vi "Step Speed Caluculation.vi"() -> ()   [LabVIEW 2025]
uses:
  controls/LAB-IQ UI Data.ctl
  HEAVE vi's/Heave Write enum.ctl
  HEAVE vi's/Heave Right enum.ctl
  SWAY vi's/Sway Write enum.ctl
  SWAY vi's/Sway Right enum.ctl
  d081153b-36ca-4bc4-8478-749476f82ba4.vi
  1202965f-721d-4349-8d61-5de826f379ef.vi
  785ec975-e53d-4ed4-be48-2cc128d7a91f.vi
  02c5850b-52e8-4ed5-91f8-6f0ad62f4994.vi
  1223eb78-e4c4-4b69-bf80-185c82055158.vi
  e5651a45-6a49-4a3f-b503-ff1eaf449b4a.vi
  support/Message Queue/Enqueue Message (Single).vi
  <vilib>/Utility/error.llb/Error Cluster From Error Code.vi
  <vilib>/Utility/file.llb/Read Delimited Spreadsheet (string).vi
  <vilib>/Utility/file.llb/Write Delimited Spreadsheet (string).vi
  <vilib>/ErrorRing/Error Ring.xnode
  support/Message Queue/LAB-IQ Message Queue.lvlib
  support/User Event - Stop/LAB-IQ User Event - Stop.lvlib
panel:
  out "error out":errorcluster
  in  "File Path :  2":path
  out "Wear Track Diameter":dbl
  in  "Stribeck table":bool
  in  "seq":bool=TRUE
  out "Drive Error":string
  out "mm/s  Surge":dbl=7.0 caption="Jog" min=0.001 max=50.0 step=0.0001 format="%.2f"
  in  "Update Surge Speed":bool
  out "mm/s  Sway":dbl=7.0 caption="Jog" min=0.001 max=50.0 step=0.0001 format="%.2f"
  in  "Update Sway Speed":bool
  in  "Update Heave Speed":bool
  out "mm/s Heave":dbl=7.0 caption="Jog" min=0.001 max=30.0 step=0.0001 format="%.2f"
  in  "mm/sec":dbl=1.0 caption="Jog" min=0.001 max=50.0 step=0.001 format="%.2f"
  out "Scratch Start Test":bool
  in  "HomeScratch":bool
  in  "TEST SELECTION":enum32{"Time", "Cycle"}(radio)
  in  "Sway Loop Delay":dbl
  in  "Sway PID Speed":dbl=1.0 format="%.4f"
  in  "Sway Jog Speed":dbl=1.0 format="%.4f"
  out "HEAVE ENABLE":bool
  in  "SPARE  5":u8
  in  "Manual Write SWAY":bool
  out "SWAY WRITE":string
  in  "SPARE  4":u8
  in  "SPARE  3":u8
  in  "SPARE 2":u8
  in  "SPARE 1":u8
  out "Spare 15":u8
  out "Spare 14":u8
  out "Spare 13":u8
  out "Spare 12":u8
  out "Spare 11":u8
  out "Spare 10":u8
  out "Spare 9":u8
  out "Spare 8":u8
  out "Spare 7":u8
  out "Spare 6":u8
  out "Spare 5":u8
  out "Spare 4":u8
  out "Spare 3":u8
  out "Spare 2":u8
  out "Spare 1":u8
  out "Node Id":u8
  out "Read SWAY Temp":bool
  out "fwMinor":u8
  out "fwMajor":u8
  out "faultCode":u16
  out "Rotary POSE":sgl format="%#.6f"
  out "SWAY POSE":sgl format="%#.6f"
  out "Homed":u8
  out "State":u8
  out "Ack ID":u16
  in  "SPEED":sgl=10000.0
  in  "Distance":sgl=10000.0
  in  "Mode Command":u8=2
  out "Sequence ID":u16
  out "error out Read SWAY":errorcluster
  out "error out Write  SWAY":errorcluster
  out "SWAY READ":string
  in  "min_finetune_floor":dbl=0.15
  in  "min_deadband_floor":dbl=0.05
  in  "fine_tune_pct":dbl=100.0
  out "Start Test Temp":bool
  in  "STOP":bool
  in  "AppLoadSeq scratch":bool
  out "Pulse delta":dbl
  in  "Fine Tune Zone":dbl=10.0
  in  "PID Delay (sec)":dbl=1.0 format="%#_6p"
  in  "Max_pos_limit":dbl=50000000.0
  in  "Min_pos_limit":dbl
  in  "i_limit":dbl=10.0
  in  "Max Step Linit":dbl=10.0
  in  "Init Step":dbl=10.0
  in  "pct_scale":dbl=100.0
  in  "Deadband":dbl=0.1
  in  "Kd":dbl
  in  "Ki":dbl
  in  "Kp":dbl=1.0
  out "Current Position":dbl
  in  "Set Load":dbl
  in  "Current Load":dbl
  in  "Manual Write Heave & Surge":bool
  out "Heave and Surge Write":string
  in  "Heave Loop Delay":dbl
  in  "Heave PID Speed":dbl=15.0
  in  "Surge Jog Speed":dbl=1.0 format="%.4f"
  in  "Heave Jog Speed":dbl=15.0
  in  "SPARE 4":u8
  in  "SPARE 3":u8
  in  "SPARE 2":u8
  in  "SPARE 1":u8
  out "Spare 15":u8
  out "Spare 14":u8
  out "Spare 13":u8
  out "Spare 12":u8
  out "Spare 11":u8
  out "Spare 10":u8
  out "Spare 9":u8
  out "Spare 8":u8
  out "Spare 7":u8
  out "Spare 6":u8
  out "Spare 5":u8
  out "Spare 4":u8
  out "Spare 3":u8
  out "Spare 2":u8
  out "Spare 1":u8
  out "Node Id":u8
  out "Read Heave Temp":bool
  out "fwMinor":u8
  out "fwMajor":u8
  out "faultCode":u16
  out "SURGE POSE":sgl format="%#.6f"
  out "HEAVE POSE":sgl format="%#.6f"
  out "Homed":u8
  out "State":u8
  out "Ack ID":u16
  in  "SPEED":sgl=10000.0
  in  "Distance":sgl=10000.0
  in  "Mode Command":u8=2
  out "Sequence ID":u16
  out "error out Read":errorcluster
  out "error out Write":errorcluster
  out "Heave and Surge Read":string
  out "Load Cell Temp":bool
  in  "Stop Scratch":bool
  in  "Enter Fixed SRR 2":dbl min=0.0 max=0.0 format="%.3f"
  in  "E.Velocity 2":bool=TRUE caption="SRR"
  in  "Tab Control 3":T1(tab)
  in  "Tab Control 5":enum32{""}(tab)
  in  "Tab Control 14":T2(tab)=enum."Motor Load"
  in  "Ramp MulFac":dbl=2.0
  in  "pulses LoadDiffRamp(2..10)":dbl=9.0
  in  "PulseControlRamp(diff<=3N)":dbl=5.0 min=1.0 max=1000.0 step=1.0 format="%#.1f"
  in  "SetLoadDeadband(%) Load(0-10N)":dbl=0.1 min=0.0001 max=100.0 step=0.0001 format="%#.6f"
  in  "PID gains out delay (microForce)":T3={"proportional gain (Kc)"=300.0, "integral time (Ti, min)"=0.00011, "derivative time (Td, min)"=0.0} {"derivative time (Td, min)" format="%.3f"; "integral time (Ti, min)" min=1e-05 max=100.0 step=1e-06 format="%.6f"; "proportional gain (Kc)" format="%.3f"}
  in  "Ramp":bool
  in  "Gain 2":dbl=0.016
  in  "pulses LoadDiff(2..10)":dbl=10.0
  in  "pulses LoadDiff(11..50)":dbl=40.0
  in  "PulseControl(diff<=3N)":dbl=1.0 min=1.0 max=1000.0 step=1.0 format="%#.1f"
  out "SetLoadDeadband(%)  2":dbl=1.0 min=0.001 max=100.0 step=0.001 format="%#.6f"
  in  "Dummy Run":bool
  out "Vertical load (N)":dbl format="%#.3f"
  in  "AutoTune":bool
  in  "Offset  3":dbl=1.5
  in  "apply load":bool
  in  "Enter ByPass Load":dbl
  in  "reinit 3":bool=TRUE
  in  "output range delay":cluster{"output high":dbl, "output low":dbl}={"output high"=100.0, "output low"=-100.0} {"output low" format="%.2f"; "output high" format="%.2f"}
  in  "PID gains out delay":T3={"proportional gain (Kc)"=30.0, "integral time (Ti, min)"=0.00101, "derivative time (Td, min)"=0.0} {"derivative time (Td, min)" format="%.3f"; "integral time (Ti, min)" min=1e-05 max=100.0 step=0.0001 format="%.4f"; "proportional gain (Kc)" format="%.3f"}
  in  "Bypass Load":bool
  in  "pulsesSent":dbl=200.0
  out "pulses":dbl
  out "actpid":dbl
  out "gFF Rot 7":cluster{dbl, dbl, dbl}(graph)
  in  "pulses LoadDiff(21..1000)":dbl=40.0
  in  "Delay":dbl=1.5 min=0.001 max=5.0 step=0.001 format="%#.6f"
  in  "deadband":dbl=0.2
  in  "Tab Control 26":enum32{"Page 1", "Page 2"}(tab)
  in  "ClearAll":bool
  out "Mz(Nm)":dbl[](array[numeric])
  out "My(Nm)":dbl[](array[numeric])
  out "Mx(Nm)":dbl[](array[numeric])
  in  "Save Dwell":dbl=0.015 caption="Save Dwell (sec)" min=0.0 max=5.0 step=0.001 format="%.3f"
  out "Mx":dbl[](graph)
  out "My":dbl[](graph)
  out "Mz":dbl[](graph)
  out "Fy(N)":dbl[](graph)
  out "Fz(N)":dbl[](graph)
  in  "ZeroAll":bool
  in  "Acq Delay (ms)":dbl=10.0
  in  "Burst Delay (ms)":dbl=10.0
  out "model":string
  out "SN":i32
  out "FFx(N)":dbl[](array[numeric])
  in  "Sensor IP":string="192.168.1.100"
  in  "Port":i32=8080
  out "FFy(N)":dbl[](array[numeric])
  out "Load(N)":dbl[](array[numeric])
  out "Fx(N)":dbl[](graph)
  out "AE":bool
  in  "delete Handle":bool
  in  "Create Handle":bool=TRUE
  out "ft_data":dbl[](array[numeric])=[1.0, 1.0, 1.0, 1.0, 1.0, 1.0]
  out "ft_range":dbl[](array[numeric])=[1.0, 1.0, 1.0, 1.0, 1.0, 1.0]
  in  "stop 6":bool
  out "running_flag":bool
  out "ft_udp_handle":i32
  out "get-data-return":i32
  out "get-range-return":i32
  out "zero-return":i32
  out "filter-return":i32
  out "initial-return":i32
  out "deleteHandle-result":i32
  in  "Tab Control 19":enum32{"Platform COM", "Config ", "DevInfo"}(tab)=enum."Config "
  in  "SAMPLES":dbl=100.0
  in  "Re-initilaize":bool
  in  "Filter ON/OFF":bool=TRUE
  in  "TracHomeSurgeOffsetCounts 10MM":dbl=505100.0
  in  "TracHomeSwayOffsetCounts 10MM":dbl=1432.0
  in  "Acoustic Emission:":dbl=1.0 min=0.0001 max=200.0 step=0.0001 format="%.4f"
  in  "Apply Filter (FF)":bool
  in  "Filter% 2":dbl=50.0 min=50.0 max=100.0 step=0.1 format="%.1f"
  in  "Apply Filter (Load)":bool=TRUE
  in  "Filter%":dbl=80.0 min=50.0 max=100.0 step=0.1 format="%.1f"
  in  "Sway distance (mm)":dbl=245.0
  in  "Surge distance (mm)":dbl=370.0
  in  "DataSavingLoopDelay(ms)":dbl=15.0
  in  "SAVE  2":bool
  in  "Enter Distance":bool caption="Enter Counts"
  in  "Sway Counts:":dbl=100.0 min=0.0 max=100000000.0 step=1.0 format="%.2f"
  in  "Distance (mm): 3":dbl=100.0 caption="Distance (mm):" min=0.0 max=1500.0 step=0.001 format="%.5f"
  in  "Surge Counts:":dbl=100.0 min=0.0 max=100000000.0 step=1.0 format="%.1f"
  in  "Distance (mm): 2":dbl=100.0 caption="Distance (mm):" min=0.0 max=1500.0 step=0.0001 format="%.3f"
  in  "Distance (mm):":dbl=100.0 min=0.0 max=1500.0 step=0.001 format="%.5f"
  in  "Heave Counts:":dbl=100.0 min=0.0 max=100000000.0 step=1.0
  in  "LRMHomeSurgeOffsetCounts":dbl=307197.0
  in  "LRMHomeSwayOffsetCounts":dbl=26880.0
  in  "TracHomeSurgeOffsetCounts 20MM":dbl=505100.0
  in  "TracHomeSwayOffsetCounts 20MM":dbl=1432.0
  in  "RotHomeSwayOffsetCounts":dbl=14656.0
  in  "RotHomeSurgeOffsetCounts":dbl=311465.0
  in  "Heave distance":dbl=340.0
  out "Zmm":dbl=1600.0
  out "Heave Pulses/mm":dbl=1600.0
  out "Surge Pulses/mm":dbl=1600.0
  out "Sway Pulses/mm":dbl=320.0
  in  "Heave Pitch":dbl=4.0
  in  "Surge Pitch":dbl=3.0
  in  "Sway Pitch":dbl=2.0
  in  "Heave PPR":dbl=6400.0
  in  "Surge PPR":dbl=6400.0
  in  "Sway PPR":dbl=6400.0
  in  "GUI":T4(tab)
  in  "Platform Settings":bool caption="Password"
  in  "Configure":bool caption="Password"
  in  "Home":bool caption="Password"
  in  "EXIT":bool
  in  "Analysis":bool caption="Password"
  in  "service 2":bool caption="Password"
  in  "MainPage":T5(tab)=enum."HOME"
  in  "Select Load Head":bool
  in  "Notes :":string
  in  "FILE":string
  in  "Sample ID :":string
  in  "Operator ID :":string
  in  "Operator Name :":string
  in  "Auto":bool caption="Power Status"
  in  "Disable Axis Jog Soft Limits":bool
  out "Sway and Surge COM Status":bool=TRUE caption="Load COM Status"
  out "Heave COM Status":bool=TRUE caption="Load COM Status"
  in  "Enable Platform":bool
  in  "Surge Forward Main":bool
  in  "Surge Backward Main":bool
  in  "Sway Right Main":bool
  in  "Sway Left Main":bool
  in  "Heave Down Main":bool
  in  "Heave Up main":bool
  in  "mm":dbl=0.001 caption="Jog" min=0.001 max=200.0 step=0.0001 format="%#.3f"
  in  "Surface Analysis":bool
  in  "Imaging":bool
  in  "Image Analysis":bool
  in  "Post Analysis":bool
  in  "SSP 0.75":bool
  in  "SSP 0.5":bool
  in  "SSP 0.3":bool
  in  "Warning":enum32{"Page 2"}(tab)
  in  "gui GIF":enum32{"Check", "Deca", "kilo", "Micro"}(tab)
  out "Communication is established":bool=TRUE caption="Load COM Status"
  in  "Reference Sample":u16(ring) items=["None", "Brass", "Aluminium", "Mild Steel"]
  out "Load Cell Communication Slide":u8(slide)=1 min=1 max=10 step=1 scale=0.0..10.0
  in  "com 3":bool
  out "com":bool
  out "DecaForce COM Status":bool caption="Load COM Status"
  in  "Loading Mode":u16(ring) items=["Constant", "Ramp", "Steps", "Indentation"]
  in  "Enter the CoF Trip":dbl=1.0
  in  "Enter the Friction Force Trip":dbl=520.0 min=500.0 max=500.0 step=1.0 format="%#.1f"
  in  "Enter the Normal load Trip":dbl=520.0 min=500.0 max=500.0 step=0.001 format="%.3f"
  in  "KiloForce":bool
  in  "DecaForce":bool
  in  "MicroForce":bool
  in  "LHBack":bool
  in  "LHNext":bool
  in  "Load Selection":T6(tab)
  in  "Enter the Load  (N)":dbl=2.0 caption="Enter the Load (N)" min=200.0 max=500.0 step=0.1 format="%#.4f"
  in  "Enter the Final Load (N)":dbl=1.0 min=0.0 max=500.0 step=1.0 format="%#.0f"
  in  "Update":bool
  in  "Enter the Loading Rate (N/min)":dbl=60.0 min=1.0 max=1200.0 step=0.1 format="%.2f"
  out "Warning 2":bool
  in  "Stribeck Table  For loading":string[][](table)
  in  "Clear 3":bool
  out "Message":string="Load Entered is out of range!!!"
  in  "Indentation":string[][](table)=[["Detection", "5", "2"], ["Unload", "0", "5"], ["Load", "10", "2"], ["Unload", "0", "5"], ["Detection", "5", "2"], ["Unload", "0", "5"]]
  in  "Multipoint":bool caption="Singlepoint"
  in  "AppLoad 4":bool
  in  "zNL":bool
  out "NL disp":dbl caption="Normal Load ( N )" min=-2000.0 max=2000.0 step=0.0001 format="%.1f"
  in  "Traction":bool
  in  "Surge Forward MM":bool
  in  "Surge Backward MM":bool
  in  "M3 Image":enum32{"Page 1", "Page 2"}(tab)
  in  "String 39":string="Jog heave to bring the upper sample closer to the lower sample within 1mm."
  in  "Sway Left MM":bool
  in  "Sway Right MM":bool
  in  "Disable Axis Jog Soft Limits":bool
  in  "mm":dbl=0.001 caption="Jog" min=0.001 max=5.0 step=0.0001 format="%#.3f"
  in  "Heave Down MM":bool
  in  "Heave Up MM":bool
  in  "Wear Track Diameter (mm)":dbl=30.0 caption="Wear Track Diameter (mm):" min=1.0 max=30.0 step=1.0 format="%.2f"
  in  "Set WTD":bool
  in  "HomeScratch":bool
  in  "HomeRot":bool
  in  "PlaceModule":bool
  in  "Motion Mode:":u16(ring) items=["Uniform Rotation", "Angular Oscillation", "Stribeck ", "Steps"]
  in  "LR Sway":bool
  in  "Rot Hor":bool
  in  "Rot Ver":bool
  in  "Scratch":bool
  in  "LR Cam":bool
  in  "MMBack":bool
  in  "MMNext":bool
  in  "Rotary Module Selection":T7(tab)
  in  "SPEED SELECTION :":enum32{"Speed in RPM", "Speed in m/sec"}(radio)=enum."Speed in m/sec"
  in  "Enter the Speed(mm/sec)":dbl=0.1 min=0.1 max=10.0 step=0.1 format="%.3f"
  in  "Enter the Speed (RPM)":dbl=45.0 min=1.0 max=3000.0 step=1.0
  in  "Enter the Frequency (Hz)":dbl=1.0 min=0.1 max=10.0 step=0.1 format="%.1f"
  in  "Enter the Angle (Deg)":dbl=45.0 min=5.0 max=300.0 step=1.0
  in  "Angular Oscillation Set":bool
  in  "Rotary Tab":enum32{"Page 1", "Page 2"}(tab)
  out "e.v/ssr 2":enum32{"E.V", "SSR"}(tab)
  in  "Enter the Final E.Velocity (m/s) 2":dbl=1.0 min=0.001 max=4.0 step=0.001 format="%.3f"
  in  "Enter initial E.Velocity (m/s) 2":dbl=2.0 min=0.001 max=4.0 step=0.001 format="%.3f"
  in  "Enter Fixed E.Velocity 2":dbl=1.0 min=0.001 max=2.0 step=0.001 format="%.3f"
  in  "Enter Final SRR 2":dbl=1.0 min=0.001 max=1.0 step=0.001 format="%.2f"
  in  "Enter initial SRR 2":dbl=1.0 min=0.001 max=1.0 step=0.001 format="%.2f"
  out "Final Speed (RPM) 3":dbl=1.0 min=0.1 max=3000.0 step=0.1 format="%.1f"
  out "Initial Speed (RPM) 2":dbl=100.0 min=0.1 max=3000.0 step=0.1 format="%.1f"
  in  "Enter the Final Velocity (m/s) 3":dbl=1.0 min=0.001 max=2.0 step=0.001 format="%.3f"
  in  "Enter initial Velocity (m/s)  3":dbl=2.0 min=0.001 max=2.0 step=0.001 format="%.3f"
  out "Ramp Up 2":bool caption="Ramp Down"
  in  "Import 2":bool
  in  "Save 2":bool
  in  "SPEED SELECTION : rotary":enum32{"Speed in Rpm", "Speed in m/sec"}(radio)=enum."Speed in m/sec"
  in  "calculate rotary":bool
  in  "String 45":string="File Path Location : C:-->LAB-IQ 150 --> User Defined\n                                       Protocol-->File.txt"
  in  "Step Speed":enum32{"Step Speed", "Step (load-Speed)"}(tab)
  in  "StepTable For Speed":string[][](table)
  in  "StepTable For Load-Speed":string[][](table)=[["", "", ""], ["", "", ""], ["", "", ""], ["", "", ""]]
  in  "StepTable For Speed 3":string[][](table)=[["", "", ""], ["", "", ""], ["", "", ""], ["", "", ""]]
  in  "Motion Direction:  3":u16(ring) items=["Clockwise", "Counter Clockwise"]
  in  "Enter Scratch length (mm):":dbl=1.0 min=1.0 max=50.0 step=0.0001 format="%.4f"
  in  "Enter Scratch Speed (mm/s):":dbl=1.0 min=0.003 max=10.0 step=0.0031 format="%.5f"
  in  "SwaySpeed Set":bool
  in  "Scartch Offset":dbl=1.0 caption="Scratch Offset: (mm)" min=0.1 max=5.0 step=0.1 format="%.1f"
  in  "Motion type:":u16(ring) items=["Unidirection", "Bidirection"]
  in  "Scratch Mode:":u16(ring) items=["Scratch", "Pre-Post Scan", "Multi Pass"]
  in  "Rotary Speed Exced":string="Motor Speed Out of Range"
  out "Humidity  Status  3":bool caption="Communication Status"
  out "Low Temp  Status  2":bool=TRUE caption="Communication Status"
  out "TK4 status 2":bool=TRUE caption="Communication Status"
  in  "String 40":string="Before selecting Acoustic make sure the sensor output pin is connected to A4."
  in  "Stage Temperature":dbl[](array[numeric])=[150.0, 230.0, 300.0, 350.0, 400.0, 450.0, 500.0]
  in  "Sample Temperature":dbl[](array[numeric])=[100.0, 150.0, 200.0, 250.0, 300.0, 350.0, 400.0]
  in  "Humidity (Amb)":bool
  in  "Clear List":bool
  out "Sensors Picked":string
  in  "Add to list":bool
  in  "Wear":bool
  in  "Vibration":bool
  in  "Humidity (Chamber)":bool
  in  "Temperature (Chamber)":bool
  in  "ECR":bool
  in  "Temperature (Amb)":bool
  in  "Microphone":bool
  in  "Acoustic Emission 3":bool
  in  "SNext":bool
  in  "APBack":bool
  in  "Enter the Temperature (°C):":dbl
  in  "Enter the Stage \nTemperature (°C):":dbl=20.0 min=20.0 max=150.0 step=1.0 format="%#.0f"
  in  "Enter the Humidity (%Rh):":dbl=30.0 min=30.0 max=85.0 step=1.0
  in  "Low Temp":bool
  in  "High Temp":bool
  in  "Humidity":bool
  in  "Main Screen Tab":T8(tab)
  in  "ClrLog":bool
  out "Trip Log":string
  in  "Start Test":bool
  out "Test status":bool caption="Test Status"
  out "AR Led":bool caption="AR"
  out "Data":bool=TRUE
  out "Health":bool=TRUE
  out "Sway COM Status":bool=TRUE caption="Load COM Status"
  out "Heave COM Status":bool=TRUE caption="Load COM Status"
  in  "Grp Tab":enum32{"Rot/LRM", "FBT"}(tab)
  in  "Sub Graph":T9(tab)
  in  "Speed Reset Graph":bool
  in  "Speed Tab":enum32{" Rotary Disc", "MTM Ball", "MTM Disc"}(tab)
  out "speed mm/sec":dbl(graph)=0.13298760003255525
  out "MTM BALL SPEED":dbl(graph)=0.13298760003255525
  out "MTM DISC  SPEED":dbl(graph)=0.13298760003255525
  in  "Temperature Reset":bool
  out "Temperature (deg c)":dbl(graph)=0.13298760003255525
  in  "ECR RESET":bool
  out "ECR":dbl(graph)=0.13298760003255525
  out "Acoustic Emission (mV)":dbl min=0.0 max=5000.0 step=0.1
  in  "Aqucostic Reset Graph":bool
  out "gACQUOS":dbl(graph)=0.13298760003255525
  in  "Humidity Reset Graph":bool
  out "HumrGp":dbl(graph)=0.13298760003255525
  out "SD (mm)":dbl caption="Sliding Distance ( mm )" min=-200.0 max=200.0 step=0.1 format="%.4f"
  in  "Siliding distance Reset Graph":bool
  out "SDGp":dbl(graph)=0.13298760003255525
  out "Hymidity":bool
  in  "Humidity Disable trip":bool=TRUE
  in  "CoF Trip  2":dbl=540.0 min=100.0 max=540.0 step=1.0
  out "Depth Trip":dbl=600.0
  in  "Depth Trip":bool=TRUE
  out "Weart Deapth":bool
  in  "Depth Reset Graph":bool
  out "Weart":bool
  in  "Depthz":bool
  out "Depth (µm)":dbl min=-200.0 max=200.0 step=0.1 format="%.1f"
  out "WearGp":dbl(graph)=0.13298760003255525
  out "NL Trip 2":dbl=600.0
  out "Load pid":bool
  in  "Load Disable Trip":bool=TRUE
  in  "Load Reset Graph":bool
  out "NL Display 4":dbl caption="Normal Load ( N )" min=-2000.0 max=2000.0 step=0.0001 format="%.1f"
  out "Main Chart 3":cluster{dbl, "NL disp":dbl, dbl}(graph)
  in  "FF Tab":T10(tab)
  in  "COF Reset Graph":bool
  in  "COF Disable Trip":bool=TRUE
  out "COF TRIP":dbl=600.0
  out "Coefficient of Friction":dbl(graph)=0.13298760003255525
  in  "zFF":bool
  in  "FF Reset Graph":bool
  in  "FF Disable Trip":bool=TRUE
  out "FF TRIP":dbl=600.0
  out "Friction Force (N)":dbl min=-2000.0 max=2000.0 step=0.0001 format="%.3f"
  out "Friction Force (N) Graph":dbl(graph)=0.13298760003255525
  out "Cyclic FF TRIP":dbl=600.0
  in  "Cyclic FF Disable Trip":bool=TRUE
  in  "Cyclic FF Reset Graph":bool
  in  "CZ FF":bool
  out "Cyclic Friction Force (N) Graph":dbl(graph)=0.13298760003255525
  out "Cyclic Friction Force (N)":dbl min=-2000.0 max=2000.0 step=0.0001 format="%.3f"
  out "cyclic COF TRIP":dbl=600.0
  in  "cyclic COF Disable Trip":bool=TRUE
  in  "cyclic COF Reset Graph":bool
  out "Cyclic Coefficient of Friction":dbl(graph)=0.13298760003255525
  in  "BACK":bool
  out "Ambient \nTemperature":dbl min=0.0 max=5000.0 step=0.1 format="%.1f"
  out "Ambient\n Humidity":dbl min=0.0 max=5000.0 step=0.1 format="%.2f"
  out "NL disp 2":dbl caption="Normal Load ( N )" min=-2000.0 max=2000.0 step=0.0001 format="%.1f"
  out "Set Humidity":dbl caption="Set Humidity  (% Rh)" min=-2000.0 max=2000.0 step=1.0 format="%.1f"
  out "humidity disp":dbl caption="Humidity (% Rh)" min=-2000.0 max=2000.0 step=1.0 format="%.1f"
  in  "Humidity On":bool
  in  "zNL 2":bool
  out "NLt":bool
  in  "Load En":bool
  out "Freq (Hz)":dbl min=0.0 max=5000.0 step=0.1 format="%.4f"
  out "HumCOMStatus":bool caption="Communication Status"
  out "Load Communication":bool
  in  "Temp Tabs":enum32{"Low Temp", "High Temp"}(tab)=enum."High Temp"
  out "Controller  Status":bool
  out "ChamberTemp":dbl format="%#.1f"
  in  "SetTmp":dbl=-190.0 caption="Set Temperature (Deg C)" min=-190.0 max=100.0 step=1.0 format="%.1f"
  in  "Cooling":bool
  in  "Heater":bool
  out "TK4 status":bool caption="Controller  Status"
  out "ChamberTemp":dbl format="%#.1f"
  in  "SetTmp":dbl caption="Set Temperature (Deg C)" min=0.0 max=1000.0 step=1.0 format="%.1f"
  in  "Set Load (N)":dbl=100.0 min=0.01 max=1500.0 step=0.01 format="%.1f"
  in  "Time Tab":enum32{"cycles", "duration"}(tab)=enum."duration"
  out "Test Duration 4":dbl=600.0 caption="Test Duration\n(HH:MM:SS)" min=0.0083 max=180000.0 step=0.0001 format="%<%H:%M:%S>t"
  out "TEST CYCLE":dbl min=0.0 max=5000.0 step=0.01 format="%.2f"
  in  "TOTAL CYCLES":dbl min=0.0 max=5000.0 step=0.1 format="%.4f"
  out "Time ( HH:MM:SS ) 2":dbl min=0.0 max=144000.0 step=1.0 format="%<%H:%M:%S>t"
  in  "Test Duration":dbl=600.0 caption="Test Duration\n(HH:MM:SS)" min=0.0083 max=180000.0 step=0.0001 format="%<%H:%M:%S>t"
  in  "Main Speed Tab":enum32{"ROTARY", "TRACTION"}(tab)
  in  "SPEED TAB":enum32{"RPM", "m/sec"}(tab)
  out "Speed (RPM)":dbl min=0.0 max=5000.0 step=0.1 format="%.1f"
  out "Set Speed":dbl caption="Set Speed (RPM)" min=0.0 max=1500.0 step=0.1 format="%.1f"
  out "Speed (m/sec)":dbl min=0.0 max=5000.0 step=0.001 format="%.4f"
  out "Set Speed (m/sec)":dbl min=0.0 max=1500.0 step=0.001 format="%.4f"
  in  "MTM MOTOR DISPLAY":enum32{"MTM RPM", "MTM m/sec"}(tab)
  out "Disc Speed (RPM)":dbl min=0.0 max=1500.0 step=0.1 format="%.1f"
  out "Ball Speed (RPM)":dbl min=0.0 max=1500.0 step=0.1 format="%.1f"
  out "Disc Speed (m/sec)":dbl min=0.0 max=1500.0 step=0.1 format="%.1f"
  out "Ball Speed (m/sec)":dbl min=0.0 max=1500.0 step=0.1 format="%.1f"
  in  "Angle and Frequency":enum32{"angular", "lrm"}(tab)
  out "Angle (Deg)":dbl min=0.0 max=5000.0 step=0.01 format="%.2f"
  out "Stroke (mm)":dbl min=0.0 max=5000.0 step=0.01 format="%.2f"
  in  "Analysis Home":bool
  in  "Password":string
  in  "Home Service":bool
  in  "Advanced Setting":bool
  in  "About Tab":enum32{"Primary"}(tab)
  in  "ECR Port:":refnum<visa-resource-name>="COM10"
  in  "Ramp Port:":refnum<visa-resource-name>="COM10"
  in  "Installation/Replacement completed":bool
  in  "Loahead":bool
  in  "Heave and Surge COM Port:":refnum<visa-resource-name>="COM9"
  in  "Sway COM Port:":refnum<visa-resource-name>="COM10"
  in  "Temp Modbus:":refnum<visa-resource-name>="COM14"
  in  "Humidity Port:":refnum<visa-resource-name>="COM10"
  in  "Edit Gain Constants":bool
  in  "Save Gain Constants":bool
  in  "Service About":bool
  # "SET JOG SPEED"
  # "Speed Exceed the limit of the Motor"
  # "Motor Speed Out of Range"
  # "load Aquisition off"
  # "load Aquisition On"
  # "Configuration"
  # "Limits for Heave Surge and Sway"
  # "Modules Offset Parameters"
  # "Counts-Distance Calculator"
  # "File Name :"
  # "Ensure the traction module is aligned\n horizontally with the stage before ENABLE."
  # "JOG MODE"
  # "Module Selection"
  # "Positioning Control"
  # "Connect the controller\ncable to M3"
  # "Environment"
  # "Sensors"
  # "Data Points"
  # "Data Points"
  # "Data Points"
  # "Data Points"
  # "ohms"
  # "Data Points"
  # "Data Points"
  # "Data Points"
  # "LAB-IQ 150 / UNITEST / WO2456 / UT150  v05 / AUGUST 2025"
  # "NOTE: This operation needs to be done only when the machine is ON."
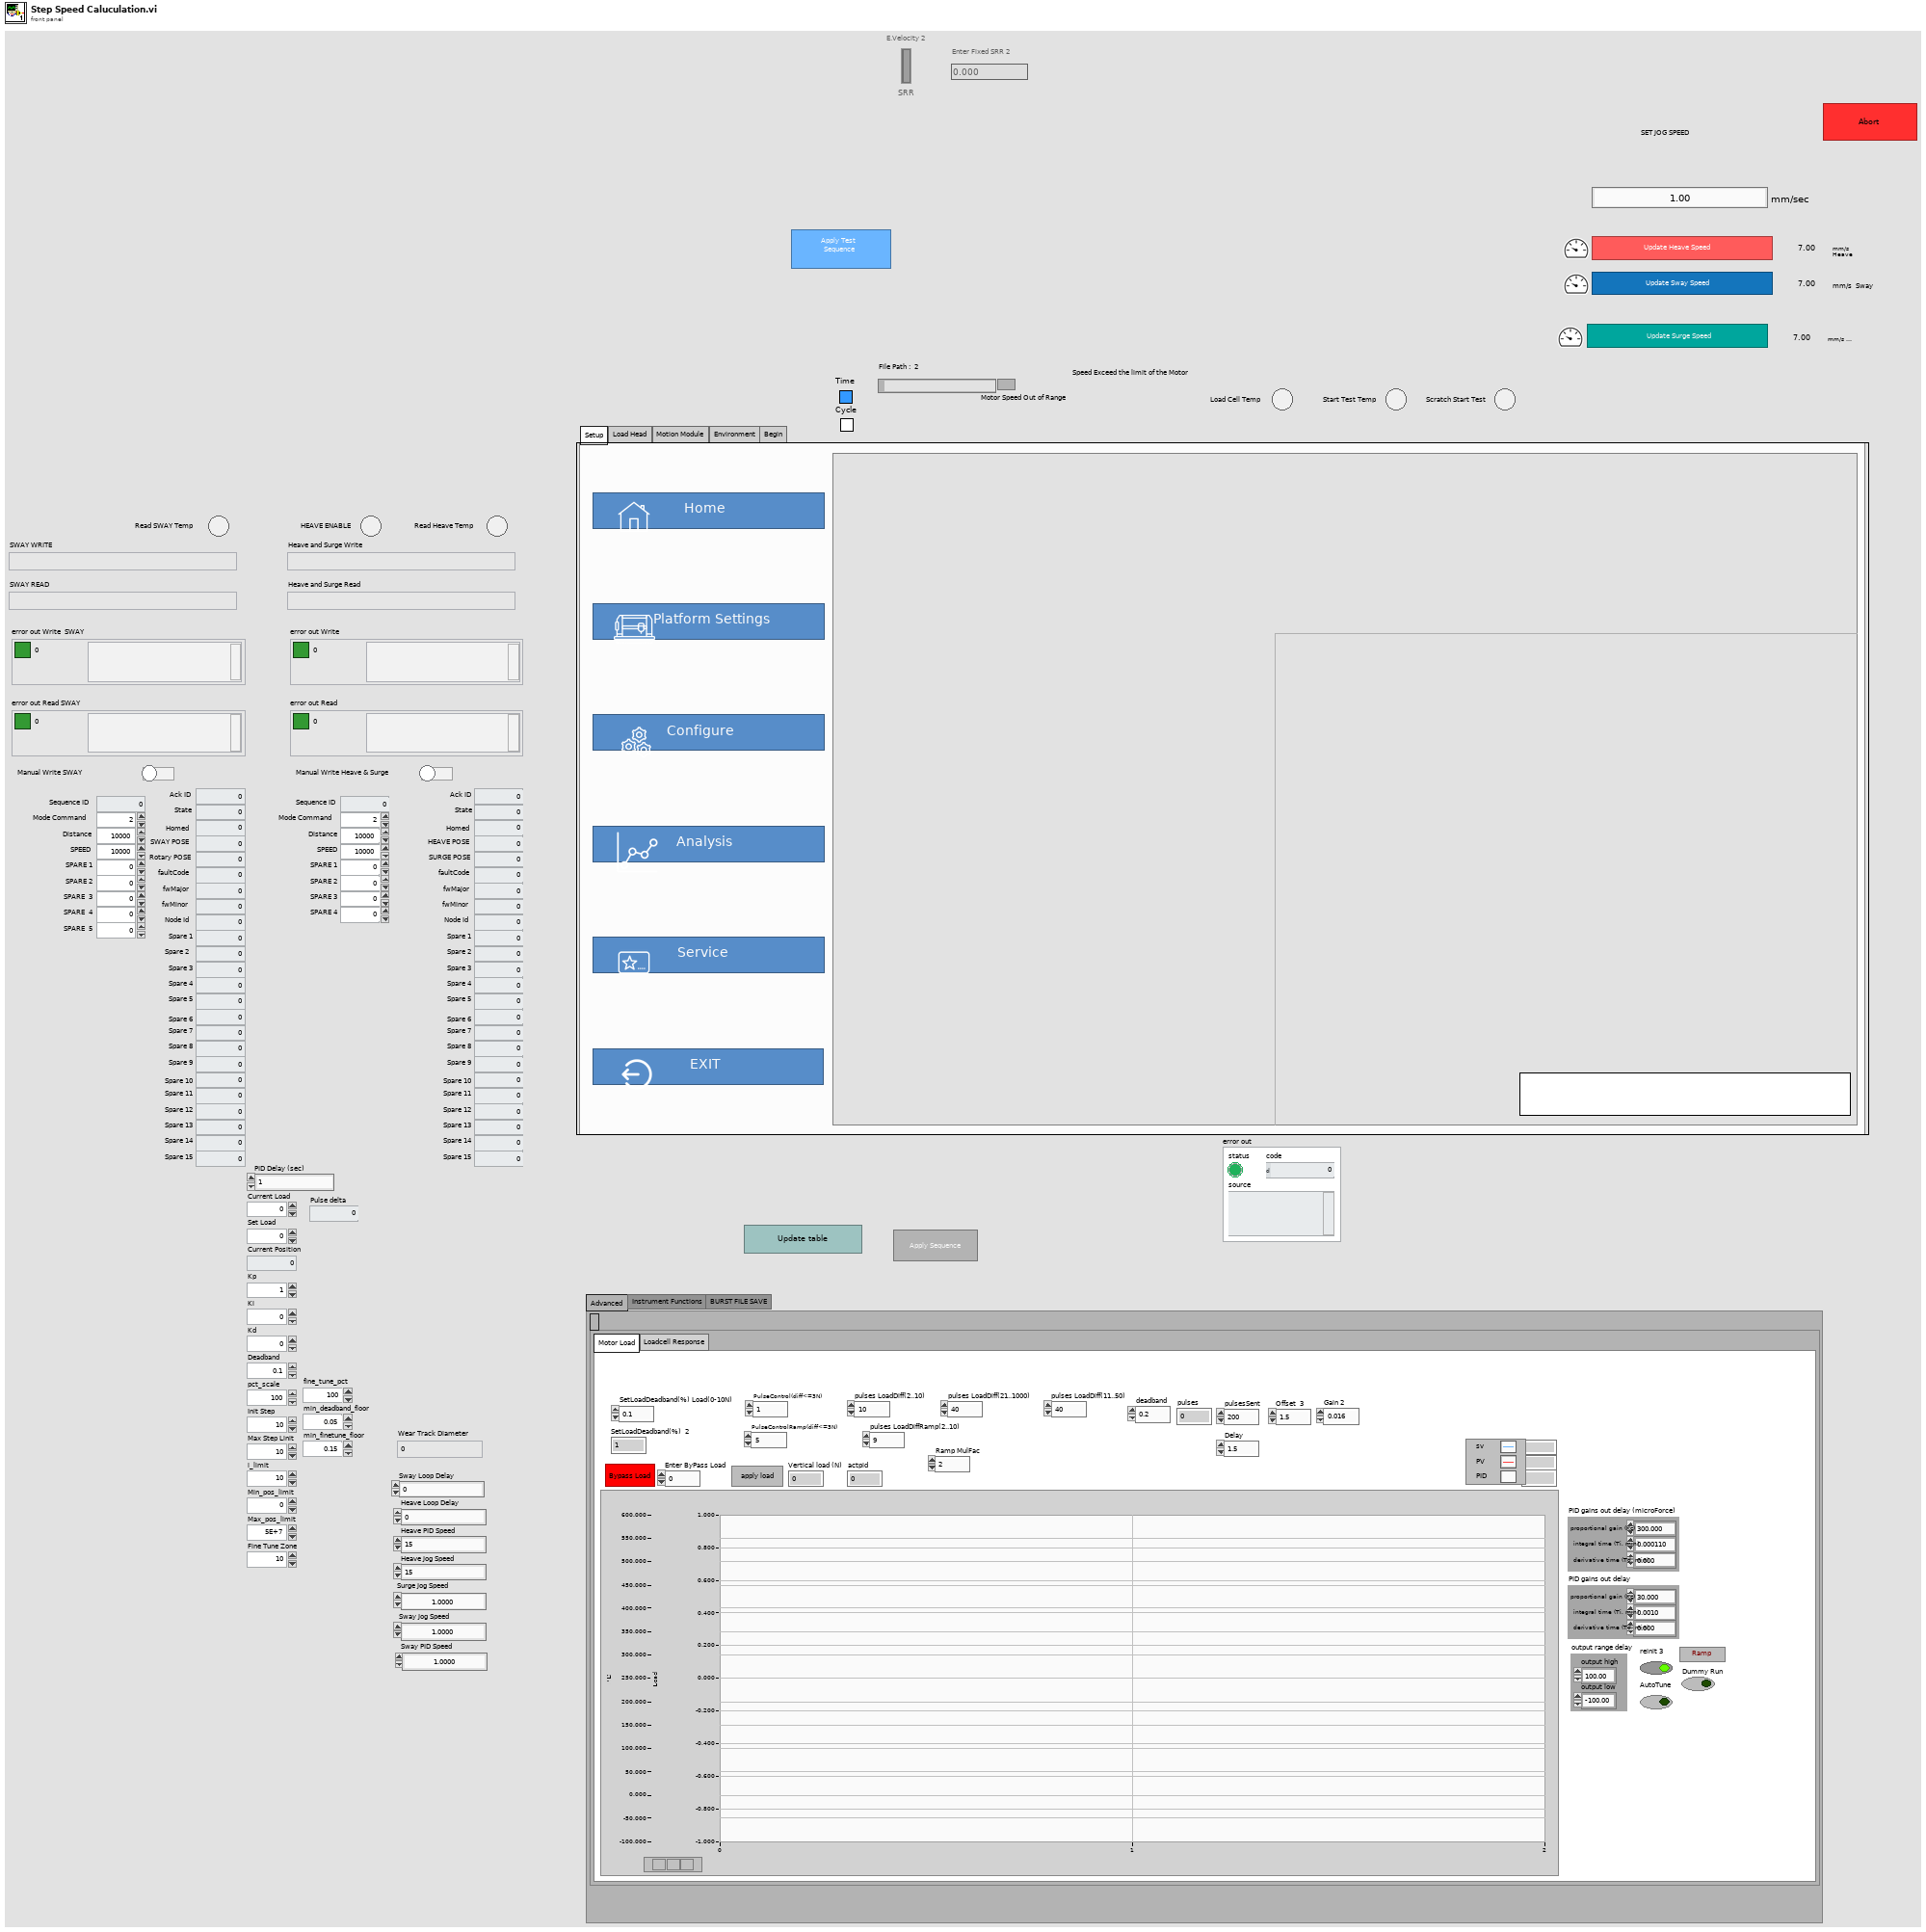
[diagram p1: front panel]
types:
  T1 = enum32{"Advanced", "Motor", "Depth_graph", "UIO Communicator", "Add to list parametrs", "Instrument Functions", "BURST FILE SAVE"}
  T2 = enum32{"LRM heating", "FBT_Heating", "Motor Load", "Loadcell Response", "Voice Load", "Step loading and speed ", "Depth"}
  T3 = cluster{"proportional gain (Kc)":dbl, "integral time (Ti, min)":dbl, "derivative time (Td, min)":dbl}
  T4 = enum32{"Setup", "Load Head", "Motion Module", "Environment", "Begin"}
  T5 = enum32{"Details", "PlatformSetting", "Analysis", "HOME"}
  T6 = enum32{"Constant", "Ramp", "Step", "Indentation"}
  T7 = enum32{"Uniform Rotation", "Angular Oscillation", "Speed Ramp", "Speed Step"}
  T8 = enum32{"  Acquire  ", "Compare Files Rot", "About", "Service"}
  T9 = enum32{"Speed", "Temperature", "ECR", "Acoustic Emission", "Humidity", "Sliding Distance"}
  T10 = enum32{"Coefficient of Friction ", "Friction Force (N)", "Cyclic Friction Force (N)", "Cyclic Coefficient of Friction "}
  T11 = typedef "LAB-IQ UI Data.ctl" = cluster{"Main Home Screen":cluster{"GUI":refnum<vi>, "Platform Settings":refnum<vi>, "Configure":refnum<vi>, "Home":refnum<vi>, "EXIT":refnum<vi>, "service 2":refnum<vi>, "MainPage":refnum<vi>, "Analysis":refnum<vi>}, "Platform Settings":cluster{"mm/s  Surge":refnum<vi>, "Update Surge Speed":refnum<vi>, "Drive Error":refnum<vi>, "Disable Axis Jog Soft Limits":refnum<vi>, "mm/s  Sway":refnum<vi>, "Sway and Surge COM Status":refnum<vi>, "Heave COM Status":refnum<vi>, "Enable Platform":refnum<vi>, "Surge Forward Main":refnum<vi>, "Sway Right Main":refnum<vi>, "Sway Left Main":refnum<vi>, "Heave Down Main":refnum<vi>, "Heave Up main":refnum<vi>, "Update Sway Speed":refnum<vi>, "Update Heave Speed":refnum<vi>, "mm/s Heave":refnum<vi>, "mm/sec":refnum<vi>, "mm":refnum<vi>, "Surge Backward Main":refnum<vi>}, "Analysis Screen":cluster{"Analysis Home":refnum<vi>, "Surface Analysis":refnum<vi>, "Imaging":refnum<vi>, "Image Analysis":refnum<vi>, "Post Analysis":refnum<vi>}, "Config Screen":cluster{"Select Load Head":refnum<vi>, "Notes :":refnum<vi>, "FILE":refnum<vi>, "Sample ID :":refnum<vi>, "Operator ID :":refnum<vi>, "Operator Name :":refnum<vi>, "Auto":refnum<vi>}, "Motion Module":cluster{"zNL":refnum<vi>, "NL disp":refnum<vi>, "Rotary Tab":refnum<vi>, "Motion Direction:  3":refnum<vi>, "E.Velocity 2":refnum<vi>, "e.v/ssr 2":refnum<vi>, "Enter Fixed E.Velocity 2":refnum<vi>, "Enter Final SRR 2":refnum<vi>, "Enter initial SRR 2":refnum<vi>, "Enter Fixed SRR 2":refnum<vi>, "Enter the Final E.Velocity (m/s) 2":refnum<vi>, "Enter initial E.Velocity (m/s) 2":refnum<vi>, "Final Speed (RPM) 3":refnum<vi>, "Initial Speed (RPM) 2":refnum<vi>, "Enter the Final Velocity (m/s) 3":refnum<vi>, "Enter initial Velocity (m/s)  3":refnum<vi>, "Ramp Up 2":refnum<vi>, "TEST SELECTION":refnum<vi>, "SPEED SELECTION : ":refnum<vi>, "Angular Oscillation Set":refnum<vi>, "Traction":refnum<vi>, "Step Speed":refnum<vi>, "StepTable For Load-Speed":refnum<vi>, "StepTable For Speed":refnum<vi>, "Surge Forward MM":refnum<vi>, "Surge Backward MM":refnum<vi>, "M3 Image":refnum<vi>, "String 39":refnum<vi>, "Sway Left MM":refnum<vi>, "Sway Right MM":refnum<vi>, "Disable Axis Jog Soft Limits":refnum<vi>, "mm":refnum<vi>, "Heave Down MM":refnum<vi>, "Heave Up MM":refnum<vi>, "Wear Track Diameter (mm)":refnum<vi>, "Set WTD":refnum<vi>, "HomeScratch":refnum<vi>, "HomeRot":refnum<vi>, "PlaceModule":refnum<vi>, "Enter the Angle (Deg)":refnum<vi>, "Enter the Frequency (Hz)":refnum<vi>, "Motion Mode:":refnum<vi>, "LR Sway":refnum<vi>, "Rot Hor":refnum<vi>, "Scratch":refnum<vi>, "LR Cam":refnum<vi>, "MMBack":refnum<vi>, "MMNext":refnum<vi>, "Rot Ver":refnum<vi>, "Rotary Module Selection":refnum<vi>, "calculate rotary":refnum<vi>, "SPEED SELECTION : rotary":refnum<vi>, "Import 2":refnum<vi>, "Save 2":refnum<vi>, "File Path :  2":refnum<vi>, "String 45":refnum<vi>, "StepTable For Speed 3":refnum<vi>, "Enter the Speed(mm/sec)":refnum<vi>, "Enter the Speed(RPM)":refnum<vi>, "Enter Scratch Speed (mm/s):":refnum<vi>, "SwaySpeed Set":refnum<vi>, "Scartch Offset":refnum<vi>, "Scratch Mode:":refnum<vi>, "Motion type:":refnum<vi>, "HomeScratch 2":refnum<vi>, "Enter Scratch length (mm):":refnum<vi>, "Wear Track Diameter":refnum<vi>, "Rotary Speed Exced":refnum<vi>}, "Environmental control":cluster{"Humidity  Status  3":refnum<vi>, "Low Temp  Status  2":refnum<vi>, "TK4 status 2":refnum<vi>, "Stage Temperature":refnum<vi>, "Sample Temperature":refnum<vi>, "Humidity (Amb)":refnum<vi>, "Clear List":refnum<vi>, "Add to list":refnum<vi>, "Wear":refnum<vi>, "Vibration":refnum<vi>, "Humidity (Chamber)":refnum<vi>, "Temperature (Chamber)":refnum<vi>, "ECR ":refnum<vi>, "Temperature (Amb)":refnum<vi>, "Microphone":refnum<vi>, "Acoustic Emission 3":refnum<vi>, "SNext":refnum<vi>, "APBack":refnum<vi>, "Enter the Temperature (°C):":refnum<vi>, "Enter the Stage \nTemperature (°C):":refnum<vi>, "Enter the Humidity (%Rh):":refnum<vi>, "Low Temp":refnum<vi>, "High Temp":refnum<vi>, "Humidity":refnum<vi>, "Sensors Picked":refnum<vi>}, "About Screen":cluster{"Password":refnum<vi>, "Home Service":refnum<vi>, "Advanced Setting":refnum<vi>, "About Tab":refnum<vi>, "ECR Port:":refnum<vi>, "Ramp Port:":refnum<vi>, "Installation/Replacement completed":refnum<vi>, "Loahead":refnum<vi>, "Heave and Surge COM Port:":refnum<vi>, "Sway COM Port:":refnum<vi>, "Temp Modbus:":refnum<vi>, "Humidity Port:":refnum<vi>, "Edit Gain Constants":refnum<vi>, "Save Gain Constants":refnum<vi>}, "Main Screen":cluster{"Main Screen Tab":refnum<vi>, "Angle and Frequency":refnum<vi>, "Stroke (mm)":refnum<vi>, "Angle (Deg)":refnum<vi>, "Main Speed Tab":refnum<vi>, "MTM MOTOR DISPLAY":refnum<vi>, "Disc Speed (m/sec)":refnum<vi>, "Ball Speed (m/sec)":refnum<vi>, "Disc Speed (RPM)":refnum<vi>, "Ball Speed (RPM)":refnum<vi>, "SPEED TAB":refnum<vi>, "Speed (m/sec)":refnum<vi>, "Set Speed (m/sec)":refnum<vi>, "Speed (RPM)":refnum<vi>, "Set Speed":refnum<vi>, "Time Tab":refnum<vi>, "Time ( HH:MM:SS ) 2":refnum<vi>, "Test Duration":refnum<vi>, "Test Duration 4":refnum<vi>, "TEST CYCLE":refnum<vi>, "TOTAL CYCLES":refnum<vi>, "Set Load (N)":refnum<vi>, "Temp Tabs":refnum<vi>, "Heater":refnum<vi>, "TK4 status":refnum<vi>, "ChamberTemp":refnum<vi>, "SetTmp":refnum<vi>, "Controller  Status":refnum<vi>, "ChamberTemp 2":refnum<vi>, "SetTmp 2":refnum<vi>, "Controller  Status 2":refnum<vi>, "ChamberTemp 3":refnum<vi>, "SetTmp 3":refnum<vi>, "Cooling":refnum<vi>, "Load Communication":refnum<vi>, "Ambient \nTemperature":refnum<vi>, "HumCOMStatus":refnum<vi>, "Ambient\n Humidity":refnum<vi>, "Freq (Hz)":refnum<vi>, "Load En":refnum<vi>, "NLt":refnum<vi>, "zNL 2":refnum<vi>, "Humidity On":refnum<vi>, "humidity disp":refnum<vi>, "Set Humidity":refnum<vi>, "NL disp 2":refnum<vi>, "Humidity On 2":refnum<vi>, "humidity disp 2":refnum<vi>, "Set Humidity 2":refnum<vi>, "NL disp 3":refnum<vi>, "AppLoadSeq scratch":refnum<vi>, "Stop Scratch":refnum<vi>, "ClrLog":refnum<vi>, "Trip Log":refnum<vi>, "STOP":refnum<vi>, "Start Test":refnum<vi>, "Test status":refnum<vi>, "AR Led":refnum<vi>, "Data":refnum<vi>, "Health":refnum<vi>, "Sway COM Status":refnum<vi>, "Heave COM Status":refnum<vi>, "Grp Tab":refnum<vi>, "Sub Graph":refnum<vi>, "SD (mm)":refnum<vi>, "Siliding distance Reset Graph":refnum<vi>, "SDGp":refnum<vi>, "Humidity Reset Graph":refnum<vi>, "HumrGp":refnum<vi>, "Acoustic Emission (mV)":refnum<vi>, "Aqucostic Reset Graph":refnum<vi>, "gACQUOS":refnum<vi>, "ECR RESET":refnum<vi>, "ECR":refnum<vi>, "Temperature Reset":refnum<vi>, "Acoustic Emission (mV) 2":refnum<vi>, "Aqucostic Reset Graph 2":refnum<vi>, "gACQUOS 2":refnum<vi>, "ECR RESET 2":refnum<vi>, "ECR 2":refnum<vi>, "Temperature Reset 2":refnum<vi>, "Temperature (deg c)":refnum<vi>, "Speed Reset Graph":refnum<vi>, "Speed Tab":refnum<vi>, "MTM DISC  SPEED":refnum<vi>, "MTM BALL SPEED":refnum<vi>, "speed mm/sec":refnum<vi>, "Hymidity":refnum<vi>, "Humidity Disable trip":refnum<vi>, "CoF Trip  2":refnum<vi>, "Depth Trip":refnum<vi>, "Weart Deapth":refnum<vi>, "Depth Reset Graph":refnum<vi>, "Weart":refnum<vi>, "Depthz":refnum<vi>, "Depth (µm)":refnum<vi>, "WearGp":refnum<vi>, "NL Trip 2":refnum<vi>, "Load pid":refnum<vi>, "Load Disable Trip":refnum<vi>, "Load Reset Graph":refnum<vi>, "NL Display 4":refnum<vi>, "Main Chart 3":refnum<vi>, "BACK":refnum<vi>, "Depth Trip 2":refnum<vi>, "COF TRIP ":refnum<vi>, "Friction Force (N)":refnum<vi>, "FF Reset Graph":refnum<vi>, "FF Disable Trip":refnum<vi>, "FF TRIP":refnum<vi>, "COF Disable Trip":refnum<vi>, "COF Reset Graph":refnum<vi>, "Start Test Temp":refnum<vi>, "zFF":refnum<vi>, "Friction Force (N) Graph":refnum<vi>, "Coefficient of Friction":refnum<vi>, "Scratch Start Test":refnum<vi>, "FF Tab":refnum<vi>, "Cyclic Friction Force (N)":refnum<vi>, "CZ FF":refnum<vi>, "Cyclic Friction Force (N) Graph":refnum<vi>, "Cyclic Coefficient of Friction":refnum<vi>, "Cyclic FF TRIP":refnum<vi>, "Cyclic FF Disable Trip":refnum<vi>, "cyclic COF Disable Trip":refnum<vi>, "cyclic COF TRIP":refnum<vi>, "cyclic COF Reset Graph":refnum<vi>, "Cyclic FF Reset Graph":refnum<vi>}, "Loading":cluster{"Indentation":refnum<vi>, "Reference Sample":refnum<vi>, "Load Cell Communication Slide":refnum<vi>, "com 3":refnum<vi>, "com":refnum<vi>, "DecaForce COM Status":refnum<vi>, "Update":refnum<vi>, "Clear 3":refnum<vi>, "seq":refnum<vi>, "Stribeck table":refnum<vi>, "Stribeck Table  For loading":refnum<vi>, "Loading Mode":refnum<vi>, "Enter the Final Load (N)":refnum<vi>, "Enter the CoF Trip":refnum<vi>, "Enter the Friction Force Trip":refnum<vi>, "Enter the Normal load Trip":refnum<vi>, "Enter the Load  (N)":refnum<vi>, "KiloForce":refnum<vi>, "DecaForce ":refnum<vi>, "MicroForce":refnum<vi>, "LHBack":refnum<vi>, "LHNext":refnum<vi>, "Enter the Loading Rate (N/min)":refnum<vi>, "Message":refnum<vi>, "Warning 2":refnum<vi>, "SSP 0.75":refnum<vi>, "SSP 0.5":refnum<vi>, "SSP 0.3":refnum<vi>, "Warning":refnum<vi>, "gui GIF":refnum<vi>, "Communication is established":refnum<vi>, "AppLoad 4":refnum<vi>, "Multipoint":refnum<vi>, "Load Selection":refnum<vi>}, "PID":cluster{"Ramp MulFac":refnum<vi>, "pulses LoadDiffRamp(2..10)":refnum<vi>, "PulseControlRamp(diff<=3N)":refnum<vi>, "SetLoadDeadband(%) Load(0-10N)":refnum<vi>, "PID gains out delay (microForce)":refnum<vi>, "Ramp":refnum<vi>, "Gain 2":refnum<vi>, "pulses LoadDiff(2..10)":refnum<vi>, "pulses LoadDiff(11..50)":refnum<vi>, "PulseControl(diff<=3N)":refnum<vi>, "SetLoadDeadband(%)  2":refnum<vi>, "Dummy Run":refnum<vi>, "Vertical load (N)":refnum<vi>, "AutoTune":refnum<vi>, "Offset 3 ":refnum<vi>, "apply load":refnum<vi>, "Offset  3":refnum<vi>, "apply load 2":refnum<vi>, "Enter ByPass Load":refnum<vi>, "reinit 3":refnum<vi>, "output range delay":refnum<vi>, "PID gains out delay":refnum<vi>, "Bypass Load":refnum<vi>, "pulsesSent":refnum<vi>, "pulses ":refnum<vi>, "actpid":refnum<vi>, "gFF Rot":refnum<vi>, "pulses LoadDiff(21..1000)":refnum<vi>, "Delay":refnum<vi>, "deadband":refnum<vi>}, "Config Parameters":cluster{"Tab Control 3":refnum<vi>, "Tab Control 19":refnum<vi>, "SAMPLES":refnum<vi>, "Re-initilaize":refnum<vi>, "Filter ON/OFF":refnum<vi>, "TracHomeSurgeOffsetCounts 10MM":refnum<vi>, "TracHomeSwayOffsetCounts 10MM":refnum<vi>, "Acoustic Emission:":refnum<vi>, "Apply Filter (FF)":refnum<vi>, "Filter% 2":refnum<vi>, "Apply Filter (Load)":refnum<vi>, "Filter% ":refnum<vi>, "Sway distance (mm)":refnum<vi>, "Surge distance (mm)":refnum<vi>, "DataSavingLoopDelay(ms)":refnum<vi>, "SAVE 2":refnum<vi>, "Enter Distance":refnum<vi>, "Sway Counts:":refnum<vi>, "Distance (mm): 3":refnum<vi>, "Surge Counts:":refnum<vi>, "Distance (mm): 2":refnum<vi>, "Distance (mm):":refnum<vi>, "Heave Counts:":refnum<vi>, "LRMHomeSurgeOffsetCounts":refnum<vi>, "LRMHomeSwayOffsetCounts":refnum<vi>, "TracHomeSurgeOffsetCounts 20MM":refnum<vi>, "TracHomeSwayOffsetCounts 20MM":refnum<vi>, "RotHomeSwayOffsetCounts":refnum<vi>, "RotHomeSurgeOffsetCounts":refnum<vi>, "Heave distance":refnum<vi>, "Zmm":refnum<vi>, "Heave Pulses/mm":refnum<vi>, "Surge Pulses/mm":refnum<vi>, "Sway Pulses/mm":refnum<vi>, "Heave Pitch":refnum<vi>, "Surge Pitch":refnum<vi>, "Sway Pitch":refnum<vi>, "Heave PPR":refnum<vi>, "Surge PPR":refnum<vi>, "Sway PPR":refnum<vi>, "Tab Control 5":refnum<vi>, "Tab Control 14":refnum<vi>, "Tab Control 26":refnum<vi>, "AE":refnum<vi>, "Heave Loop Delay":refnum<vi>, "Heave PID Speed":refnum<vi>, "Surge Jog Speed":refnum<vi>, "Heave Jog Speed":refnum<vi>, "Sway Loop Delay":refnum<vi>, "Sway PID Speed":refnum<vi>, "Sway Jog Speed":refnum<vi>}, "Loading Com Port":cluster{"ClearAll":refnum<vi>, "Mz(Nm)":refnum<vi>, "My(Nm)":refnum<vi>, "Mx(Nm)":refnum<vi>, "Save Dwell":refnum<vi>, "Mx ":refnum<vi>, "My ":refnum<vi>, "Mz":refnum<vi>, "Fx(N)":refnum<vi>, "Fy(N)":refnum<vi>, "Fz(N)":refnum<vi>, "ZeroAll":refnum<vi>, "Acq Delay (ms)":refnum<vi>, "Burst Delay (ms)":refnum<vi>, "model":refnum<vi>, "SN":refnum<vi>, "FFx(N)":refnum<vi>, "Sensor IP":refnum<vi>, "Port":refnum<vi>, "FFy(N)":refnum<vi>, "Load(N)":refnum<vi>, "delete Handle":refnum<vi>, "Create Handle":refnum<vi>, "ft_data":refnum<vi>, "ft_range":refnum<vi>, "ft_data 2":refnum<vi>, "stop 6":refnum<vi>, "running_flag":refnum<vi>, "ft_udp_handle":refnum<vi>, "get-data-return":refnum<vi>, "get-range-return":refnum<vi>, "zero-return":refnum<vi>, "filter-return":refnum<vi>, "initial-return":refnum<vi>, "deleteHandle-result":refnum<vi>, "Load Cell Temp":refnum<vi>}, "Heave AND Surge":cluster{"SURGE POSE":refnum<vi>, "error out Read":refnum<vi>, "HEAVE POSE":refnum<vi>, "State":refnum<vi>, "Homed":refnum<vi>, "Sequence ID":refnum<vi>, "error out Write":refnum<vi>, "faultCode":refnum<vi>, "Ack ID":refnum<vi>, "SPEED":refnum<vi>, "Distance":refnum<vi>, "Mode Command":refnum<vi>, "Heave and Surge Read":refnum<vi>, "Read Heave Temp":refnum<vi>, "Spare 15":refnum<vi>, "Spare 14":refnum<vi>, "Spare 13":refnum<vi>, "Spare 12":refnum<vi>, "Spare 11":refnum<vi>, "Spare 10":refnum<vi>, "Spare 9":refnum<vi>, "Spare 8":refnum<vi>, "Spare 7":refnum<vi>, "Spare 6":refnum<vi>, "Spare 5":refnum<vi>, "Spare 4":refnum<vi>, "Spare 2":refnum<vi>, "Spare 1":refnum<vi>, "Node Id":refnum<vi>, "Spare 3":refnum<vi>, "SPARE 4":refnum<vi>, "SPARE 3":refnum<vi>, "SPARE 2":refnum<vi>, "SPARE 1":refnum<vi>, "fwMajor":refnum<vi>, "fwMinor":refnum<vi>, "Manual Write":refnum<vi>, "Heave and Surge Write":refnum<vi>}, "New PID LOGIC":cluster{"Fine Tune Zone":refnum<vi>, "PID SDelay":refnum<vi>, "Max_pos_limit":refnum<vi>, "Min_pos_limit":refnum<vi>, "i_limit":refnum<vi>, "pct_scale":refnum<vi>, "Deadband":refnum<vi>, "Kd":refnum<vi>, "Ki":refnum<vi>, "Kp":refnum<vi>, "Current Position":refnum<vi>, "Set Load":refnum<vi>, "Current Load":refnum<vi>, "Pulse delta":refnum<vi>, "Init Step":refnum<vi>, "Max Step Linit":refnum<vi>}, "SWAY ":cluster{"fwMajor":refnum<vi>, "Homed":refnum<vi>, "Rotary POSE":refnum<vi>, "State":refnum<vi>, "SWAY POSE":refnum<vi>, "Ack ID":refnum<vi>, "faultCode":refnum<vi>, "Node Id":refnum<vi>, "fwMinor":refnum<vi>, "Spare 6":refnum<vi>, "Spare 5":refnum<vi>, "Spare 4":refnum<vi>, "Spare 3":refnum<vi>, "Spare 2":refnum<vi>, "Spare 1":refnum<vi>, "Spare 7":refnum<vi>, "SPARE  5":refnum<vi>, "error out Write  SWAY ":refnum<vi>, "error out Read SWAY ":refnum<vi>, "Manual Write SWAY ":refnum<vi>, "SWAY WRITE":refnum<vi>, "SPARE  4":refnum<vi>, "SPARE  3":refnum<vi>, "SPARE 2":refnum<vi>, "SPARE 1":refnum<vi>, "Spare 15":refnum<vi>, "Spare 14":refnum<vi>, "Spare 13":refnum<vi>, "Spare 12":refnum<vi>, "Spare 11":refnum<vi>, "Spare 9":refnum<vi>, "Spare 8":refnum<vi>, "SPEED":refnum<vi>, "Distance":refnum<vi>, "Mode Command":refnum<vi>, "Sequence ID":refnum<vi>, "SWAY READ":refnum<vi>, "Spare 10":refnum<vi>, "Read SWAY Temp":refnum<vi>}}
  T12 = typedef "init queue out loop.ctl" = cluster{"UI Loop":refnum<queue>, "LOAD COM LOOP ":refnum<queue>, "SWAY MOTOR COM LOOP":refnum<queue>, "HEAVE MOTOR COM LOOP":refnum<queue>, "TEMPERATURE COM LOOP":refnum<queue>, "RAMP MOTOR COM LOOP":refnum<queue>, "ECR PORT":refnum<queue>, "HUMIDITY COM PORT":refnum<queue>, "PROGRAM LOOP":refnum<queue>, "MONITOR LOOP":refnum<queue>, "REPORT":refnum<queue>, "LOAD PID":refnum<queue>}
  T13 = enum8{"Enabled", "Disabled", "Disabled and Grayed Out"}
  T14 = enum16{"INIT", "SETLOWPASSFILTER", "SETZERO", "GETSENSORINFO", "GETRANGE", "ZEROALL", "READDATA", "UNINITIAL", "DELETEHANDLE"}
  T15 = typedef "Heave Write enum.ctl" = enum16{"INIT", "WRITE", "CLOSE", "REINIT"}
  T16 = typedef "Sway Write enum.ctl" = enum16{"INIT", "WRITE", "CLOSE", "REINIT"}
  T17 = typedef "Sway Right enum.ctl" = enum16{"INIT", "READ", "CLOSE", "REINIT", ""}
  T18 = typedef "Heave Right enum.ctl" = enum16{"INIT", "READ", "CLOSE", "REINIT", ""}
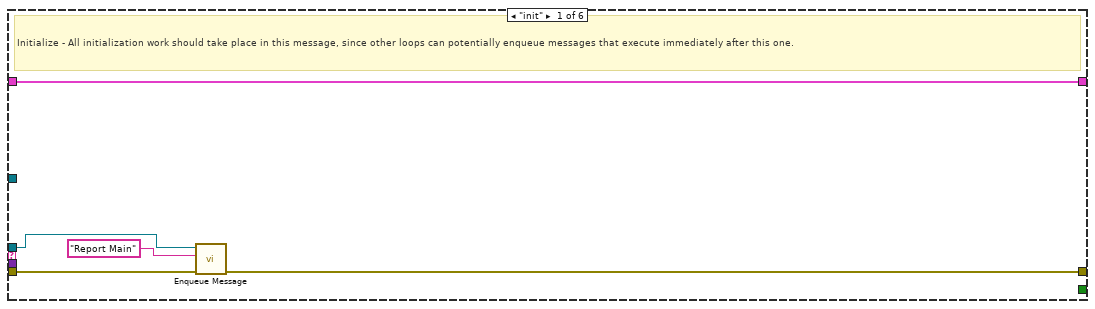
[diagram p2: hidden frame]
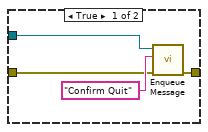
[diagram p3: hidden frame]
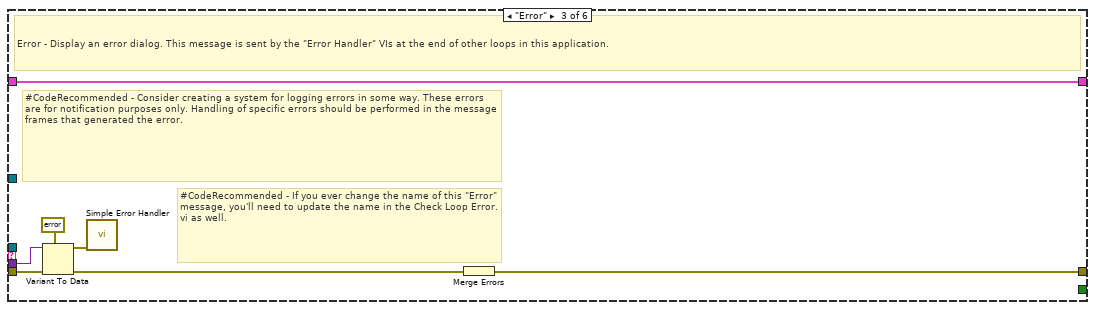
[diagram p4: hidden frame]
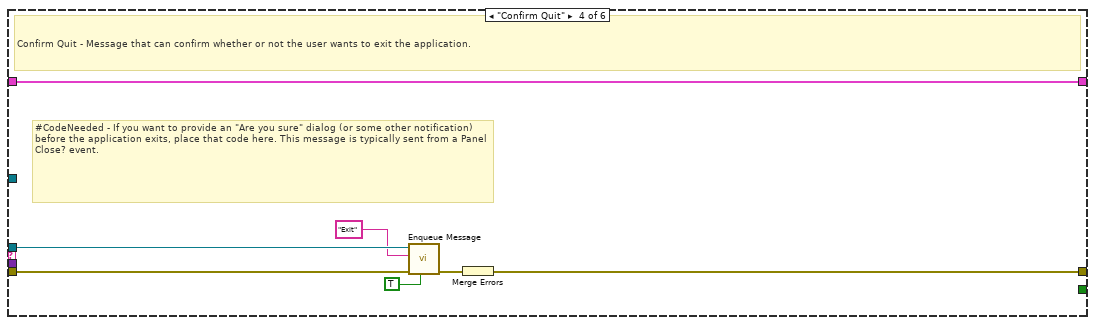
[diagram p5: hidden frame]
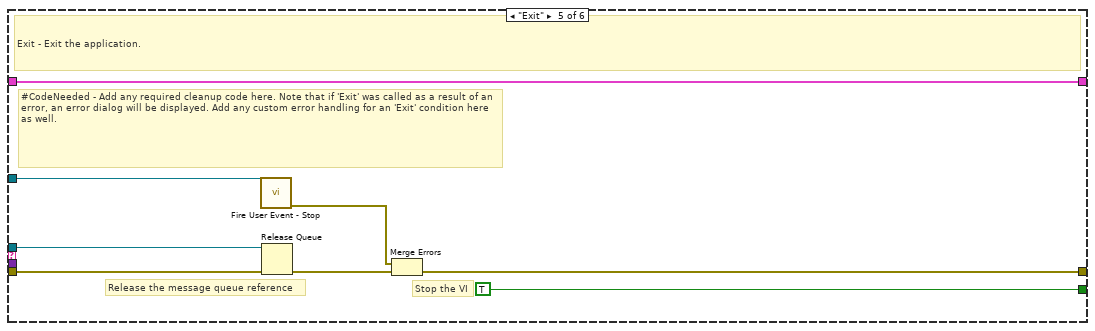
[diagram p6: hidden frame]
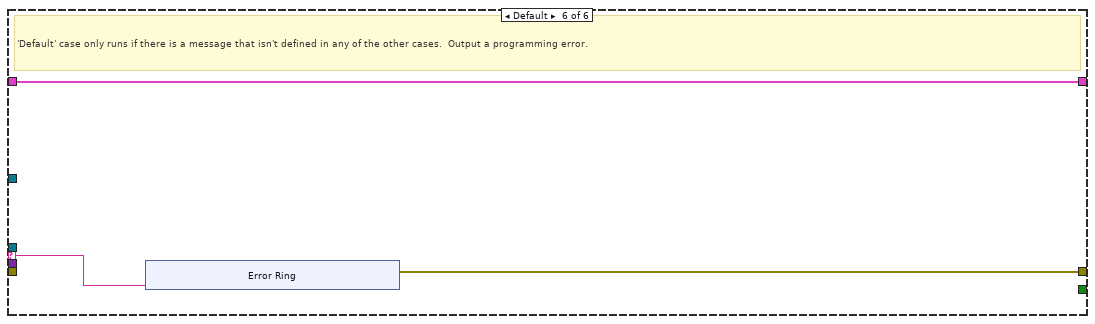
[diagram p7: hidden frame]
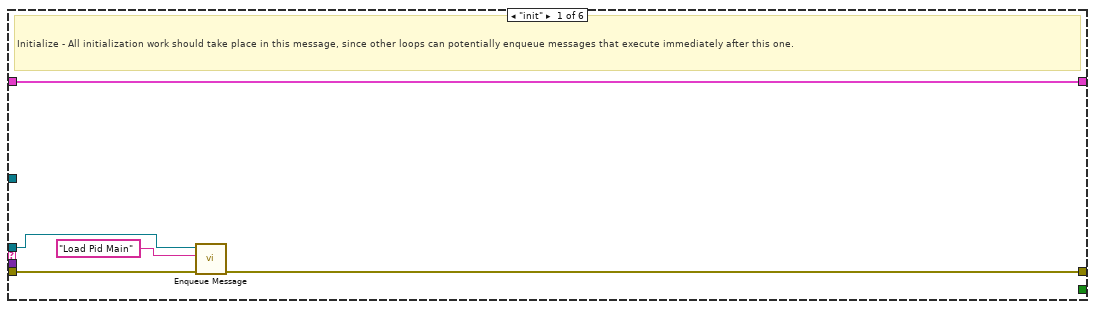
[diagram p8: hidden frame]
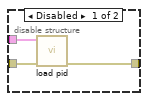
[diagram p10: hidden frame]
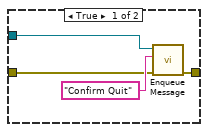
[diagram p11: hidden frame]
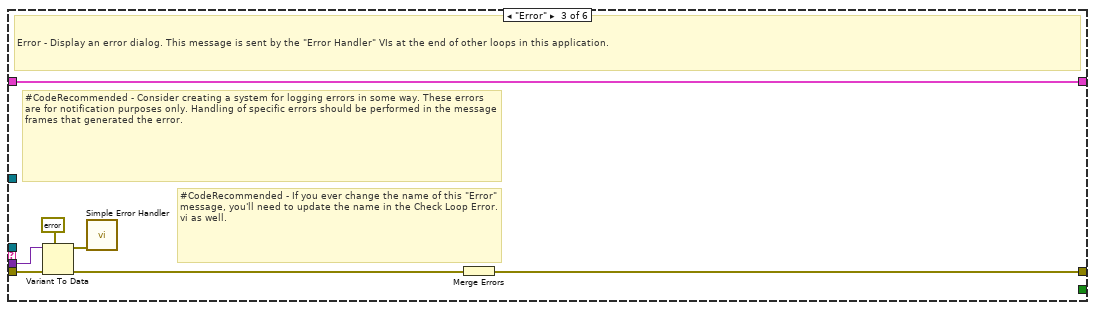
[diagram p12: hidden frame]
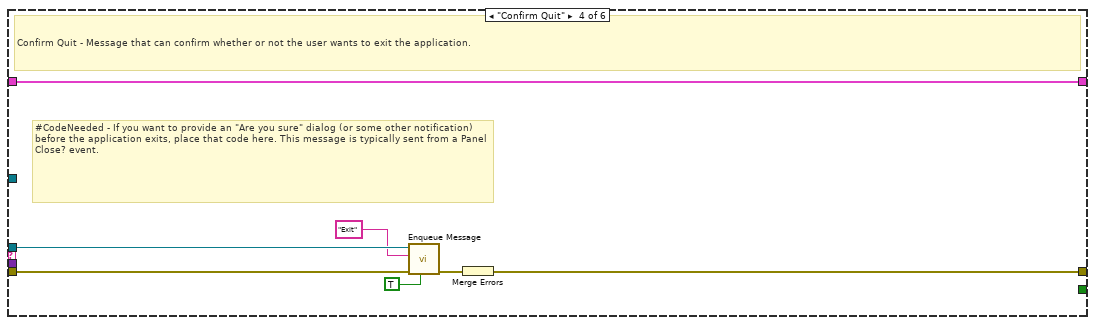
[diagram p13: hidden frame]
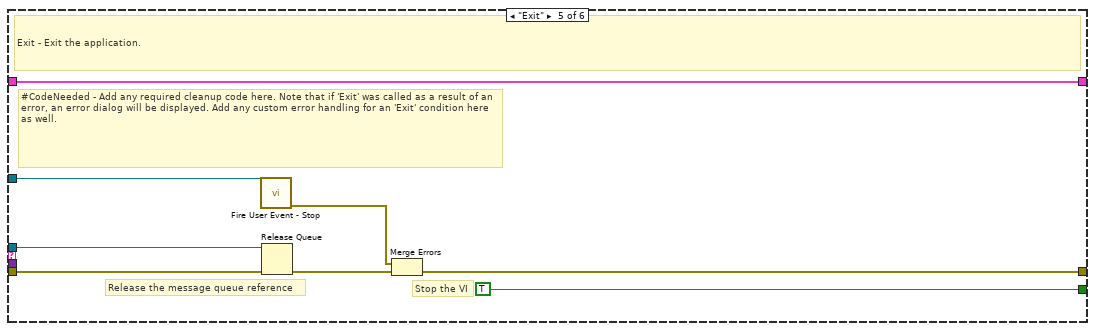
[diagram p14: hidden frame]
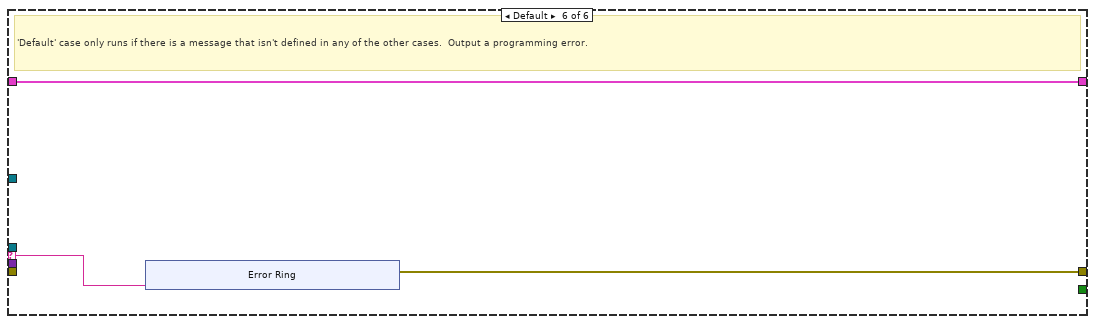
[diagram p15: hidden frame]
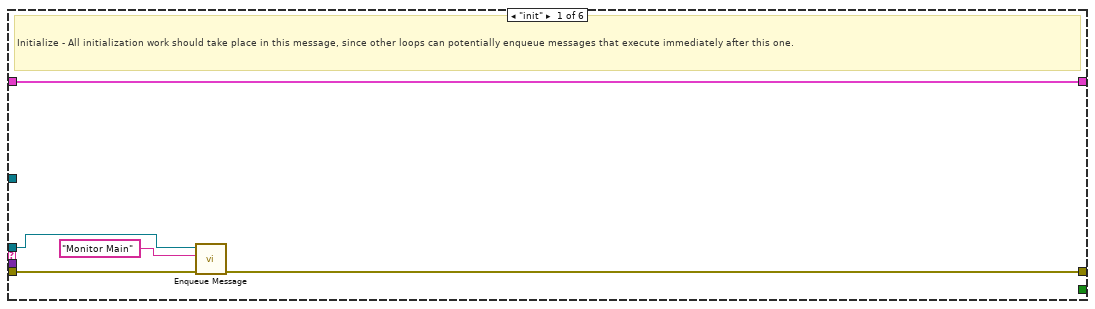
[diagram p16: hidden frame]
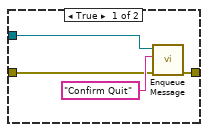
[diagram p17: hidden frame]
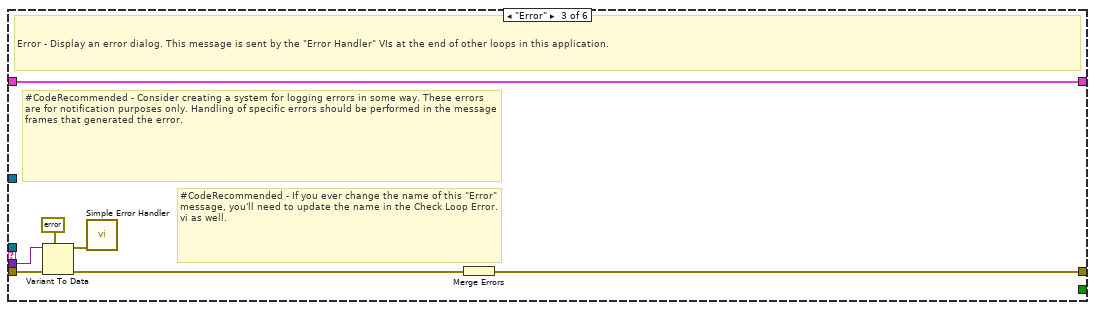
[diagram p18: hidden frame]
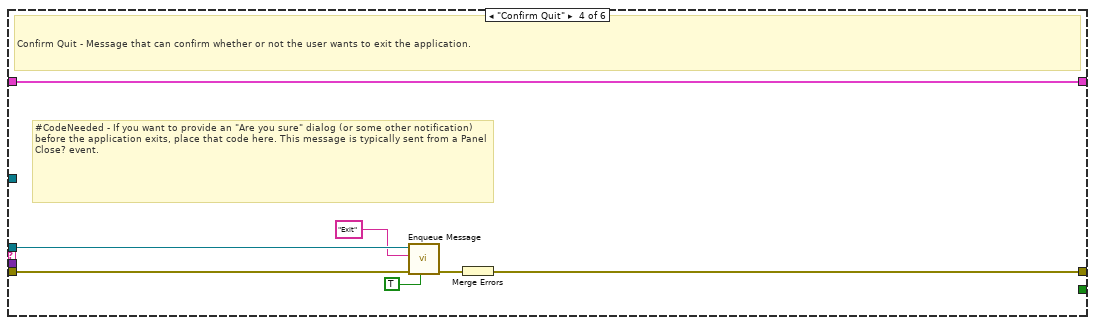
[diagram p19: hidden frame]
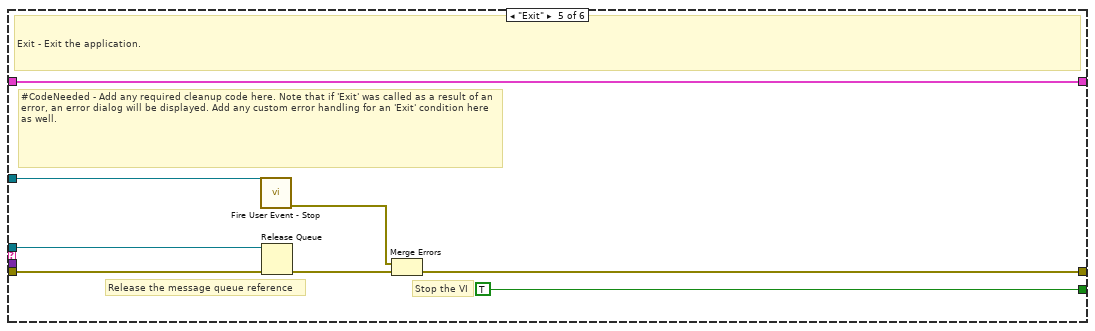
[diagram p20: hidden frame]
diagram:
  # "Select Load Head"
  n1 = flat-sequence {
    tunnel: [w55] -> w42
    tunnel: T11 {"Main Home Screen"={"GUI"=refnum, "Platform Settings"=refnum, "Configure"=refnum, "Home"=refnum, "EXIT"=refnum, "service 2"=refnum, "MainPage"=refnum, "Analysis"=refnum}, "Platform Settings"={"mm/s  Surge"=refnum, "Update Surge Speed"=refnum, "Drive Error"=refnum, "Disable Axis Jog Soft Limits"=refnum, "mm/s  Sway"=refnum, "Sway and Surge COM Status"=refnum, "Heave COM Status"=refnum, "Enable Platform"=refnum, "Surge Forward Main"=refnum, "Sway Right Main"=refnum, "Sway Left Main"=refnum, "Heave Down Main"=refnum, "Heave Up main"=refnum, "Update Sway Speed"=refnum, "Update Heave Speed"=refnum, "mm/s Heave"=refnum, "mm/sec"=refnum, "mm"=refnum, "Surge Backward Main"=refnum}, "Analysis Screen"={"Analysis Home"=refnum, "Surface Analysis"=refnum, "Imaging"=refnum, "Image Analysis"=refnum, "Post Analysis"=refnum}, "Config Screen"={"Select Load Head"=refnum, "Notes :"=refnum, "FILE"=refnum, "Sample ID :"=refnum, "Operator ID :"=refnum, "Operator Name :"=refnum, "Auto"=refnum}, "Motion Module"={"zNL"=refnum, "NL disp"=refnum, "Rotary Tab"=refnum, "Motion Direction:  3"=refnum, "E.Velocity 2"=refnum, "e.v/ssr 2"=refnum, "Enter Fixed E.Velocity 2"=refnum, "Enter Final SRR 2"=refnum, "Enter initial SRR 2"=refnum, "Enter Fixed SRR 2"=refnum, "Enter the Final E.Velocity (m/s) 2"=refnum, "Enter initial E.Velocity (m/s) 2"=refnum, "Final Speed (RPM) 3"=refnum, "Initial Speed (RPM) 2"=refnum, "Enter the Final Velocity (m/s) 3"=refnum, "Enter initial Velocity (m/s)  3"=refnum, "Ramp Up 2"=refnum, "TEST SELECTION"=refnum, "SPEED SELECTION : "=refnum, "Angular Oscillation Set"=refnum, "Traction"=refnum, "Step Speed"=refnum, "StepTable For Load-Speed"=refnum, "StepTable For Speed"=refnum, "Surge Forward MM"=refnum, "Surge Backward MM"=refnum, "M3 Image"=refnum, "String 39"=refnum, "Sway Left MM"=refnum, "Sway Right MM"=refnum, "Disable Axis Jog Soft Limits"=refnum, "mm"=refnum, "Heave Down MM"=refnum, "Heave Up MM"=refnum, "Wear Track Diameter (mm)"=refnum, "Set WTD"=refnum, "HomeScratch"=refnum, "HomeRot"=refnum, "PlaceModule"=refnum, "Enter the Angle (Deg)"=refnum, "Enter the Frequency (Hz)"=refnum, "Motion Mode:"=refnum, "LR Sway"=refnum, "Rot Hor"=refnum, "Scratch"=refnum, "LR Cam"=refnum, "MMBack"=refnum, "MMNext"=refnum, "Rot Ver"=refnum, "Rotary Module Selection"=refnum, "calculate rotary"=refnum, "SPEED SELECTION : rotary"=refnum, "Import 2"=refnum, "Save 2"=refnum, "File Path :  2"=refnum, "String 45"=refnum, "StepTable For Speed 3"=refnum, "Enter the Speed(mm/sec)"=refnum, "Enter the Speed(RPM)"=refnum, "Enter Scratch Speed (mm/s):"=refnum, "SwaySpeed Set"=refnum, "Scartch Offset"=refnum, "Scratch Mode:"=refnum, "Motion type:"=refnum, "HomeScratch 2"=refnum, "Enter Scratch length (mm):"=refnum, "Wear Track Diameter"=refnum, "Rotary Speed Exced"=refnum}, "Environmental control"={"Humidity  Status  3"=refnum, "Low Temp  Status  2"=refnum, "TK4 status 2"=refnum, "Stage Temperature"=refnum, "Sample Temperature"=refnum, "Humidity (Amb)"=refnum, "Clear List"=refnum, "Add to list"=refnum, "Wear"=refnum, "Vibration"=refnum, "Humidity (Chamber)"=refnum, "Temperature (Chamber)"=refnum, "ECR "=refnum, "Temperature (Amb)"=refnum, "Microphone"=refnum, "Acoustic Emission 3"=refnum, "SNext"=refnum, "APBack"=refnum, "Enter the Temperature (°C):"=refnum, "Enter the Stage \nTemperature (°C):"=refnum, "Enter the Humidity (%Rh):"=refnum, "Low Temp"=refnum, "High Temp"=refnum, "Humidity"=refnum, "Sensors Picked"=refnum}, "About Screen"={"Password"=refnum, "Home Service"=refnum, "Advanced Setting"=refnum, "About Tab"=refnum, "ECR Port:"=refnum, "Ramp Port:"=refnum, "Installation/Replacement completed"=refnum, "Loahead"=refnum, "Heave and Surge COM Port:"=refnum, "Sway COM Port:"=refnum, "Temp Modbus:"=refnum, "Humidity Port:"=refnum, "Edit Gain Constants"=refnum, "Save Gain Constants"=refnum}, "Main Screen"={"Main Screen Tab"=refnum, "Angle and Frequency"=refnum, "Stroke (mm)"=refnum, "Angle (Deg)"=refnum, "Main Speed Tab"=refnum, "MTM MOTOR DISPLAY"=refnum, "Disc Speed (m/sec)"=refnum, "Ball Speed (m/sec)"=refnum, "Disc Speed (RPM)"=refnum, "Ball Speed (RPM)"=refnum, "SPEED TAB"=refnum, "Speed (m/sec)"=refnum, "Set Speed (m/sec)"=refnum, "Speed (RPM)"=refnum, "Set Speed"=refnum, "Time Tab"=refnum, "Time ( HH:MM:SS ) 2"=refnum, "Test Duration"=refnum, "Test Duration 4"=refnum, "TEST CYCLE"=refnum, "TOTAL CYCLES"=refnum, "Set Load (N)"=refnum, "Temp Tabs"=refnum, "Heater"=refnum, "TK4 status"=refnum, "ChamberTemp"=refnum, "SetTmp"=refnum, "Controller  Status"=refnum, "ChamberTemp 2"=refnum, "SetTmp 2"=refnum, "Controller  Status 2"=refnum, "ChamberTemp 3"=refnum, "SetTmp 3"=refnum, "Cooling"=refnum, "Load Communication"=refnum, "Ambient \nTemperature"=refnum, "HumCOMStatus"=refnum, "Ambient\n Humidity"=refnum, "Freq (Hz)"=refnum, "Load En"=refnum, "NLt"=refnum, "zNL 2"=refnum, "Humidity On"=refnum, "humidity disp"=refnum, "Set Humidity"=refnum, "NL disp 2"=refnum, "Humidity On 2"=refnum, "humidity disp 2"=refnum, "Set Humidity 2"=refnum, "NL disp 3"=refnum, "AppLoadSeq scratch"=refnum, "Stop Scratch"=refnum, "ClrLog"=refnum, "Trip Log"=refnum, "STOP"=refnum, "Start Test"=refnum, "Test status"=refnum, "AR Led"=refnum, "Data"=refnum, "Health"=refnum, "Sway COM Status"=refnum, "Heave COM Status"=refnum, "Grp Tab"=refnum, "Sub Graph"=refnum, "SD (mm)"=refnum, "Siliding distance Reset Graph"=refnum, "SDGp"=refnum, "Humidity Reset Graph"=refnum, "HumrGp"=refnum, "Acoustic Emission (mV)"=refnum, "Aqucostic Reset Graph"=refnum, "gACQUOS"=refnum, "ECR RESET"=refnum, "ECR"=refnum, "Temperature Reset"=refnum, "Acoustic Emission (mV) 2"=refnum, "Aqucostic Reset Graph 2"=refnum, "gACQUOS 2"=refnum, "ECR RESET 2"=refnum, "ECR 2"=refnum, "Temperature Reset 2"=refnum, "Temperature (deg c)"=refnum, "Speed Reset Graph"=refnum, "Speed Tab"=refnum, "MTM DISC  SPEED"=refnum, "MTM BALL SPEED"=refnum, "speed mm/sec"=refnum, "Hymidity"=refnum, "Humidity Disable trip"=refnum, "CoF Trip  2"=refnum, "Depth Trip"=refnum, "Weart Deapth"=refnum, "Depth Reset Graph"=refnum, "Weart"=refnum, "Depthz"=refnum, "Depth (µm)"=refnum, "WearGp"=refnum, "NL Trip 2"=refnum, "Load pid"=refnum, "Load Disable Trip"=refnum, "Load Reset Graph"=refnum, "NL Display 4"=refnum, "Main Chart 3"=refnum, "BACK"=refnum, "Depth Trip 2"=refnum, "COF TRIP "=refnum, "Friction Force (N)"=refnum, "FF Reset Graph"=refnum, "FF Disable Trip"=refnum, "FF TRIP"=refnum, "COF Disable Trip"=refnum, "COF Reset Graph"=refnum, "Start Test Temp"=refnum, "zFF"=refnum, "Friction Force (N) Graph"=refnum, "Coefficient of Friction"=refnum, "Scratch Start Test"=refnum, "FF Tab"=refnum, "Cyclic Friction Force (N)"=refnum, "CZ FF"=refnum, "Cyclic Friction Force (N) Graph"=refnum, "Cyclic Coefficient of Friction"=refnum, "Cyclic FF TRIP"=refnum, "Cyclic FF Disable Trip"=refnum, "cyclic COF Disable Trip"=refnum, "cyclic COF TRIP"=refnum, "cyclic COF Reset Graph"=refnum, "Cyclic FF Reset Graph"=refnum}, "Loading"={"Indentation"=refnum, "Reference Sample"=refnum, "Load Cell Communication Slide"=refnum, "com 3"=refnum, "com"=refnum, "DecaForce COM Status"=refnum, "Update"=refnum, "Clear 3"=refnum, "seq"=refnum, "Stribeck table"=refnum, "Stribeck Table  For loading"=refnum, "Loading Mode"=refnum, "Enter the Final Load (N)"=refnum, "Enter the CoF Trip"=refnum, "Enter the Friction Force Trip"=refnum, "Enter the Normal load Trip"=refnum, "Enter the Load  (N)"=refnum, "KiloForce"=refnum, "DecaForce "=refnum, "MicroForce"=refnum, "LHBack"=refnum, "LHNext"=refnum, "Enter the Loading Rate (N/min)"=refnum, "Message"=refnum, "Warning 2"=refnum, "SSP 0.75"=refnum, "SSP 0.5"=refnum, "SSP 0.3"=refnum, "Warning"=refnum, "gui GIF"=refnum, "Communication is established"=refnum, "AppLoad 4"=refnum, "Multipoint"=refnum, "Load Selection"=refnum}, "PID"={"Ramp MulFac"=refnum, "pulses LoadDiffRamp(2..10)"=refnum, "PulseControlRamp(diff<=3N)"=refnum, "SetLoadDeadband(%) Load(0-10N)"=refnum, "PID gains out delay (microForce)"=refnum, "Ramp"=refnum, "Gain 2"=refnum, "pulses LoadDiff(2..10)"=refnum, "pulses LoadDiff(11..50)"=refnum, "PulseControl(diff<=3N)"=refnum, "SetLoadDeadband(%)  2"=refnum, "Dummy Run"=refnum, "Vertical load (N)"=refnum, "AutoTune"=refnum, "Offset 3 "=refnum, "apply load"=refnum, "Offset  3"=refnum, "apply load 2"=refnum, "Enter ByPass Load"=refnum, "reinit 3"=refnum, "output range delay"=refnum, "PID gains out delay"=refnum, "Bypass Load"=refnum, "pulsesSent"=refnum, "pulses "=refnum, "actpid"=refnum, "gFF Rot"=refnum, "pulses LoadDiff(21..1000)"=refnum, "Delay"=refnum, "deadband"=refnum}, "Config Parameters"={"Tab Control 3"=refnum, "Tab Control 19"=refnum, "SAMPLES"=refnum, "Re-initilaize"=refnum, "Filter ON/OFF"=refnum, "TracHomeSurgeOffsetCounts 10MM"=refnum, "TracHomeSwayOffsetCounts 10MM"=refnum, "Acoustic Emission:"=refnum, "Apply Filter (FF)"=refnum, "Filter% 2"=refnum, "Apply Filter (Load)"=refnum, "Filter% "=refnum, "Sway distance (mm)"=refnum, "Surge distance (mm)"=refnum, "DataSavingLoopDelay(ms)"=refnum, "SAVE 2"=refnum, "Enter Distance"=refnum, "Sway Counts:"=refnum, "Distance (mm): 3"=refnum, "Surge Counts:"=refnum, "Distance (mm): 2"=refnum, "Distance (mm):"=refnum, "Heave Counts:"=refnum, "LRMHomeSurgeOffsetCounts"=refnum, "LRMHomeSwayOffsetCounts"=refnum, "TracHomeSurgeOffsetCounts 20MM"=refnum, "TracHomeSwayOffsetCounts 20MM"=refnum, "RotHomeSwayOffsetCounts"=refnum, "RotHomeSurgeOffsetCounts"=refnum, "Heave distance"=refnum, "Zmm"=refnum, "Heave Pulses/mm"=refnum, "Surge Pulses/mm"=refnum, "Sway Pulses/mm"=refnum, "Heave Pitch"=refnum, "Surge Pitch"=refnum, "Sway Pitch"=refnum, "Heave PPR"=refnum, "Surge PPR"=refnum, "Sway PPR"=refnum, "Tab Control 5"=refnum, "Tab Control 14"=refnum, "Tab Control 26"=refnum, "AE"=refnum, "Heave Loop Delay"=refnum, "Heave PID Speed"=refnum, "Surge Jog Speed"=refnum, "Heave Jog Speed"=refnum, "Sway Loop Delay"=refnum, "Sway PID Speed"=refnum, "Sway Jog Speed"=refnum}, "Loading Com Port"={"ClearAll"=refnum, "Mz(Nm)"=refnum, "My(Nm)"=refnum, "Mx(Nm)"=refnum, "Save Dwell"=refnum, "Mx "=refnum, "My "=refnum, "Mz"=refnum, "Fx(N)"=refnum, "Fy(N)"=refnum, "Fz(N)"=refnum, "ZeroAll"=refnum, "Acq Delay (ms)"=refnum, "Burst Delay (ms)"=refnum, "model"=refnum, "SN"=refnum, "FFx(N)"=refnum, "Sensor IP"=refnum, "Port"=refnum, "FFy(N)"=refnum, "Load(N)"=refnum, "delete Handle"=refnum, "Create Handle"=refnum, "ft_data"=refnum, "ft_range"=refnum, "ft_data 2"=refnum, "stop 6"=refnum, "running_flag"=refnum, "ft_udp_handle"=refnum, "get-data-return"=refnum, "get-range-return"=refnum, "zero-return"=refnum, "filter-return"=refnum, "initial-return"=refnum, "deleteHandle-result"=refnum, "Load Cell Temp"=refnum}, "Heave AND Surge"={"SURGE POSE"=refnum, "error out Read"=refnum, "HEAVE POSE"=refnum, "State"=refnum, "Homed"=refnum, "Sequence ID"=refnum, "error out Write"=refnum, "faultCode"=refnum, "Ack ID"=refnum, "SPEED"=refnum, "Distance"=refnum, "Mode Command"=refnum, "Heave and Surge Read"=refnum, "Read Heave Temp"=refnum, "Spare 15"=refnum, "Spare 14"=refnum, "Spare 13"=refnum, "Spare 12"=refnum, "Spare 11"=refnum, "Spare 10"=refnum, "Spare 9"=refnum, "Spare 8"=refnum, "Spare 7"=refnum, "Spare 6"=refnum, "Spare 5"=refnum, "Spare 4"=refnum, "Spare 2"=refnum, "Spare 1"=refnum, "Node Id"=refnum, "Spare 3"=refnum, "SPARE 4"=refnum, "SPARE 3"=refnum, "SPARE 2"=refnum, "SPARE 1"=refnum, "fwMajor"=refnum, "fwMinor"=refnum, "Manual Write"=refnum, "Heave and Surge Write"=refnum}, "New PID LOGIC"={"Fine Tune Zone"=refnum, "PID SDelay"=refnum, "Max_pos_limit"=refnum, "Min_pos_limit"=refnum, "i_limit"=refnum, "pct_scale"=refnum, "Deadband"=refnum, "Kd"=refnum, "Ki"=refnum, "Kp"=refnum, "Current Position"=refnum, "Set Load"=refnum, "Current Load"=refnum, "Pulse delta"=refnum, "Init Step"=refnum, "Max Step Linit"=refnum}, "SWAY "={"fwMajor"=refnum, "Homed"=refnum, "Rotary POSE"=refnum, "State"=refnum, "SWAY POSE"=refnum, "Ack ID"=refnum, "faultCode"=refnum, "Node Id"=refnum, "fwMinor"=refnum, "Spare 6"=refnum, "Spare 5"=refnum, "Spare 4"=refnum, "Spare 3"=refnum, "Spare 2"=refnum, "Spare 1"=refnum, "Spare 7"=refnum, "SPARE  5"=refnum, "error out Write  SWAY "=refnum, "error out Read SWAY "=refnum, "Manual Write SWAY "=refnum, "SWAY WRITE"=refnum, "SPARE  4"=refnum, "SPARE  3"=refnum, "SPARE 2"=refnum, "SPARE 1"=refnum, "Spare 15"=refnum, "Spare 14"=refnum, "Spare 13"=refnum, "Spare 12"=refnum, "Spare 11"=refnum, "Spare 9"=refnum, "Spare 8"=refnum, "SPEED"=refnum, "Distance"=refnum, "Mode Command"=refnum, "Sequence ID"=refnum, "SWAY READ"=refnum, "Spare 10"=refnum, "Read SWAY Temp"=refnum}} ("Data Cluster") -> [w54]
    tunnel: w42 -> [w84]
    tunnel: [w64] -> w41
    tunnel: w41 -> [w91]
    tunnel: [w85] -> w40
    tunnel: w40 -> [w100]
    tunnel: [w99] -> w39
    tunnel: w39 -> [w136]
    tunnel: [w135] -> w37
    tunnel: w37 -> [w206]
    tunnel: [w205] -> w36
    tunnel: w36 -> [w233]
    tunnel: [w232] -> w35
    tunnel: w35 -> [w249]
    tunnel: [w248] -> w34
    tunnel: w34 -> [w366]
    tunnel: [w365] -> w9
    tunnel: w9 -> [w396]
    tunnel: [w395] -> w8
    tunnel: w8 -> [w449]
    tunnel: [w448] -> w7
    tunnel: w7 -> [w486]
    tunnel: [w485] -> w6
    tunnel: w6 -> [w526]
    tunnel: [w525] -> w3
    tunnel: w3 -> [w544]
    tunnel: [w543] -> w2
    tunnel: [w584] -> w14
    tunnel: w2 -> [w585]
    frame #0 {
      n2 = control-ref of="GUI"() -> (w63:refnum<vi>)
      n3 = control-ref of="MainPage"() -> (w57:refnum<vi>)
      n4 = control-ref of="Platform Settings"() -> (w62:refnum<vi>)
      n5 = control-ref of="Configure"() -> (w61:refnum<vi>)
      n6 = control-ref of="Home"() -> (w60:refnum<vi>)
      n7 = control-ref of="EXIT"() -> (w59:refnum<vi>)
      n8 = control-ref of="service 2"() -> (w58:refnum<vi>)
      n9 = control-ref of="Analysis"() -> (w56:refnum<vi>)
      n10 = Bundle By Name(cluster=w54, "Main Home Screen.GUI"=w63, "Main Home Screen.Platform Settings"=w62, "Main Home Screen.Configure"=w61, "Main Home Screen.Home"=w60, "Main Home Screen.EXIT"=w59, "Main Home Screen.service 2"=w58, "Main Home Screen.MainPage"=w57, "Main Home Screen.Analysis"=w56) -> (w55:T11)
    }
    frame #1 {
      n11 = control-ref of="Sway Right Main"() -> (w74:refnum<vi>)
      n12 = control-ref of="Sway Left Main"() -> (w73:refnum<vi>)
      n13 = control-ref of="Heave Down Main"() -> (w72:refnum<vi>)
      n14 = control-ref of="Heave Up main"() -> (w71:refnum<vi>)
      n15 = control-ref of="Update Sway Speed"() -> (w70:refnum<vi>)
      n16 = control-ref of="Update Heave Speed"() -> (w69:refnum<vi>)
      n17 = control-ref of="Surge Backward Main"() -> (w65:refnum<vi>)
      n18 = control-ref of="Update Surge Speed"() -> (w82:refnum<vi>)
      n19 = control-ref of="Disable Axis Jog Soft Limits"() -> (w80:refnum<vi>)
      n20 = control-ref of="Sway and Surge COM Status"() -> (w78:refnum<vi>)
      n21 = control-ref of="Heave COM Status"() -> (w77:refnum<vi>)
      n22 = control-ref of="Enable Platform"() -> (w76:refnum<vi>)
      n23 = control-ref of="Surge Forward Main"() -> (w75:refnum<vi>)
      n24 = control-ref of="mm/s Heave"() -> (w68:refnum<vi>)
      n25 = control-ref of="mm/sec"() -> (w67:refnum<vi>)
      n26 = control-ref of="mm"() -> (w66:refnum<vi>)
      n27 = control-ref of="mm/s  Surge"() -> (w83:refnum<vi>)
      n28 = control-ref of="mm/s  Sway"() -> (w79:refnum<vi>)
      n29 = control-ref of="Drive Error"() -> (w81:refnum<vi>)
      n30 = Bundle By Name(cluster=w84, "Platform Settings.mm/s  Surge"=w83, "Platform Settings.Update Surge Speed"=w82, "Platform Settings.Drive Error"=w81, "Platform Settings.Disable Axis Jog Soft Limits"=w80, "Platform Settings.mm/s  Sway"=w79, "Platform Settings.Sway and Surge COM Status"=w78, "Platform Settings.Heave COM Status"=w77, "Platform Settings.Enable Platform"=w76, "Platform Settings.Surge Forward Main"=w75, "Platform Settings.Sway Right Main"=w74, "Platform Settings.Sway Left Main"=w73, "Platform Settings.Heave Down Main"=w72, "Platform Settings.Heave Up main"=w71, "Platform Settings.Update Sway Speed"=w70, "Platform Settings.Update Heave Speed"=w69, "Platform Settings.mm/s Heave"=w68, "Platform Settings.mm/sec"=w67, "Platform Settings.mm"=w66, "Platform Settings.Surge Backward Main"=w65) -> (w64:T11)
    }
    frame #2 {
      n31 = control-ref of="Analysis Home"() -> (w90:refnum<vi>)
      n32 = control-ref of="Surface Analysis"() -> (w89:refnum<vi>)
      n33 = control-ref of="Imaging"() -> (w88:refnum<vi>)
      n34 = control-ref of="Image Analysis"() -> (w87:refnum<vi>)
      n35 = control-ref of="Post Analysis"() -> (w86:refnum<vi>)
      n36 = Bundle By Name(cluster=w91, "Analysis Screen.Analysis Home"=w90, "Analysis Screen.Surface Analysis"=w89, "Analysis Screen.Imaging"=w88, "Analysis Screen.Image Analysis"=w87, "Analysis Screen.Post Analysis"=w86) -> (w85:T11)
    }
    frame #3 {
      n37 = control-ref of="Select Load Head"() -> (w98:refnum<vi>)
      n38 = control-ref of="Auto"() -> (w92:refnum<vi>)
      n39 = control-ref of="Notes :"() -> (w97:refnum<vi>)
      n40 = control-ref of="FILE"() -> (w96:refnum<vi>)
      n41 = control-ref of="Sample ID :"() -> (w95:refnum<vi>)
      n42 = control-ref of="Operator ID :"() -> (w94:refnum<vi>)
      n43 = control-ref of="Operator Name :"() -> (w93:refnum<vi>)
      n44 = Bundle By Name(cluster=w100, "Config Screen.Select Load Head"=w98, "Config Screen.Notes :"=w97, "Config Screen.FILE"=w96, "Config Screen.Sample ID :"=w95, "Config Screen.Operator ID :"=w94, "Config Screen.Operator Name :"=w93, "Config Screen.Auto"=w92) -> (w99:T11)
    }
    frame #4 {
      n45 = control-ref of="Warning"() -> (w128:refnum<vi>)
      n46 = control-ref of="gui GIF"() -> (w127:refnum<vi>)
      n47 = control-ref of="Load Selection"() -> (w101:refnum<vi>)
      n48 = control-ref of="Warning 2"() -> (w132:refnum<vi>)
      n49 = control-ref of="SSP 0.75"() -> (w131:refnum<vi>)
      n50 = control-ref of="SSP 0.5"() -> (w130:refnum<vi>)
      n51 = control-ref of="SSP 0.3"() -> (w129:refnum<vi>)
      n52 = control-ref of="Communication is established"() -> (w126:refnum<vi>)
      n53 = control-ref of="AppLoad 4"() -> (w125:refnum<vi>)
      n54 = control-ref of="Multipoint"() -> (w124:refnum<vi>)
      n55 = control-ref of="com 3"() -> (w120:refnum<vi>)
      n56 = control-ref of="com"() -> (w119:refnum<vi>)
      n57 = control-ref of="DecaForce COM Status"() -> (w118:refnum<vi>)
      n58 = control-ref of="Update"() -> (w117:refnum<vi>)
      n59 = control-ref of="Clear 3"() -> (w116:refnum<vi>)
      n60 = control-ref of="seq"() -> (w115:refnum<vi>)
      n61 = control-ref of="Stribeck table"() -> (w114:refnum<vi>)
      n62 = control-ref of="KiloForce"() -> (w106:refnum<vi>)
      n63 = control-ref of="DecaForce"() -> (w105:refnum<vi>)
      n64 = control-ref of="MicroForce"() -> (w104:refnum<vi>)
      n65 = control-ref of="LHBack"() -> (w103:refnum<vi>)
      n66 = control-ref of="LHNext"() -> (w102:refnum<vi>)
      n67 = control-ref of="Enter the Loading Rate (N/min)"() -> (w134:refnum<vi>)
      n68 = control-ref of="Enter the Final Load (N)"() -> (w111:refnum<vi>)
      n69 = control-ref of="Enter the CoF Trip"() -> (w110:refnum<vi>)
      n70 = control-ref of="Enter the Friction Force Trip"() -> (w109:refnum<vi>)
      n71 = control-ref of="Enter the Normal load Trip"() -> (w108:refnum<vi>)
      n72 = control-ref of="Enter the Load  (N)"() -> (w107:refnum<vi>)
      n73 = control-ref of="Message"() -> (w133:refnum<vi>)
      n74 = control-ref of="Indentation"() -> (w123:refnum<vi>)
      n75 = control-ref of="Stribeck Table  For loading"() -> (w113:refnum<vi>)
      n76 = control-ref of="Reference Sample"() -> (w122:refnum<vi>)
      n77 = control-ref of="Load Cell Communication Slide"() -> (w121:refnum<vi>)
      n78 = control-ref of="Loading Mode"() -> (w112:refnum<vi>)
      n79 = Bundle By Name(cluster=w136, "Loading.Enter the Loading Rate (N/min)"=w134, "Loading.Message"=w133, "Loading.Warning 2"=w132, "Loading.SSP 0.75"=w131, "Loading.SSP 0.5"=w130, "Loading.SSP 0.3"=w129, "Loading.Warning"=w128, "Loading.gui GIF"=w127, "Loading.Communication is established"=w126, "Loading.AppLoad 4"=w125, "Loading.Multipoint"=w124, "Loading.Indentation"=w123, "Loading.Reference Sample"=w122, "Loading.Load Cell Communication Slide"=w121, "Loading.com 3"=w120, "Loading.com"=w119, "Loading.DecaForce COM Status"=w118, "Loading.Update"=w117, "Loading.Clear 3"=w116, "Loading.seq"=w115, "Loading.Stribeck table"=w114, "Loading.Stribeck Table  For loading"=w113, "Loading.Loading Mode"=w112, "Loading.Enter the Final Load (N)"=w111, "Loading.Enter the CoF Trip"=w110, "Loading.Enter the Friction Force Trip"=w109, "Loading.Enter the Normal load Trip"=w108, "Loading.Enter the Load  (N)"=w107, "Loading.KiloForce"=w106, "Loading.DecaForce"=w105, "Loading.MicroForce"=w104, "Loading.LHBack"=w103, "Loading.LHNext"=w102, "Loading.Load Selection"=w101) -> (w135:T11)
    }
    frame #5 {
      n80 = control-ref of="TEST SELECTION"() -> (w187:refnum<vi>)
      n81 = control-ref of="SPEED SELECTION :"() -> (w186:refnum<vi>)
      n82 = control-ref of="SPEED SELECTION : rotary"() -> (w153:refnum<vi>)
      n83 = control-ref of="Rotary Tab"() -> (w202:refnum<vi>)
      n84 = control-ref of="e.v/ssr 2"() -> (w199:refnum<vi>)
      n85 = control-ref of="Step Speed"() -> (w183:refnum<vi>)
      n86 = control-ref of="M3 Image"() -> (w178:refnum<vi>)
      n87 = control-ref of="Rotary Module Selection"() -> (w155:refnum<vi>)
      n88 = control-ref of="zNL"() -> (w204:refnum<vi>)
      n89 = control-ref of="E.Velocity 2"() -> (w200:refnum<vi>)
      n90 = control-ref of="Ramp Up 2"() -> (w188:refnum<vi>)
      n91 = control-ref of="Angular Oscillation Set"() -> (w185:refnum<vi>)
      n92 = control-ref of="Traction"() -> (w184:refnum<vi>)
      n93 = control-ref of="Surge Forward MM"() -> (w180:refnum<vi>)
      n94 = control-ref of="Surge Backward MM"() -> (w179:refnum<vi>)
      n95 = control-ref of="Sway Left MM"() -> (w176:refnum<vi>)
      n96 = control-ref of="Sway Right MM"() -> (w175:refnum<vi>)
      n97 = control-ref of="Disable Axis Jog Soft Limits"() -> (w174:refnum<vi>)
      n98 = control-ref of="Heave Down MM"() -> (w172:refnum<vi>)
      n99 = control-ref of="Heave Up MM"() -> (w171:refnum<vi>)
      n100 = control-ref of="Set WTD"() -> (w169:refnum<vi>)
      n101 = control-ref of="HomeScratch"() -> (w168:refnum<vi>)
      n102 = control-ref of="HomeRot"() -> (w167:refnum<vi>)
      n103 = control-ref of="PlaceModule"() -> (w166:refnum<vi>)
      n104 = control-ref of="LR Sway"() -> (w162:refnum<vi>)
      n105 = control-ref of="Rot Hor"() -> (w161:refnum<vi>)
      n106 = control-ref of="Scratch"() -> (w160:refnum<vi>)
      n107 = control-ref of="LR Cam"() -> (w159:refnum<vi>)
      n108 = control-ref of="MMBack"() -> (w158:refnum<vi>)
      n109 = control-ref of="MMNext"() -> (w157:refnum<vi>)
      n110 = control-ref of="Rot Ver"() -> (w156:refnum<vi>)
      n111 = control-ref of="calculate rotary"() -> (w154:refnum<vi>)
      n112 = control-ref of="Import 2"() -> (w152:refnum<vi>)
      n113 = control-ref of="Save 2"() -> (w151:refnum<vi>)
      n114 = control-ref of="SwaySpeed Set"() -> (w144:refnum<vi>)
      n115 = control-ref of="HomeScratch"() -> (w140:refnum<vi>)
      n116 = control-ref of="Enter Scratch length (mm):"() -> (w139:refnum<vi>)
      n117 = control-ref of="NL disp"() -> (w203:refnum<vi>)
      n118 = control-ref of="Enter Fixed E.Velocity 2"() -> (w198:refnum<vi>)
      n119 = control-ref of="Enter Final SRR 2"() -> (w197:refnum<vi>)
      n120 = control-ref of="Enter initial SRR 2"() -> (w196:refnum<vi>)
      n121 = control-ref of="Enter Fixed SRR 2"() -> (w195:refnum<vi>)
      n122 = control-ref of="Enter the Final E.Velocity (m/s) 2"() -> (w194:refnum<vi>)
      n123 = control-ref of="Enter initial E.Velocity (m/s) 2"() -> (w193:refnum<vi>)
      n124 = control-ref of="Final Speed (RPM) 3"() -> (w192:refnum<vi>)
      n125 = control-ref of="Initial Speed (RPM) 2"() -> (w191:refnum<vi>)
      n126 = control-ref of="Enter the Final Velocity (m/s) 3"() -> (w190:refnum<vi>)
      n127 = control-ref of="Enter initial Velocity (m/s)  3"() -> (w189:refnum<vi>)
      n128 = control-ref of="mm"() -> (w173:refnum<vi>)
      n129 = control-ref of="Wear Track Diameter (mm)"() -> (w170:refnum<vi>)
      n130 = control-ref of="Enter the Angle (Deg)"() -> (w165:refnum<vi>)
      n131 = control-ref of="Enter the Frequency (Hz)"() -> (w164:refnum<vi>)
      n132 = control-ref of="Wear Track Diameter"() -> (w138:refnum<vi>)
      n133 = control-ref of="Enter the Speed(mm/sec)"() -> (w147:refnum<vi>)
      n134 = control-ref of="Enter the Speed (RPM)"() -> (w146:refnum<vi>)
      n135 = control-ref of="Enter Scratch Speed (mm/s):"() -> (w145:refnum<vi>)
      n136 = control-ref of="Scartch Offset"() -> (w143:refnum<vi>)
      n137 = control-ref of="String 39"() -> (w177:refnum<vi>)
      n138 = control-ref of="Rotary Speed Exced"() -> (w137:refnum<vi>)
      n139 = control-ref of="String 45"() -> (w149:refnum<vi>)
      n140 = control-ref of="StepTable For Load-Speed"() -> (w182:refnum<vi>)
      n141 = control-ref of="StepTable For Speed"() -> (w181:refnum<vi>)
      n142 = control-ref of="Motion Direction:  3"() -> (w201:refnum<vi>)
      n143 = control-ref of="Motion Mode:"() -> (w163:refnum<vi>)
      n144 = control-ref of="StepTable For Speed 3"() -> (w148:refnum<vi>)
      n145 = control-ref of="Scratch Mode:"() -> (w142:refnum<vi>)
      n146 = control-ref of="Motion type:"() -> (w141:refnum<vi>)
      n147 = control-ref of="File Path :  2"() -> (w150:refnum<vi>)
      n148 = Bundle By Name(cluster=w206, "Motion Module.zNL"=w204, "Motion Module.NL disp"=w203, "Motion Module.Rotary Tab"=w202, "Motion Module.Motion Direction:  3"=w201, "Motion Module.E.Velocity 2"=w200, "Motion Module.e.v/ssr 2"=w199, "Motion Module.Enter Fixed E.Velocity 2"=w198, "Motion Module.Enter Final SRR 2"=w197, "Motion Module.Enter initial SRR 2"=w196, "Motion Module.Enter Fixed SRR 2"=w195, "Motion Module.Enter the Final E.Velocity (m/s) 2"=w194, "Motion Module.Enter initial E.Velocity (m/s) 2"=w193, "Motion Module.Final Speed (RPM) 3"=w192, "Motion Module.Initial Speed (RPM) 2"=w191, "Motion Module.Enter the Final Velocity (m/s) 3"=w190, "Motion Module.Enter initial Velocity (m/s)  3"=w189, "Motion Module.Ramp Up 2"=w188, "Motion Module.TEST SELECTION"=w187, "Motion Module.SPEED SELECTION :"=w186, "Motion Module.Angular Oscillation Set"=w185, "Motion Module.Traction"=w184, "Motion Module.Step Speed"=w183, "Motion Module.StepTable For Load-Speed"=w182, "Motion Module.StepTable For Speed"=w181, "Motion Module.Surge Forward MM"=w180, "Motion Module.Surge Backward MM"=w179, "Motion Module.M3 Image"=w178, "Motion Module.String 39"=w177, "Motion Module.Sway Left MM"=w176, "Motion Module.Sway Right MM"=w175, "Motion Module.Disable Axis Jog Soft Limits"=w174, "Motion Module.mm"=w173, "Motion Module.Heave Down MM"=w172, "Motion Module.Heave Up MM"=w171, "Motion Module.Wear Track Diameter (mm)"=w170, "Motion Module.Set WTD"=w169, "Motion Module.HomeScratch"=w168, "Motion Module.HomeRot"=w167, "Motion Module.PlaceModule"=w166, "Motion Module.Enter the Angle (Deg)"=w165, "Motion Module.Enter the Frequency (Hz)"=w164, "Motion Module.Motion Mode:"=w163, "Motion Module.LR Sway"=w162, "Motion Module.Rot Hor"=w161, "Motion Module.Scratch"=w160, "Motion Module.LR Cam"=w159, "Motion Module.MMBack"=w158, "Motion Module.MMNext"=w157, "Motion Module.Rot Ver"=w156, "Motion Module.Rotary Module Selection"=w155, "Motion Module.calculate rotary"=w154, "Motion Module.SPEED SELECTION : rotary"=w153, "Motion Module.Import 2"=w152, "Motion Module.Save 2"=w151, "Motion Module.File Path :  2"=w150, "Motion Module.String 45"=w149, "Motion Module.StepTable For Speed 3"=w148, "Motion Module.Enter the Speed(mm/sec)"=w147, "Motion Module.Enter the Speed(RPM)"=w146, "Motion Module.Enter Scratch Speed (mm/s):"=w145, "Motion Module.SwaySpeed Set"=w144, "Motion Module.Scartch Offset"=w143, "Motion Module.Scratch Mode:"=w142, "Motion Module.Motion type:"=w141, "Motion Module.HomeScratch 2"=w140, "Motion Module.Enter Scratch length (mm):"=w139, "Motion Module.Wear Track Diameter"=w138, "Motion Module.Rotary Speed Exced"=w137) -> (w205:T11)
    }
    frame #6 {
      n149 = control-ref of="Add to list"() -> (w224:refnum<vi>)
      n150 = control-ref of="Wear"() -> (w223:refnum<vi>)
      n151 = control-ref of="Vibration"() -> (w222:refnum<vi>)
      n152 = control-ref of="Humidity (Chamber)"() -> (w221:refnum<vi>)
      n153 = control-ref of="Temperature (Chamber)"() -> (w220:refnum<vi>)
      n154 = control-ref of="ECR"() -> (w219:refnum<vi>)
      n155 = control-ref of="Temperature (Amb)"() -> (w218:refnum<vi>)
      n156 = control-ref of="Microphone"() -> (w217:refnum<vi>)
      n157 = control-ref of="Acoustic Emission 3"() -> (w216:refnum<vi>)
      n158 = control-ref of="SNext"() -> (w215:refnum<vi>)
      n159 = control-ref of="APBack"() -> (w214:refnum<vi>)
      n160 = control-ref of="Low Temp"() -> (w210:refnum<vi>)
      n161 = control-ref of="High Temp"() -> (w209:refnum<vi>)
      n162 = control-ref of="Humidity"() -> (w208:refnum<vi>)
      n163 = control-ref of="Humidity  Status  3"() -> (w231:refnum<vi>)
      n164 = control-ref of="Low Temp  Status  2"() -> (w230:refnum<vi>)
      n165 = control-ref of="TK4 status 2"() -> (w229:refnum<vi>)
      n166 = control-ref of="Humidity (Amb)"() -> (w226:refnum<vi>)
      n167 = control-ref of="Clear List"() -> (w225:refnum<vi>)
      n168 = control-ref of="Enter the Temperature (°C):"() -> (w213:refnum<vi>)
      n169 = control-ref of="Enter the Stage \nTemperature (°C):"() -> (w212:refnum<vi>)
      n170 = control-ref of="Enter the Humidity (%Rh):"() -> (w211:refnum<vi>)
      n171 = control-ref of="Sensors Picked"() -> (w207:refnum<vi>)
      n172 = control-ref of="Stage Temperature"() -> (w228:refnum<vi>)
      n173 = control-ref of="Sample Temperature"() -> (w227:refnum<vi>)
      n174 = Bundle By Name(cluster=w233, "Environmental control.Humidity  Status  3"=w231, "Environmental control.Low Temp  Status  2"=w230, "Environmental control.TK4 status 2"=w229, "Environmental control.Stage Temperature"=w228, "Environmental control.Sample Temperature"=w227, "Environmental control.Humidity (Amb)"=w226, "Environmental control.Clear List"=w225, "Environmental control.Add to list"=w224, "Environmental control.Wear"=w223, "Environmental control.Vibration"=w222, "Environmental control.Humidity (Chamber)"=w221, "Environmental control.Temperature (Chamber)"=w220, "Environmental control.ECR"=w219, "Environmental control.Temperature (Amb)"=w218, "Environmental control.Microphone"=w217, "Environmental control.Acoustic Emission 3"=w216, "Environmental control.SNext"=w215, "Environmental control.APBack"=w214, "Environmental control.Enter the Temperature (°C):"=w213, "Environmental control.Enter the Stage \nTemperature (°C):"=w212, "Environmental control.Enter the Humidity (%Rh):"=w211, "Environmental control.Low Temp"=w210, "Environmental control.High Temp"=w209, "Environmental control.Humidity"=w208, "Environmental control.Sensors Picked"=w207) -> (w232:T11)
    }
    frame #7 {
      n175 = control-ref of="ECR Port:"() -> (w243:refnum<vi>)
      n176 = control-ref of="Ramp Port:"() -> (w242:refnum<vi>)
      n177 = control-ref of="Heave and Surge COM Port:"() -> (w239:refnum<vi>)
      n178 = control-ref of="Sway COM Port:"() -> (w238:refnum<vi>)
      n179 = control-ref of="Temp Modbus:"() -> (w237:refnum<vi>)
      n180 = control-ref of="Humidity Port:"() -> (w236:refnum<vi>)
      n181 = control-ref of="About Tab"() -> (w244:refnum<vi>)
      n182 = control-ref of="Home Service"() -> (w246:refnum<vi>)
      n183 = control-ref of="Advanced Setting"() -> (w245:refnum<vi>)
      n184 = control-ref of="Installation/Replacement completed"() -> (w241:refnum<vi>)
      n185 = control-ref of="Loahead"() -> (w240:refnum<vi>)
      n186 = control-ref of="Edit Gain Constants"() -> (w235:refnum<vi>)
      n187 = control-ref of="Save Gain Constants"() -> (w234:refnum<vi>)
      n188 = control-ref of="Password"() -> (w247:refnum<vi>)
      n189 = Bundle By Name(cluster=w249, "About Screen.Password"=w247, "About Screen.Home Service"=w246, "About Screen.Advanced Setting"=w245, "About Screen.About Tab"=w244, "About Screen.ECR Port:"=w243, "About Screen.Ramp Port:"=w242, "About Screen.Installation/Replacement completed"=w241, "About Screen.Loahead"=w240, "About Screen.Heave and Surge COM Port:"=w239, "About Screen.Sway COM Port:"=w238, "About Screen.Temp Modbus:"=w237, "About Screen.Humidity Port:"=w236, "About Screen.Edit Gain Constants"=w235, "About Screen.Save Gain Constants"=w234) -> (w248:T11)
    }
    frame #8 {
      n190 = control-ref of="Cyclic Friction Force (N) Graph"() -> (w257:refnum<vi>)
      n191 = control-ref of="Cyclic Coefficient of Friction"() -> (w256:refnum<vi>)
      n192 = control-ref of="SDGp"() -> (w305:refnum<vi>)
      n193 = control-ref of="HumrGp"() -> (w303:refnum<vi>)
      n194 = control-ref of="gACQUOS"() -> (w300:refnum<vi>)
      n195 = control-ref of="ECR"() -> (w298:refnum<vi>)
      n196 = control-ref of="Temperature (deg c)"() -> (w296:refnum<vi>)
      n197 = control-ref of="MTM DISC  SPEED"() -> (w293:refnum<vi>)
      n198 = control-ref of="MTM BALL SPEED"() -> (w292:refnum<vi>)
      n199 = control-ref of="speed mm/sec"() -> (w291:refnum<vi>)
      n200 = control-ref of="WearGp"() -> (w281:refnum<vi>)
      n201 = control-ref of="Main Chart 3"() -> (w275:refnum<vi>)
      n202 = control-ref of="Friction Force (N) Graph"() -> (w263:refnum<vi>)
      n203 = control-ref of="Coefficient of Friction"() -> (w262:refnum<vi>)
      n204 = control-ref of="Main Screen Tab"() -> (w364:refnum<vi>)
      n205 = control-ref of="Angle and Frequency"() -> (w363:refnum<vi>)
      n206 = control-ref of="Main Speed Tab"() -> (w360:refnum<vi>)
      n207 = control-ref of="MTM MOTOR DISPLAY"() -> (w359:refnum<vi>)
      n208 = control-ref of="SPEED TAB"() -> (w354:refnum<vi>)
      n209 = control-ref of="Time Tab"() -> (w349:refnum<vi>)
      n210 = control-ref of="Temp Tabs"() -> (w342:refnum<vi>)
      n211 = control-ref of="Grp Tab"() -> (w309:refnum<vi>)
      n212 = control-ref of="Sub Graph"() -> (w308:refnum<vi>)
      n213 = control-ref of="Speed Tab"() -> (w294:refnum<vi>)
      n214 = control-ref of="FF Tab"() -> (w260:refnum<vi>)
      n215 = control-ref of="CZ FF"() -> (w258:refnum<vi>)
      n216 = control-ref of="Cyclic FF Disable Trip"() -> (w254:refnum<vi>)
      n217 = control-ref of="cyclic COF Disable Trip"() -> (w253:refnum<vi>)
      n218 = control-ref of="cyclic COF Reset Graph"() -> (w251:refnum<vi>)
      n219 = control-ref of="Cyclic FF Reset Graph"() -> (w250:refnum<vi>)
      n220 = control-ref of="Scratch Start Test"() -> (w261:refnum<vi>)
      n221 = control-ref of="Heater"() -> (w341:refnum<vi>)
      n222 = control-ref of="TK4 status"() -> (w340:refnum<vi>)
      n223 = control-ref of="Controller  Status"() -> (w337:refnum<vi>)
      n224 = control-ref of="Cooling"() -> (w334:refnum<vi>)
      n225 = control-ref of="Load Communication"() -> (w333:refnum<vi>)
      n226 = control-ref of="HumCOMStatus"() -> (w331:refnum<vi>)
      n227 = control-ref of="Load En"() -> (w328:refnum<vi>)
      n228 = control-ref of="NLt"() -> (w327:refnum<vi>)
      n229 = control-ref of="zNL 2"() -> (w326:refnum<vi>)
      n230 = control-ref of="Humidity On"() -> (w325:refnum<vi>)
      n231 = control-ref of="AppLoadSeq scratch"() -> (w321:refnum<vi>)
      n232 = control-ref of="Stop Scratch"() -> (w320:refnum<vi>)
      n233 = control-ref of="ClrLog"() -> (w319:refnum<vi>)
      n234 = control-ref of="STOP"() -> (w317:refnum<vi>)
      n235 = control-ref of="Start Test"() -> (w316:refnum<vi>)
      n236 = control-ref of="Test status"() -> (w315:refnum<vi>)
      n237 = control-ref of="AR Led"() -> (w314:refnum<vi>)
      n238 = control-ref of="Data"() -> (w313:refnum<vi>)
      n239 = control-ref of="Health"() -> (w312:refnum<vi>)
      n240 = control-ref of="Sway COM Status"() -> (w311:refnum<vi>)
      n241 = control-ref of="Heave COM Status"() -> (w310:refnum<vi>)
      n242 = control-ref of="Siliding distance Reset Graph"() -> (w306:refnum<vi>)
      n243 = control-ref of="Humidity Reset Graph"() -> (w304:refnum<vi>)
      n244 = control-ref of="Aqucostic Reset Graph"() -> (w301:refnum<vi>)
      n245 = control-ref of="ECR RESET"() -> (w299:refnum<vi>)
      n246 = control-ref of="Temperature Reset"() -> (w297:refnum<vi>)
      n247 = control-ref of="Speed Reset Graph"() -> (w295:refnum<vi>)
      n248 = control-ref of="Hymidity"() -> (w290:refnum<vi>)
      n249 = control-ref of="Humidity Disable trip"() -> (w289:refnum<vi>)
      n250 = control-ref of="Weart Deapth"() -> (w286:refnum<vi>)
      n251 = control-ref of="Depth Reset Graph"() -> (w285:refnum<vi>)
      n252 = control-ref of="Weart"() -> (w284:refnum<vi>)
      n253 = control-ref of="Depthz"() -> (w283:refnum<vi>)
      n254 = control-ref of="Load pid"() -> (w279:refnum<vi>)
      n255 = control-ref of="Load Disable Trip"() -> (w278:refnum<vi>)
      n256 = control-ref of="Load Reset Graph"() -> (w277:refnum<vi>)
      n257 = control-ref of="BACK"() -> (w274:refnum<vi>)
      n258 = control-ref of="zFF"() -> (w264:refnum<vi>)
      n259 = control-ref of="FF Reset Graph"() -> (w270:refnum<vi>)
      n260 = control-ref of="FF Disable Trip"() -> (w269:refnum<vi>)
      n261 = control-ref of="COF Disable Trip"() -> (w267:refnum<vi>)
      n262 = control-ref of="COF Reset Graph"() -> (w266:refnum<vi>)
      n263 = control-ref of="Start Test Temp"() -> (w265:refnum<vi>)
      n264 = control-ref of="Depth Trip"() -> (w273:refnum<vi>)
      n265 = control-ref of="Cyclic Friction Force (N)"() -> (w259:refnum<vi>)
      n266 = control-ref of="Cyclic FF TRIP"() -> (w255:refnum<vi>)
      n267 = control-ref of="cyclic COF TRIP"() -> (w252:refnum<vi>)
      n268 = control-ref of="Stroke (mm)"() -> (w362:refnum<vi>)
      n269 = control-ref of="Angle (Deg)"() -> (w361:refnum<vi>)
      n270 = control-ref of="Disc Speed (m/sec)"() -> (w358:refnum<vi>)
      n271 = control-ref of="Ball Speed (m/sec)"() -> (w357:refnum<vi>)
      n272 = control-ref of="Disc Speed (RPM)"() -> (w356:refnum<vi>)
      n273 = control-ref of="Ball Speed (RPM)"() -> (w355:refnum<vi>)
      n274 = control-ref of="Speed (m/sec)"() -> (w353:refnum<vi>)
      n275 = control-ref of="Set Speed (m/sec)"() -> (w352:refnum<vi>)
      n276 = control-ref of="Speed (RPM)"() -> (w351:refnum<vi>)
      n277 = control-ref of="Set Speed"() -> (w350:refnum<vi>)
      n278 = control-ref of="Time ( HH:MM:SS ) 2"() -> (w348:refnum<vi>)
      n279 = control-ref of="Test Duration"() -> (w347:refnum<vi>)
      n280 = control-ref of="Test Duration 4"() -> (w346:refnum<vi>)
      n281 = control-ref of="TEST CYCLE"() -> (w345:refnum<vi>)
      n282 = control-ref of="TOTAL CYCLES"() -> (w344:refnum<vi>)
      n283 = control-ref of="Set Load (N)"() -> (w343:refnum<vi>)
      n284 = control-ref of="ChamberTemp"() -> (w339:refnum<vi>)
      n285 = control-ref of="SetTmp"() -> (w338:refnum<vi>)
      n286 = control-ref of="ChamberTemp"() -> (w336:refnum<vi>)
      n287 = control-ref of="SetTmp"() -> (w335:refnum<vi>)
      n288 = control-ref of="Ambient \nTemperature"() -> (w332:refnum<vi>)
      n289 = control-ref of="Ambient\n Humidity"() -> (w330:refnum<vi>)
      n290 = control-ref of="Freq (Hz)"() -> (w329:refnum<vi>)
      n291 = control-ref of="humidity disp"() -> (w324:refnum<vi>)
      n292 = control-ref of="Set Humidity"() -> (w323:refnum<vi>)
      n293 = control-ref of="NL disp 2"() -> (w322:refnum<vi>)
      n294 = control-ref of="SD (mm)"() -> (w307:refnum<vi>)
      n295 = control-ref of="Acoustic Emission (mV)"() -> (w302:refnum<vi>)
      n296 = control-ref of="CoF Trip  2"() -> (w288:refnum<vi>)
      n297 = control-ref of="Depth Trip"() -> (w287:refnum<vi>)
      n298 = control-ref of="Depth (µm)"() -> (w282:refnum<vi>)
      n299 = control-ref of="NL Trip 2"() -> (w280:refnum<vi>)
      n300 = control-ref of="NL Display 4"() -> (w276:refnum<vi>)
      n301 = control-ref of="COF TRIP"() -> (w272:refnum<vi>)
      n302 = control-ref of="Friction Force (N)"() -> (w271:refnum<vi>)
      n303 = control-ref of="FF TRIP"() -> (w268:refnum<vi>)
      n304 = control-ref of="Trip Log"() -> (w318:refnum<vi>)
      n305 = Bundle By Name(cluster=w366, "Main Screen.Main Screen Tab"=w364, "Main Screen.Angle and Frequency"=w363, "Main Screen.Stroke (mm)"=w362, "Main Screen.Angle (Deg)"=w361, "Main Screen.Main Speed Tab"=w360, "Main Screen.MTM MOTOR DISPLAY"=w359, "Main Screen.Disc Speed (m/sec)"=w358, "Main Screen.Ball Speed (m/sec)"=w357, "Main Screen.Disc Speed (RPM)"=w356, "Main Screen.Ball Speed (RPM)"=w355, "Main Screen.SPEED TAB"=w354, "Main Screen.Speed (m/sec)"=w353, "Main Screen.Set Speed (m/sec)"=w352, "Main Screen.Speed (RPM)"=w351, "Main Screen.Set Speed"=w350, "Main Screen.Time Tab"=w349, "Main Screen.Time ( HH:MM:SS ) 2"=w348, "Main Screen.Test Duration"=w347, "Main Screen.Test Duration 4"=w346, "Main Screen.TEST CYCLE"=w345, "Main Screen.TOTAL CYCLES"=w344, "Main Screen.Set Load (N)"=w343, "Main Screen.Temp Tabs"=w342, "Main Screen.Heater"=w341, "Main Screen.TK4 status"=w340, "Main Screen.ChamberTemp"=w339, "Main Screen.SetTmp"=w338, "Main Screen.Controller  Status"=w337, "Main Screen.ChamberTemp 2"=w336, "Main Screen.SetTmp 2"=w335, "Main Screen.Cooling"=w334, "Main Screen.Load Communication"=w333, "Main Screen.Ambient \nTemperature"=w332, "Main Screen.HumCOMStatus"=w331, "Main Screen.Ambient\n Humidity"=w330, "Main Screen.Freq (Hz)"=w329, "Main Screen.Load En"=w328, "Main Screen.NLt"=w327, "Main Screen.zNL 2"=w326, "Main Screen.Humidity On"=w325, "Main Screen.humidity disp"=w324, "Main Screen.Set Humidity"=w323, "Main Screen.NL disp 2"=w322, "Main Screen.AppLoadSeq scratch"=w321, "Main Screen.Stop Scratch"=w320, "Main Screen.ClrLog"=w319, "Main Screen.Trip Log"=w318, "Main Screen.STOP"=w317, "Main Screen.Start Test"=w316, "Main Screen.Test status"=w315, "Main Screen.AR Led"=w314, "Main Screen.Data"=w313, "Main Screen.Health"=w312, "Main Screen.Sway COM Status"=w311, "Main Screen.Heave COM Status"=w310, "Main Screen.Grp Tab"=w309, "Main Screen.Sub Graph"=w308, "Main Screen.SD (mm)"=w307, "Main Screen.Siliding distance Reset Graph"=w306, "Main Screen.SDGp"=w305, "Main Screen.Humidity Reset Graph"=w304, "Main Screen.HumrGp"=w303, "Main Screen.Acoustic Emission (mV)"=w302, "Main Screen.Aqucostic Reset Graph"=w301, "Main Screen.gACQUOS"=w300, "Main Screen.ECR RESET"=w299, "Main Screen.ECR"=w298, "Main Screen.Temperature Reset"=w297, "Main Screen.Temperature (deg c)"=w296, "Main Screen.Speed Reset Graph"=w295, "Main Screen.Speed Tab"=w294, "Main Screen.MTM DISC  SPEED"=w293, "Main Screen.MTM BALL SPEED"=w292, "Main Screen.speed mm/sec"=w291, "Main Screen.Hymidity"=w290, "Main Screen.Humidity Disable trip"=w289, "Main Screen.CoF Trip  2"=w288, "Main Screen.Depth Trip"=w287, "Main Screen.Weart Deapth"=w286, "Main Screen.Depth Reset Graph"=w285, "Main Screen.Weart"=w284, "Main Screen.Depthz"=w283, "Main Screen.Depth (µm)"=w282, "Main Screen.WearGp"=w281, "Main Screen.NL Trip 2"=w280, "Main Screen.Load pid"=w279, "Main Screen.Load Disable Trip"=w278, "Main Screen.Load Reset Graph"=w277, "Main Screen.NL Display 4"=w276, "Main Screen.Main Chart 3"=w275, "Main Screen.BACK"=w274, "Main Screen.Depth Trip 2"=w273, "Main Screen.COF TRIP"=w272, "Main Screen.Friction Force (N)"=w271, "Main Screen.FF Reset Graph"=w270, "Main Screen.FF Disable Trip"=w269, "Main Screen.FF TRIP"=w268, "Main Screen.COF Disable Trip"=w267, "Main Screen.COF Reset Graph"=w266, "Main Screen.FF Tab"=w260, "Main Screen.Start Test Temp"=w265, "Main Screen.zFF"=w264, "Main Screen.Friction Force (N) Graph"=w263, "Main Screen.Coefficient of Friction"=w262, "Main Screen.Scratch Start Test"=w261, "Main Screen.Cyclic Friction Force (N)"=w259, "Main Screen.CZ FF"=w258, "Main Screen.Cyclic Friction Force (N) Graph"=w257, "Main Screen.Cyclic Coefficient of Friction"=w256, "Main Screen.Cyclic FF TRIP"=w255, "Main Screen.Cyclic FF Disable Trip"=w254, "Main Screen.cyclic COF Disable Trip"=w253, "Main Screen.cyclic COF TRIP"=w252, "Main Screen.cyclic COF Reset Graph"=w251, "Main Screen.Cyclic FF Reset Graph"=w250) -> (w365:T11)
    }
    frame #9 {
      n306 = control-ref of="gFF Rot 7"() -> (w370:refnum<vi>)
      n307 = control-ref of="Ramp"() -> (w389:refnum<vi>)
      n308 = control-ref of="Dummy Run"() -> (w383:refnum<vi>)
      n309 = control-ref of="AutoTune"() -> (w381:refnum<vi>)
      n310 = control-ref of="apply load"() -> (w379:refnum<vi>)
      n311 = control-ref of="reinit 3"() -> (w377:refnum<vi>)
      n312 = control-ref of="Bypass Load"() -> (w374:refnum<vi>)
      n313 = control-ref of="PID gains out delay (microForce)"() -> (w390:refnum<vi>)
      n314 = control-ref of="output range delay"() -> (w376:refnum<vi>)
      n315 = control-ref of="PID gains out delay"() -> (w375:refnum<vi>)
      n316 = control-ref of="Ramp MulFac"() -> (w394:refnum<vi>)
      n317 = control-ref of="pulses LoadDiffRamp(2..10)"() -> (w393:refnum<vi>)
      n318 = control-ref of="PulseControlRamp(diff<=3N)"() -> (w392:refnum<vi>)
      n319 = control-ref of="SetLoadDeadband(%) Load(0-10N)"() -> (w391:refnum<vi>)
      n320 = control-ref of="Gain 2"() -> (w388:refnum<vi>)
      n321 = control-ref of="pulses LoadDiff(2..10)"() -> (w387:refnum<vi>)
      n322 = control-ref of="pulses LoadDiff(11..50)"() -> (w386:refnum<vi>)
      n323 = control-ref of="PulseControl(diff<=3N)"() -> (w385:refnum<vi>)
      n324 = control-ref of="SetLoadDeadband(%)  2"() -> (w384:refnum<vi>)
      n325 = control-ref of="Vertical load (N)"() -> (w382:refnum<vi>)
      n326 = control-ref of="Offset  3"() -> (w380:refnum<vi>)
      n327 = control-ref of="Enter ByPass Load"() -> (w378:refnum<vi>)
      n328 = control-ref of="pulsesSent"() -> (w373:refnum<vi>)
      n329 = control-ref of="pulses"() -> (w372:refnum<vi>)
      n330 = control-ref of="actpid"() -> (w371:refnum<vi>)
      n331 = control-ref of="pulses LoadDiff(21..1000)"() -> (w369:refnum<vi>)
      n332 = control-ref of="Delay"() -> (w368:refnum<vi>)
      n333 = control-ref of="deadband"() -> (w367:refnum<vi>)
      n334 = Bundle By Name(cluster=w396, "PID.Ramp MulFac"=w394, "PID.pulses LoadDiffRamp(2..10)"=w393, "PID.PulseControlRamp(diff<=3N)"=w392, "PID.SetLoadDeadband(%) Load(0-10N)"=w391, "PID.PID gains out delay (microForce)"=w390, "PID.Ramp"=w389, "PID.Gain 2"=w388, "PID.pulses LoadDiff(2..10)"=w387, "PID.pulses LoadDiff(11..50)"=w386, "PID.PulseControl(diff<=3N)"=w385, "PID.SetLoadDeadband(%)  2"=w384, "PID.Dummy Run"=w383, "PID.Vertical load (N)"=w382, "PID.AutoTune"=w381, "PID.Offset 3"=w380, "PID.apply load"=w379, "PID.Enter ByPass Load"=w378, "PID.reinit 3"=w377, "PID.output range delay"=w376, "PID.PID gains out delay"=w375, "PID.Bypass Load"=w374, "PID.pulsesSent"=w373, "PID.pulses"=w372, "PID.actpid"=w371, "PID.gFF Rot"=w370, "PID.pulses LoadDiff(21..1000)"=w369, "PID.Delay"=w368, "PID.deadband"=w367) -> (w395:T11)
    }
    frame #10 {
      n335 = control-ref of="Tab Control 3"() -> (w447:refnum<vi>)
      n336 = control-ref of="Tab Control 19"() -> (w446:refnum<vi>)
      n337 = control-ref of="Tab Control 5"() -> (w407:refnum<vi>)
      n338 = control-ref of="Tab Control 14"() -> (w406:refnum<vi>)
      n339 = control-ref of="Tab Control 26"() -> (w405:refnum<vi>)
      n340 = control-ref of="Re-initilaize"() -> (w444:refnum<vi>)
      n341 = control-ref of="Filter ON/OFF"() -> (w443:refnum<vi>)
      n342 = control-ref of="Apply Filter (FF)"() -> (w439:refnum<vi>)
      n343 = control-ref of="Apply Filter (Load)"() -> (w437:refnum<vi>)
      n344 = control-ref of="SAVE  2"() -> (w432:refnum<vi>)
      n345 = control-ref of="Enter Distance"() -> (w431:refnum<vi>)
      n346 = control-ref of="AE"() -> (w404:refnum<vi>)
      n347 = control-ref of="Heave Loop Delay"() -> (w403:refnum<vi>)
      n348 = control-ref of="Heave PID Speed"() -> (w402:refnum<vi>)
      n349 = control-ref of="Surge Jog Speed"() -> (w401:refnum<vi>)
      n350 = control-ref of="Heave Jog Speed"() -> (w400:refnum<vi>)
      n351 = control-ref of="Sway Loop Delay"() -> (w399:refnum<vi>)
      n352 = control-ref of="Sway PID Speed"() -> (w398:refnum<vi>)
      n353 = control-ref of="Sway Jog Speed"() -> (w397:refnum<vi>)
      n354 = control-ref of="SAMPLES"() -> (w445:refnum<vi>)
      n355 = control-ref of="TracHomeSurgeOffsetCounts 10MM"() -> (w442:refnum<vi>)
      n356 = control-ref of="TracHomeSwayOffsetCounts 10MM"() -> (w441:refnum<vi>)
      n357 = control-ref of="Acoustic Emission:"() -> (w440:refnum<vi>)
      n358 = control-ref of="Filter% 2"() -> (w438:refnum<vi>)
      n359 = control-ref of="Filter%"() -> (w436:refnum<vi>)
      n360 = control-ref of="Sway distance (mm)"() -> (w435:refnum<vi>)
      n361 = control-ref of="Surge distance (mm)"() -> (w434:refnum<vi>)
      n362 = control-ref of="DataSavingLoopDelay(ms)"() -> (w433:refnum<vi>)
      n363 = control-ref of="Sway Counts:"() -> (w430:refnum<vi>)
      n364 = control-ref of="Distance (mm): 3"() -> (w429:refnum<vi>)
      n365 = control-ref of="Surge Counts:"() -> (w428:refnum<vi>)
      n366 = control-ref of="Distance (mm): 2"() -> (w427:refnum<vi>)
      n367 = control-ref of="Distance (mm):"() -> (w426:refnum<vi>)
      n368 = control-ref of="Heave Counts:"() -> (w425:refnum<vi>)
      n369 = control-ref of="LRMHomeSurgeOffsetCounts"() -> (w424:refnum<vi>)
      n370 = control-ref of="LRMHomeSwayOffsetCounts"() -> (w423:refnum<vi>)
      n371 = control-ref of="TracHomeSurgeOffsetCounts 20MM"() -> (w422:refnum<vi>)
      n372 = control-ref of="TracHomeSwayOffsetCounts 20MM"() -> (w421:refnum<vi>)
      n373 = control-ref of="RotHomeSwayOffsetCounts"() -> (w420:refnum<vi>)
      n374 = control-ref of="RotHomeSurgeOffsetCounts"() -> (w419:refnum<vi>)
      n375 = control-ref of="Heave distance"() -> (w418:refnum<vi>)
      n376 = control-ref of="Zmm"() -> (w417:refnum<vi>)
      n377 = control-ref of="Heave Pulses/mm"() -> (w416:refnum<vi>)
      n378 = control-ref of="Surge Pulses/mm"() -> (w415:refnum<vi>)
      n379 = control-ref of="Sway Pulses/mm"() -> (w414:refnum<vi>)
      n380 = control-ref of="Heave Pitch"() -> (w413:refnum<vi>)
      n381 = control-ref of="Surge Pitch"() -> (w412:refnum<vi>)
      n382 = control-ref of="Sway Pitch"() -> (w411:refnum<vi>)
      n383 = control-ref of="Heave PPR"() -> (w410:refnum<vi>)
      n384 = control-ref of="Surge PPR"() -> (w409:refnum<vi>)
      n385 = control-ref of="Sway PPR"() -> (w408:refnum<vi>)
      n386 = Bundle By Name(cluster=w449, "Config Parameters.Tab Control 3"=w447, "Config Parameters.Tab Control 19"=w446, "Config Parameters.SAMPLES"=w445, "Config Parameters.Re-initilaize"=w444, "Config Parameters.Filter ON/OFF"=w443, "Config Parameters.TracHomeSurgeOffsetCounts 10MM"=w442, "Config Parameters.TracHomeSwayOffsetCounts 10MM"=w441, "Config Parameters.Acoustic Emission:"=w440, "Config Parameters.Apply Filter (FF)"=w439, "Config Parameters.Filter% 2"=w438, "Config Parameters.Apply Filter (Load)"=w437, "Config Parameters.Filter%"=w436, "Config Parameters.Sway distance (mm)"=w435, "Config Parameters.Surge distance (mm)"=w434, "Config Parameters.DataSavingLoopDelay(ms)"=w433, "Config Parameters.SAVE 2"=w432, "Config Parameters.Enter Distance"=w431, "Config Parameters.Sway Counts:"=w430, "Config Parameters.Distance (mm): 3"=w429, "Config Parameters.Surge Counts:"=w428, "Config Parameters.Distance (mm): 2"=w427, "Config Parameters.Distance (mm):"=w426, "Config Parameters.Heave Counts:"=w425, "Config Parameters.LRMHomeSurgeOffsetCounts"=w424, "Config Parameters.LRMHomeSwayOffsetCounts"=w423, "Config Parameters.TracHomeSurgeOffsetCounts 20MM"=w422, "Config Parameters.TracHomeSwayOffsetCounts 20MM"=w421, "Config Parameters.RotHomeSwayOffsetCounts"=w420, "Config Parameters.RotHomeSurgeOffsetCounts"=w419, "Config Parameters.Heave distance"=w418, "Config Parameters.Zmm"=w417, "Config Parameters.Heave Pulses/mm"=w416, "Config Parameters.Surge Pulses/mm"=w415, "Config Parameters.Sway Pulses/mm"=w414, "Config Parameters.Heave Pitch"=w413, "Config Parameters.Surge Pitch"=w412, "Config Parameters.Sway Pitch"=w411, "Config Parameters.Heave PPR"=w410, "Config Parameters.Surge PPR"=w409, "Config Parameters.Sway PPR"=w408, "Config Parameters.Tab Control 5"=w407, "Config Parameters.Tab Control 14"=w406, "Config Parameters.Tab Control 26"=w405, "Config Parameters.AE"=w404, "Config Parameters.Heave Loop Delay"=w403, "Config Parameters.Heave PID Speed"=w402, "Config Parameters.Surge Jog Speed"=w401, "Config Parameters.Heave Jog Speed"=w400, "Config Parameters.Sway Loop Delay"=w399, "Config Parameters.Sway PID Speed"=w398, "Config Parameters.Sway Jog Speed"=w397) -> (w448:T11)
    }
    frame #11 {
      n387 = control-ref of="Mx"() -> (w479:refnum<vi>)
      n388 = control-ref of="My"() -> (w478:refnum<vi>)
      n389 = control-ref of="Mz"() -> (w477:refnum<vi>)
      n390 = control-ref of="Fx(N)"() -> (w476:refnum<vi>)
      n391 = control-ref of="Fy(N)"() -> (w475:refnum<vi>)
      n392 = control-ref of="Fz(N)"() -> (w474:refnum<vi>)
      n393 = control-ref of="Load Cell Temp"() -> (w450:refnum<vi>)
      n394 = control-ref of="ClearAll"() -> (w484:refnum<vi>)
      n395 = control-ref of="ZeroAll"() -> (w473:refnum<vi>)
      n396 = control-ref of="delete Handle"() -> (w463:refnum<vi>)
      n397 = control-ref of="Create Handle"() -> (w462:refnum<vi>)
      n398 = control-ref of="stop 6"() -> (w459:refnum<vi>)
      n399 = control-ref of="running_flag"() -> (w458:refnum<vi>)
      n400 = control-ref of="Save Dwell"() -> (w480:refnum<vi>)
      n401 = control-ref of="Acq Delay (ms)"() -> (w472:refnum<vi>)
      n402 = control-ref of="Burst Delay (ms)"() -> (w471:refnum<vi>)
      n403 = control-ref of="SN"() -> (w469:refnum<vi>)
      n404 = control-ref of="Port"() -> (w466:refnum<vi>)
      n405 = control-ref of="ft_udp_handle"() -> (w457:refnum<vi>)
      n406 = control-ref of="get-data-return"() -> (w456:refnum<vi>)
      n407 = control-ref of="get-range-return"() -> (w455:refnum<vi>)
      n408 = control-ref of="zero-return"() -> (w454:refnum<vi>)
      n409 = control-ref of="filter-return"() -> (w453:refnum<vi>)
      n410 = control-ref of="initial-return"() -> (w452:refnum<vi>)
      n411 = control-ref of="deleteHandle-result"() -> (w451:refnum<vi>)
      n412 = control-ref of="model"() -> (w470:refnum<vi>)
      n413 = control-ref of="Sensor IP"() -> (w467:refnum<vi>)
      n414 = control-ref of="Mz(Nm)"() -> (w483:refnum<vi>)
      n415 = control-ref of="My(Nm)"() -> (w482:refnum<vi>)
      n416 = control-ref of="Mx(Nm)"() -> (w481:refnum<vi>)
      n417 = control-ref of="FFx(N)"() -> (w468:refnum<vi>)
      n418 = control-ref of="FFy(N)"() -> (w465:refnum<vi>)
      n419 = control-ref of="Load(N)"() -> (w464:refnum<vi>)
      n420 = control-ref of="ft_data"() -> (w461:refnum<vi>)
      n421 = control-ref of="ft_range"() -> (w460:refnum<vi>)
      n422 = Bundle By Name(cluster=w486, "Loading Com Port.ClearAll"=w484, "Loading Com Port.Mz(Nm)"=w483, "Loading Com Port.My(Nm)"=w482, "Loading Com Port.Mx(Nm)"=w481, "Loading Com Port.Save Dwell"=w480, "Loading Com Port.Mx"=w479, "Loading Com Port.My"=w478, "Loading Com Port.Mz"=w477, "Loading Com Port.Fx(N)"=w476, "Loading Com Port.Fy(N)"=w475, "Loading Com Port.Fz(N)"=w474, "Loading Com Port.ZeroAll"=w473, "Loading Com Port.Acq Delay (ms)"=w472, "Loading Com Port.Burst Delay (ms)"=w471, "Loading Com Port.model"=w470, "Loading Com Port.SN"=w469, "Loading Com Port.FFx(N)"=w468, "Loading Com Port.Sensor IP"=w467, "Loading Com Port.Port"=w466, "Loading Com Port.FFy(N)"=w465, "Loading Com Port.Load(N)"=w464, "Loading Com Port.delete Handle"=w463, "Loading Com Port.Create Handle"=w462, "Loading Com Port.ft_data"=w461, "Loading Com Port.ft_range"=w460, "Loading Com Port.stop 6"=w459, "Loading Com Port.running_flag"=w458, "Loading Com Port.ft_udp_handle"=w457, "Loading Com Port.get-data-return"=w456, "Loading Com Port.get-range-return"=w455, "Loading Com Port.zero-return"=w454, "Loading Com Port.filter-return"=w453, "Loading Com Port.initial-return"=w452, "Loading Com Port.deleteHandle-result"=w451, "Loading Com Port.Load Cell Temp"=w450) -> (w485:T11)
    }
    frame #12 {
      n423 = control-ref of="Manual Write Heave & Surge"() -> (w488:refnum<vi>)
      n424 = control-ref of="Read Heave Temp"() -> (w511:refnum<vi>)
      n425 = control-ref of="error out Read"() -> (w523:refnum<vi>)
      n426 = control-ref of="error out Write"() -> (w518:refnum<vi>)
      n427 = control-ref of="SURGE POSE"() -> (w524:refnum<vi>)
      n428 = control-ref of="HEAVE POSE"() -> (w522:refnum<vi>)
      n429 = control-ref of="State"() -> (w521:refnum<vi>)
      n430 = control-ref of="Homed"() -> (w520:refnum<vi>)
      n431 = control-ref of="Sequence ID"() -> (w519:refnum<vi>)
      n432 = control-ref of="faultCode"() -> (w517:refnum<vi>)
      n433 = control-ref of="Ack ID"() -> (w516:refnum<vi>)
      n434 = control-ref of="SPEED"() -> (w515:refnum<vi>)
      n435 = control-ref of="Distance"() -> (w514:refnum<vi>)
      n436 = control-ref of="Mode Command"() -> (w513:refnum<vi>)
      n437 = control-ref of="SPARE 2"() -> (w510:refnum<vi>)
      n438 = control-ref of="SPARE 1"() -> (w509:refnum<vi>)
      n439 = control-ref of="Spare 15"() -> (w508:refnum<vi>)
      n440 = control-ref of="Spare 14"() -> (w507:refnum<vi>)
      n441 = control-ref of="Spare 13"() -> (w506:refnum<vi>)
      n442 = control-ref of="Spare 12"() -> (w505:refnum<vi>)
      n443 = control-ref of="Spare 11"() -> (w504:refnum<vi>)
      n444 = control-ref of="Spare 10"() -> (w503:refnum<vi>)
      n445 = control-ref of="Spare 9"() -> (w502:refnum<vi>)
      n446 = control-ref of="Spare 8"() -> (w501:refnum<vi>)
      n447 = control-ref of="Spare 7"() -> (w500:refnum<vi>)
      n448 = control-ref of="Spare 6"() -> (w499:refnum<vi>)
      n449 = control-ref of="Spare 5"() -> (w498:refnum<vi>)
      n450 = control-ref of="Spare 4"() -> (w497:refnum<vi>)
      n451 = control-ref of="Spare 3"() -> (w496:refnum<vi>)
      n452 = control-ref of="Spare 2"() -> (w495:refnum<vi>)
      n453 = control-ref of="Spare 1"() -> (w494:refnum<vi>)
      n454 = control-ref of="Node Id"() -> (w493:refnum<vi>)
      n455 = control-ref of="SPARE 3"() -> (w492:refnum<vi>)
      n456 = control-ref of="SPARE 4"() -> (w491:refnum<vi>)
      n457 = control-ref of="fwMajor"() -> (w490:refnum<vi>)
      n458 = control-ref of="fwMinor"() -> (w489:refnum<vi>)
      n459 = control-ref of="Heave and Surge Write"() -> (w487:refnum<vi>)
      n460 = control-ref of="Heave and Surge Read"() -> (w512:refnum<vi>)
      n461 = Bundle By Name(cluster=w526, "Heave AND Surge.SURGE POSE"=w524, "Heave AND Surge.error out Read"=w523, "Heave AND Surge.HEAVE POSE"=w522, "Heave AND Surge.State"=w521, "Heave AND Surge.Homed"=w520, "Heave AND Surge.Sequence ID"=w519, "Heave AND Surge.error out Write"=w518, "Heave AND Surge.faultCode"=w517, "Heave AND Surge.Ack ID"=w516, "Heave AND Surge.SPEED"=w515, "Heave AND Surge.Distance"=w514, "Heave AND Surge.Mode Command"=w513, "Heave AND Surge.Heave and Surge Read"=w512, "Heave AND Surge.Read Heave Temp"=w511, "Heave AND Surge.SPARE 2"=w510, "Heave AND Surge.SPARE 1"=w509, "Heave AND Surge.Spare 15"=w508, "Heave AND Surge.Spare 14"=w507, "Heave AND Surge.Spare 13"=w506, "Heave AND Surge.Spare 12"=w505, "Heave AND Surge.Spare 11"=w504, "Heave AND Surge.Spare 10"=w503, "Heave AND Surge.Spare 9"=w502, "Heave AND Surge.Spare 8"=w501, "Heave AND Surge.Spare 7"=w500, "Heave AND Surge.Spare 6"=w499, "Heave AND Surge.Spare 5"=w498, "Heave AND Surge.Spare 4"=w497, "Heave AND Surge.Spare 3"=w496, "Heave AND Surge.Spare 2"=w495, "Heave AND Surge.Spare 1"=w494, "Heave AND Surge.Node Id"=w493, "Heave AND Surge.SPARE 3"=w492, "Heave AND Surge.SPARE 4"=w491, "Heave AND Surge.fwMajor"=w490, "Heave AND Surge.fwMinor"=w489, "Heave AND Surge.Manual Write"=w488, "Heave AND Surge.Heave and Surge Write"=w487) -> (w525:T11)
    }
    frame #13 {
      n462 = control-ref of="Fine Tune Zone"() -> (w542:refnum<vi>)
      n463 = control-ref of="PID Delay (sec)"() -> (w541:refnum<vi>)
      n464 = control-ref of="Max_pos_limit"() -> (w540:refnum<vi>)
      n465 = control-ref of="Min_pos_limit"() -> (w539:refnum<vi>)
      n466 = control-ref of="i_limit"() -> (w538:refnum<vi>)
      n467 = control-ref of="pct_scale"() -> (w529:refnum<vi>)
      n468 = control-ref of="Deadband"() -> (w537:refnum<vi>)
      n469 = control-ref of="Kd"() -> (w536:refnum<vi>)
      n470 = control-ref of="Ki"() -> (w535:refnum<vi>)
      n471 = control-ref of="Kp"() -> (w534:refnum<vi>)
      n472 = control-ref of="Current Position"() -> (w533:refnum<vi>)
      n473 = control-ref of="Set Load"() -> (w532:refnum<vi>)
      n474 = control-ref of="Current Load"() -> (w531:refnum<vi>)
      n475 = control-ref of="Pulse delta"() -> (w530:refnum<vi>)
      n476 = control-ref of="Init Step"() -> (w528:refnum<vi>)
      n477 = control-ref of="Max Step Linit"() -> (w527:refnum<vi>)
      n478 = Bundle By Name(cluster=w544, "New PID LOGIC.Fine Tune Zone"=w542, "New PID LOGIC.PID SDelay"=w541, "New PID LOGIC.Max_pos_limit"=w540, "New PID LOGIC.Min_pos_limit"=w539, "New PID LOGIC.i_limit"=w538, "New PID LOGIC.pct_scale"=w529, "New PID LOGIC.Deadband"=w537, "New PID LOGIC.Kd"=w536, "New PID LOGIC.Ki"=w535, "New PID LOGIC.Kp"=w534, "New PID LOGIC.Current Position"=w533, "New PID LOGIC.Set Load"=w532, "New PID LOGIC.Current Load"=w531, "New PID LOGIC.Pulse delta"=w530, "New PID LOGIC.Init Step"=w528, "New PID LOGIC.Max Step Linit"=w527) -> (w543:T11)
    }
    frame #14 {
      n479 = control-ref of="Manual Write SWAY"() -> (w564:refnum<vi>)
      n480 = control-ref of="Read SWAY Temp"() -> (w545:refnum<vi>)
      n481 = control-ref of="error out Write  SWAY"() -> (w566:refnum<vi>)
      n482 = control-ref of="error out Read SWAY"() -> (w565:refnum<vi>)
      n483 = control-ref of="fwMajor"() -> (w583:refnum<vi>)
      n484 = control-ref of="Homed"() -> (w582:refnum<vi>)
      n485 = control-ref of="Rotary POSE"() -> (w581:refnum<vi>)
      n486 = control-ref of="State"() -> (w580:refnum<vi>)
      n487 = control-ref of="SWAY POSE"() -> (w579:refnum<vi>)
      n488 = control-ref of="Ack ID"() -> (w578:refnum<vi>)
      n489 = control-ref of="faultCode"() -> (w577:refnum<vi>)
      n490 = control-ref of="Node Id"() -> (w576:refnum<vi>)
      n491 = control-ref of="fwMinor"() -> (w575:refnum<vi>)
      n492 = control-ref of="Spare 6"() -> (w574:refnum<vi>)
      n493 = control-ref of="Spare 5"() -> (w573:refnum<vi>)
      n494 = control-ref of="Spare 4"() -> (w572:refnum<vi>)
      n495 = control-ref of="Spare 3"() -> (w571:refnum<vi>)
      n496 = control-ref of="Spare 2"() -> (w570:refnum<vi>)
      n497 = control-ref of="Spare 1"() -> (w569:refnum<vi>)
      n498 = control-ref of="Spare 7"() -> (w568:refnum<vi>)
      n499 = control-ref of="SPARE  5"() -> (w567:refnum<vi>)
      n500 = control-ref of="SPARE  4"() -> (w562:refnum<vi>)
      n501 = control-ref of="SPARE  3"() -> (w561:refnum<vi>)
      n502 = control-ref of="SPARE 2"() -> (w560:refnum<vi>)
      n503 = control-ref of="SPARE 1"() -> (w559:refnum<vi>)
      n504 = control-ref of="Spare 15"() -> (w558:refnum<vi>)
      n505 = control-ref of="Spare 14"() -> (w557:refnum<vi>)
      n506 = control-ref of="Spare 13"() -> (w556:refnum<vi>)
      n507 = control-ref of="Spare 12"() -> (w555:refnum<vi>)
      n508 = control-ref of="Spare 11"() -> (w554:refnum<vi>)
      n509 = control-ref of="Spare 9"() -> (w553:refnum<vi>)
      n510 = control-ref of="Spare 8"() -> (w552:refnum<vi>)
      n511 = control-ref of="SPEED"() -> (w551:refnum<vi>)
      n512 = control-ref of="Distance"() -> (w550:refnum<vi>)
      n513 = control-ref of="Mode Command"() -> (w549:refnum<vi>)
      n514 = control-ref of="Sequence ID"() -> (w548:refnum<vi>)
      n515 = control-ref of="Spare 10"() -> (w546:refnum<vi>)
      n516 = control-ref of="SWAY WRITE"() -> (w563:refnum<vi>)
      n517 = control-ref of="SWAY READ"() -> (w547:refnum<vi>)
      n518 = Bundle By Name(cluster=w585, "SWAY.fwMajor"=w583, "SWAY.Homed"=w582, "SWAY.Rotary POSE"=w581, "SWAY.State"=w580, "SWAY.SWAY POSE"=w579, "SWAY.Ack ID"=w578, "SWAY.faultCode"=w577, "SWAY.Node Id"=w576, "SWAY.fwMinor"=w575, "SWAY.Spare 6"=w574, "SWAY.Spare 5"=w573, "SWAY.Spare 4"=w572, "SWAY.Spare 3"=w571, "SWAY.Spare 2"=w570, "SWAY.Spare 1"=w569, "SWAY.Spare 7"=w568, "SWAY.SPARE  5"=w567, "SWAY.error out Write  SWAY"=w566, "SWAY.error out Read SWAY"=w565, "SWAY.Manual Write SWAY"=w564, "SWAY.SWAY WRITE"=w563, "SWAY.SPARE  4"=w562, "SWAY.SPARE  3"=w561, "SWAY.SPARE 2"=w560, "SWAY.SPARE 1"=w559, "SWAY.Spare 15"=w558, "SWAY.Spare 14"=w557, "SWAY.Spare 13"=w556, "SWAY.Spare 12"=w555, "SWAY.Spare 11"=w554, "SWAY.Spare 9"=w553, "SWAY.Spare 8"=w552, "SWAY.SPEED"=w551, "SWAY.Distance"=w550, "SWAY.Mode Command"=w549, "SWAY.Sequence ID"=w548, "SWAY.SWAY READ"=w547, "SWAY.Spare 10"=w546, "SWAY.Read SWAY Temp"=w545) -> (w584:T11)
    }
  }
  n519 = call <userlib>:"Fit VI window to Largest Dec.vi"() -> ("error out"=w30:errorcluster, "dup VI Ref"=w27:refnum<vi>)  [unwired: 6 in]
  n520 = invoke on="Invoke Node" class="VI" method="FP.Run-Time Position.Maximized"(reference=w27, error in=w30) -> (error out=w29:errorcluster)  [unwired: 2 in, 3 out]
  n521 = call <vilib>:"Clear Errors.vi"("error in (no error)"=w29) -> ("error out"=w28:errorcluster)  [unwired: 5 in, 1 out]
  n522 = control-ref of="This VI"() -> (w33:refnum<vi>)
  n523 = invoke on="Invoke Node" class="VI" method="Default Vals.Reinit All"(reference=w33, error in=w28) -> (reference out=w31:refnum<vi>, error out=w32:errorcluster)  [unwired: 1 in, 1 out]
  n524 = Close Reference(reference=w31, error in (no error)=w32) -> (error out=w26:errorcluster)
  n525 = call "Create User Event - Stop.vi"("error in (no error)"=w26) -> ("error out"=w4:errorcluster, "User Event - Stop"=w13:refnum<user-event>)  [unwired: 9 in]
  n526 = call "main screen queue out Unitest.vi"("error in (no error)"=w4) -> ("error out"=w53:errorcluster, "output Queue"=w25:T12)  [unwired: 9 in]
  n527 = Unbundle By Name(w25) -> ("RAMP MOTOR COM LOOP"=w18:refnum<queue>)
  n528 = Unbundle By Name(w25) -> ("TEMPERATURE COM LOOP"=w20:refnum<queue>)
  n529 = Unbundle By Name(w25) -> ("ECR PORT"=w17:refnum<queue>)
  n530 = Unbundle By Name(w25) -> ("SWAY MOTOR COM LOOP"=w22:refnum<queue>)
  n531 = Unbundle By Name(w25) -> ("UI Loop"=w51:refnum<queue>)
  n532 = Unbundle By Name(w25) -> ("LOAD COM LOOP"=w23:refnum<queue>)
  n533 = Unbundle By Name(w25) -> ("HEAVE MOTOR COM LOOP"=w5:refnum<queue>)
  n534 = Unbundle By Name(w25) -> ("HUMIDITY COM PORT"=w16:refnum<queue>)
  n535 = Unbundle By Name(w25) -> ("PROGRAM LOOP"=w15:refnum<queue>)
  n536 = Unbundle By Name(w25) -> ("MONITOR LOOP"=w12:refnum<queue>)
  n537 = Unbundle By Name(w25) -> ("LOAD PID"=w11:refnum<queue>)
  n538 = Unbundle By Name(w25) -> ("REPORT"=w10:refnum<queue>)
  n539 = register-events(w13) -> (reference out=w45:refnum<event-registration>, error out=w43:errorcluster)  [unwired: 2 in]
  n540 = Merge Errors(w43, w53) -> (w44:errorcluster)
  n541 = while {
    tunnel: w51 -> [w593]
    shift-right: [w591] -> w48
    shift-left: w45 -> [w592]
    tunnel: [w587] -> w46
    stop <- w589 stop-if-true
    # "Event Handling Loop"
    n542 = event shown="[51] \"calculate rotary\": Value Change" {
      selector: w592 -> [_ _ _ _ _ _ _ _ _ _ _ _ _ _ _ _ _ _ _ _ _ _ _ _ _ _ _ _ _ _ _ _ _ _ _ _ _ _ _ _ _ _ _ _ _ _ _ _ _ _ _ _ _ _ _]
      dyn-events: [_ _ _ _ _ _ _ _ _ _ _ _ _ _ _ _ _ _ _ _ _ _ _ _ _ _ _ _ _ _ _ _ _ _ _ _ _ _ _ _ _ _ _ _ _ _ _ _ _ _ _ _ _ _ _] -> w591
      timeout: 10 -> [_ _ _ _ _ _ _ _ _ _ _ _ _ _ _ _ _ _ _ _ _ _ _ _ _ _ _ _ _ _ _ _ _ _ _ _ _ _ _ _ _ _ _ _ _ _ _ _ _ _ _ _ _ _ _]
      tunnel: [_ _ _ _ _ _ _ _ _ _ _ _ _ _ _ _ _ _ _ _ _ _ _ _ _ _ _ _ _ _ _ _ _ _ _ _ _ _ _ _ _ _ _ _ _ _ _ _ _ _ _ _ _ _ TRUE ("Discard?")] -> w589
      tunnel: w593 -> [w598 w602 w607 w612 w617 w622 w627 w632 w637 w642 w647 w652 w657 w662 w667 w672 w677 w682 w687 w692 w697 w702 w707 w712 w717 w722 w727 w732 w737 w742 w747 w752 w757 w762 w767 w772 w777 w782 w787 w792 w797 w802 w807 w812 w817 w822 w827 w832 w837 w842 w847 w852 w855 w860 w862]
      tunnel: [w597 w600 w605 w610 w615 w620 w625 w630 w635 w640 w645 w650 w655 w660 w665 w670 w675 w680 w685 w690 w695 w700 w705 w710 w715 w720 w725 w730 w735 w740 w745 w750 w755 w760 w765 w770 w775 w780 w785 w790 w795 w800 w805 w810 w815 w820 w825 w830 w835 w840 w845 w850 _ w859 _] -> w590
      tunnel: [w596 w601 w606 w611 w616 w621 w626 w631 w636 w641 w646 w651 w656 w661 w666 w671 w676 w681 w686 w691 w696 w701 w706 w711 w716 w721 w726 w731 w736 w741 w746 w751 w756 w761 w766 w771 w776 w781 w786 w791 w796 w801 w806 w811 w816 w821 w826 w831 w836 w841 w846 w851 w855 w858 w862] -> w588
      event Panel Close? {
        n543 = event-data() -> ()  [unwired: 1 in, 1 out]
        n544 = call-poly "Enqueue Message.vi"("Priority Message? (F)"=TRUE, "Message"="Confirm Quit", "Message Queue"=w598) -> ("error out"=w597:errorcluster, "dup Message Queue"=w596:refnum<queue>)  [unwired: 7 in]
        n545 = event-data("Discard?"=TRUE) -> ()  [unwired: 1 in, 1 out]
      }
      event Timeout {
        n546 = event-data() -> ()  [unwired: 1 in, 1 out]
        n547 = call-poly "Enqueue Message.vi"("Priority Message? (F)"=TRUE, "Message"="Time Out", "Message Queue"=w602) -> ("error out"=w600:errorcluster, "dup Message Queue"=w601:refnum<queue>)  [unwired: 7 in]
      }
      event "SAVE  2": Value Change {
        n548 = event-data() -> ()  [unwired: 1 in, 1 out]
        n549 = call-poly "Enqueue Message.vi"("Priority Message? (F)"=TRUE, "Message"="Service Save", "Message Queue"=w607) -> ("error out"=w605:errorcluster, "dup Message Queue"=w606:refnum<queue>)  [unwired: 7 in]
      }
      event "Home": Value Change {
        n550 = event-data() -> ()  [unwired: 1 in, 1 out]
        n551 = call-poly "Enqueue Message.vi"("Priority Message? (F)"=TRUE, "Message"="HOME", "Message Queue"=w612) -> ("error out"=w610:errorcluster, "dup Message Queue"=w611:refnum<queue>)  [unwired: 7 in]
      }
      event "Platform Settings": Value Change {
        n552 = event-data() -> ()  [unwired: 1 in, 1 out]
        n553 = call-poly "Enqueue Message.vi"("Priority Message? (F)"=TRUE, "Message"="Platform Setting", "Message Queue"=w617) -> ("error out"=w615:errorcluster, "dup Message Queue"=w616:refnum<queue>)  [unwired: 7 in]
      }
      event "Configure": Value Change {
        n554 = event-data() -> ()  [unwired: 1 in, 1 out]
        n555 = call-poly "Enqueue Message.vi"("Priority Message? (F)"=TRUE, "Message"="Configure", "Message Queue"=w622) -> ("error out"=w620:errorcluster, "dup Message Queue"=w621:refnum<queue>)  [unwired: 7 in]
      }
      event "Analysis": Value Change {
        n556 = event-data() -> ()  [unwired: 1 in, 1 out]
        n557 = call-poly "Enqueue Message.vi"("Priority Message? (F)"=TRUE, "Message"="Analysis", "Message Queue"=w627) -> ("error out"=w625:errorcluster, "dup Message Queue"=w626:refnum<queue>)  [unwired: 7 in]
      }
      event "service 2": Value Change {
        n558 = event-data() -> ()  [unwired: 1 in, 1 out]
        n559 = call-poly "Enqueue Message.vi"("Priority Message? (F)"=TRUE, "Message"="service 2", "Message Queue"=w632) -> ("error out"=w630:errorcluster, "dup Message Queue"=w631:refnum<queue>)  [unwired: 7 in]
      }
      event "Auto": Value Change {
        n560 = event-data() -> ()  [unwired: 1 in, 1 out]
        n561 = call-poly "Enqueue Message.vi"("Priority Message? (F)"=TRUE, "Message"="Auto", "Message Queue"=w637) -> ("error out"=w635:errorcluster, "dup Message Queue"=w636:refnum<queue>)  [unwired: 7 in]
      }
      event "Select Load Head": Value Change {
        n562 = event-data() -> ()  [unwired: 1 in, 1 out]
        n563 = call-poly "Enqueue Message.vi"("Priority Message? (F)"=TRUE, "Message"="Select Load Head", "Message Queue"=w642) -> ("error out"=w640:errorcluster, "dup Message Queue"=w641:refnum<queue>)  [unwired: 7 in]
      }
      event "com 3": Value Change {
        n564 = event-data() -> ()  [unwired: 1 in, 1 out]
        n565 = call-poly "Enqueue Message.vi"("Priority Message? (F)"=TRUE, "Message"="com 3", "Message Queue"=w647) -> ("error out"=w645:errorcluster, "dup Message Queue"=w646:refnum<queue>)  [unwired: 7 in]
      }
      event "Loading Mode": Value Change {
        n566 = event-data() -> ()  [unwired: 1 in, 1 out]
        n567 = call-poly "Enqueue Message.vi"("Priority Message? (F)"=TRUE, "Message"="Loading Mode", "Message Queue"=w652) -> ("error out"=w650:errorcluster, "dup Message Queue"=w651:refnum<queue>)  [unwired: 7 in]
      }
      event "SSP 0.3": Value Change {
        n568 = event-data() -> ()  [unwired: 1 in, 1 out]
        n569 = call-poly "Enqueue Message.vi"("Priority Message? (F)"=TRUE, "Message"="SSP 0.3", "Message Queue"=w657) -> ("error out"=w655:errorcluster, "dup Message Queue"=w656:refnum<queue>)  [unwired: 7 in]
      }
      event "SSP 0.5": Value Change {
        n570 = event-data() -> ()  [unwired: 1 in, 1 out]
        n571 = call-poly "Enqueue Message.vi"("Priority Message? (F)"=TRUE, "Message"="SSP 0.5", "Message Queue"=w662) -> ("error out"=w660:errorcluster, "dup Message Queue"=w661:refnum<queue>)  [unwired: 7 in]
      }
      event "SSP 0.75": Value Change {
        n572 = event-data() -> ()  [unwired: 1 in, 1 out]
        n573 = call-poly "Enqueue Message.vi"("Priority Message? (F)"=TRUE, "Message"="SSP 0.75", "Message Queue"=w667) -> ("error out"=w665:errorcluster, "dup Message Queue"=w666:refnum<queue>)  [unwired: 7 in]
      }
      event "LHBack": Value Change {
        n574 = event-data() -> ()  [unwired: 1 in, 1 out]
        n575 = call-poly "Enqueue Message.vi"("Priority Message? (F)"=TRUE, "Message"="LHBack", "Message Queue"=w672) -> ("error out"=w670:errorcluster, "dup Message Queue"=w671:refnum<queue>)  [unwired: 7 in]
      }
      event "LHNext": Value Change {
        n576 = event-data() -> ()  [unwired: 1 in, 1 out]
        n577 = call-poly "Enqueue Message.vi"("Priority Message? (F)"=TRUE, "Message"="LHNext", "Message Queue"=w677) -> ("error out"=w675:errorcluster, "dup Message Queue"=w676:refnum<queue>)  [unwired: 7 in]
      }
      event "Rot Ver": Value Change {
        n578 = event-data() -> ()  [unwired: 1 in, 1 out]
        n579 = call-poly "Enqueue Message.vi"("Priority Message? (F)"=TRUE, "Message"="Rot Ver", "Message Queue"=w682) -> ("error out"=w680:errorcluster, "dup Message Queue"=w681:refnum<queue>)  [unwired: 7 in]
      }
      event "Scratch": Value Change {
        n580 = event-data() -> ()  [unwired: 1 in, 1 out]
        n581 = call-poly "Enqueue Message.vi"("Priority Message? (F)"=TRUE, "Message"="Scratch", "Message Queue"=w687) -> ("error out"=w685:errorcluster, "dup Message Queue"=w686:refnum<queue>)  [unwired: 7 in]
      }
      event "Motion Mode:": Value Change {
        n582 = event-data() -> ()  [unwired: 1 in, 1 out]
        n583 = call-poly "Enqueue Message.vi"("Priority Message? (F)"=TRUE, "Message"="Motion Mode:", "Message Queue"=w692) -> ("error out"=w690:errorcluster, "dup Message Queue"=w691:refnum<queue>)  [unwired: 7 in]
      }
      event "MMBack": Value Change {
        n584 = event-data() -> ()  [unwired: 1 in, 1 out]
        n585 = call-poly "Enqueue Message.vi"("Priority Message? (F)"=TRUE, "Message"="MMBack", "Message Queue"=w697) -> ("error out"=w695:errorcluster, "dup Message Queue"=w696:refnum<queue>)  [unwired: 7 in]
      }
      event "MMNext": Value Change {
        n586 = event-data() -> ()  [unwired: 1 in, 1 out]
        n587 = call-poly "Enqueue Message.vi"("Priority Message? (F)"=TRUE, "Message"="MMNext", "Message Queue"=w702) -> ("error out"=w700:errorcluster, "dup Message Queue"=w701:refnum<queue>)  [unwired: 7 in]
      }
      event "APBack": Value Change {
        n588 = event-data() -> ()  [unwired: 1 in, 1 out]
        n589 = call-poly "Enqueue Message.vi"("Priority Message? (F)"=TRUE, "Message"="APBack", "Message Queue"=w707) -> ("error out"=w705:errorcluster, "dup Message Queue"=w706:refnum<queue>)  [unwired: 7 in]
      }
      event "SNext": Value Change {
        n590 = event-data() -> ()  [unwired: 1 in, 1 out]
        n591 = call-poly "Enqueue Message.vi"("Priority Message? (F)"=TRUE, "Message"="SNext", "Message Queue"=w712) -> ("error out"=w710:errorcluster, "dup Message Queue"=w711:refnum<queue>)  [unwired: 7 in]
      }
      event "ZeroAll": Value Change {
        n592 = event-data() -> ()  [unwired: 1 in, 1 out]
        n593 = call-poly "Enqueue Message.vi"("Priority Message? (F)"=TRUE, "Message"="ZeroAll", "Message Queue"=w717) -> ("error out"=w715:errorcluster, "dup Message Queue"=w716:refnum<queue>)  [unwired: 7 in]
      }
      event "Enable Platform": Value Change {
        n594 = event-data() -> ()  [unwired: 1 in, 1 out]
        n595 = call-poly "Enqueue Message.vi"("Priority Message? (F)"=TRUE, "Message"="Enable Platform", "Message Queue"=w722) -> ("error out"=w720:errorcluster, "dup Message Queue"=w721:refnum<queue>)  [unwired: 7 in]
      }
      event "Heave Up main": Value Change {
        n596 = event-data() -> ()  [unwired: 1 in, 1 out]
        n597 = call-poly "Enqueue Message.vi"("Priority Message? (F)"=TRUE, "Message"="Heave Up main", "Message Queue"=w727) -> ("error out"=w725:errorcluster, "dup Message Queue"=w726:refnum<queue>)  [unwired: 7 in]
      }
      event "Heave Up MM": Value Change {
        n598 = event-data() -> ()  [unwired: 1 in, 1 out]
        n599 = call-poly "Enqueue Message.vi"("Priority Message? (F)"=TRUE, "Message"="Heave Up MM", "Message Queue"=w732) -> ("error out"=w730:errorcluster, "dup Message Queue"=w731:refnum<queue>)  [unwired: 7 in]
      }
      event "Heave Down Main": Value Change {
        n600 = event-data() -> ()  [unwired: 1 in, 1 out]
        n601 = call-poly "Enqueue Message.vi"("Priority Message? (F)"=TRUE, "Message"="Heave Down Main", "Message Queue"=w737) -> ("error out"=w735:errorcluster, "dup Message Queue"=w736:refnum<queue>)  [unwired: 7 in]
      }
      event "Heave Down MM": Value Change {
        n602 = event-data() -> ()  [unwired: 1 in, 1 out]
        n603 = call-poly "Enqueue Message.vi"("Priority Message? (F)"=TRUE, "Message"="Heave Down MM", "Message Queue"=w742) -> ("error out"=w740:errorcluster, "dup Message Queue"=w741:refnum<queue>)  [unwired: 7 in]
      }
      event "Manual Write Heave & Surge": Value Change {
        n604 = event-data() -> ()  [unwired: 1 in, 1 out]
        n605 = call-poly "Enqueue Message.vi"("Priority Message? (F)"=TRUE, "Message"="Manual Write Heave & Surge", "Message Queue"=w747) -> ("error out"=w745:errorcluster, "dup Message Queue"=w746:refnum<queue>)  [unwired: 7 in]
      }
      event "Manual Write SWAY": Value Change {
        n606 = event-data() -> ()  [unwired: 1 in, 1 out]
        n607 = call-poly "Enqueue Message.vi"("Priority Message? (F)"=TRUE, "Message"="Manual Write SWAY", "Message Queue"=w752) -> ("error out"=w750:errorcluster, "dup Message Queue"=w751:refnum<queue>)  [unwired: 7 in]
      }
      event "Surge Backward Main": Value Change {
        n608 = event-data() -> ()  [unwired: 1 in, 1 out]
        n609 = call-poly "Enqueue Message.vi"("Priority Message? (F)"=TRUE, "Message"="Surge Backward Main", "Message Queue"=w757) -> ("error out"=w755:errorcluster, "dup Message Queue"=w756:refnum<queue>)  [unwired: 7 in]
      }
      event "Surge Backward MM": Value Change {
        n610 = event-data() -> ()  [unwired: 1 in, 1 out]
        n611 = call-poly "Enqueue Message.vi"("Priority Message? (F)"=TRUE, "Message"="Surge Backward MM", "Message Queue"=w762) -> ("error out"=w760:errorcluster, "dup Message Queue"=w761:refnum<queue>)  [unwired: 7 in]
      }
      event "Surge Forward Main": Value Change {
        n612 = event-data() -> ()  [unwired: 1 in, 1 out]
        n613 = call-poly "Enqueue Message.vi"("Priority Message? (F)"=TRUE, "Message"="Surge Forward Main", "Message Queue"=w767) -> ("error out"=w765:errorcluster, "dup Message Queue"=w766:refnum<queue>)  [unwired: 7 in]
      }
      event "Surge Forward MM": Value Change {
        n614 = event-data() -> ()  [unwired: 1 in, 1 out]
        n615 = call-poly "Enqueue Message.vi"("Priority Message? (F)"=TRUE, "Message"="Surge Forward MM", "Message Queue"=w772) -> ("error out"=w770:errorcluster, "dup Message Queue"=w771:refnum<queue>)  [unwired: 7 in]
      }
      event "Sway Left Main": Value Change {
        n616 = event-data() -> ()  [unwired: 1 in, 1 out]
        n617 = call-poly "Enqueue Message.vi"("Priority Message? (F)"=TRUE, "Message"="Sway Left Main", "Message Queue"=w777) -> ("error out"=w775:errorcluster, "dup Message Queue"=w776:refnum<queue>)  [unwired: 7 in]
      }
      event "Sway Left MM": Value Change {
        n618 = event-data() -> ()  [unwired: 1 in, 1 out]
        n619 = call-poly "Enqueue Message.vi"("Priority Message? (F)"=TRUE, "Message"="Sway Left MM", "Message Queue"=w782) -> ("error out"=w780:errorcluster, "dup Message Queue"=w781:refnum<queue>)  [unwired: 7 in]
      }
      event "Sway Right MM": Value Change {
        n620 = event-data() -> ()  [unwired: 1 in, 1 out]
        n621 = call-poly "Enqueue Message.vi"("Priority Message? (F)"=TRUE, "Message"="Sway Right MM", "Message Queue"=w787) -> ("error out"=w785:errorcluster, "dup Message Queue"=w786:refnum<queue>)  [unwired: 7 in]
      }
      event "Sway Right Main": Value Change {
        n622 = event-data() -> ()  [unwired: 1 in, 1 out]
        n623 = call-poly "Enqueue Message.vi"("Priority Message? (F)"=TRUE, "Message"="Sway Right Main", "Message Queue"=w792) -> ("error out"=w790:errorcluster, "dup Message Queue"=w791:refnum<queue>)  [unwired: 7 in]
      }
      event "Load En": Value Change {
        n624 = event-data() -> ()  [unwired: 1 in, 1 out]
        n625 = call-poly "Enqueue Message.vi"("Priority Message? (F)"=TRUE, "Message"="Load En", "Message Queue"=w797) -> ("error out"=w795:errorcluster, "dup Message Queue"=w796:refnum<queue>)  [unwired: 7 in]
      }
      event "apply load": Value Change {
        n626 = event-data() -> ()  [unwired: 1 in, 1 out]
        n627 = call-poly "Enqueue Message.vi"("Priority Message? (F)"=TRUE, "Message"="apply load", "Message Queue"=w802) -> ("error out"=w800:errorcluster, "dup Message Queue"=w801:refnum<queue>)  [unwired: 7 in]
      }
      event "BACK": Value Change {
        n628 = event-data() -> ()  [unwired: 1 in, 1 out]
        n629 = call-poly "Enqueue Message.vi"("Priority Message? (F)"=TRUE, "Message"="BACK", "Message Queue"=w807) -> ("error out"=w805:errorcluster, "dup Message Queue"=w806:refnum<queue>)  [unwired: 7 in]
      }
      event "Start Test": Value Change {
        n630 = event-data() -> ()  [unwired: 1 in, 1 out]
        n631 = call-poly "Enqueue Message.vi"("Priority Message? (F)"=TRUE, "Message"="Start Test", "Message Queue"=w812) -> ("error out"=w810:errorcluster, "dup Message Queue"=w811:refnum<queue>)  [unwired: 7 in]
      }
      event "STOP": Value Change {
        n632 = event-data() -> ()  [unwired: 1 in, 1 out]
        n633 = call-poly "Enqueue Message.vi"("Priority Message? (F)"=TRUE, "Message"="STOP", "Message Queue"=w817) -> ("error out"=w815:errorcluster, "dup Message Queue"=w816:refnum<queue>)  [unwired: 7 in]
      }
      event "PlaceModule": Value Change {
        n634 = event-data() -> ()  [unwired: 1 in, 1 out]
        n635 = call-poly "Enqueue Message.vi"("Priority Message? (F)"=TRUE, "Message"="PlaceModule", "Message Queue"=w822) -> ("error out"=w820:errorcluster, "dup Message Queue"=w821:refnum<queue>)  [unwired: 7 in]
      }
      event "HomeRot", "HomeScratch", "HomeScratch": Value Change {
        n636 = event-data() -> ()  [unwired: 1 in, 1 out]
        n637 = call-poly "Enqueue Message.vi"("Priority Message? (F)"=TRUE, "Message"="Stage Homing", "Message Queue"=w827) -> ("error out"=w825:errorcluster, "dup Message Queue"=w826:refnum<queue>)  [unwired: 7 in]
      }
      event "Clear 3": Value Change {
        n638 = event-data() -> ()  [unwired: 1 in, 1 out]
        n639 = call-poly "Enqueue Message.vi"("Priority Message? (F)"=TRUE, "Message"="Clear 3", "Message Queue"=w832) -> ("error out"=w830:errorcluster, "dup Message Queue"=w831:refnum<queue>)  [unwired: 7 in]
      }
      event "Set WTD": Value Change {
        n640 = event-data() -> ()  [unwired: 1 in, 1 out]
        n641 = call-poly "Enqueue Message.vi"("Priority Message? (F)"=TRUE, "Message"="Set WTD", "Message Queue"=w837) -> ("error out"=w835:errorcluster, "dup Message Queue"=w836:refnum<queue>)  [unwired: 7 in]
      }
      event "Import 2": Value Change {
        n642 = event-data() -> ()  [unwired: 1 in, 1 out]
        n643 = call-poly "Enqueue Message.vi"("Priority Message? (F)"=TRUE, "Message"="Import 2", "Message Queue"=w842) -> ("error out"=w840:errorcluster, "dup Message Queue"=w841:refnum<queue>)  [unwired: 7 in]
      }
      event "Save 2": Value Change {
        n644 = event-data() -> ()  [unwired: 1 in, 1 out]
        n645 = call-poly "Enqueue Message.vi"("Priority Message? (F)"=TRUE, "Message"="Save 2", "Message Queue"=w847) -> ("error out"=w845:errorcluster, "dup Message Queue"=w846:refnum<queue>)  [unwired: 7 in]
      }
      event "calculate rotary": Value Change {
        n646 = event-data() -> ()  [unwired: 1 in, 1 out]
        n647 = call-poly "Enqueue Message.vi"("Priority Message? (F)"=TRUE, "Message"="Calculate Rotary", "Message Queue"=w852) -> ("error out"=w850:errorcluster, "dup Message Queue"=w851:refnum<queue>)  [unwired: 7 in]
      }
      event Application Instance Close {
        # "#CodeRecommended - When a project closes, all VIs within that project are aborted and leave memory. However, any code placed in this event frame is guaranteed to run to completion, so add any cleanup code that absolutely must happen here."
        n648 = event-data() -> ()  [unwired: 1 in, 1 out]
      }
      event "EXIT": Value Change {
        n649 = event-data() -> ()  [unwired: 1 in, 1 out]
        n650 = call-poly "Enqueue Message.vi"("Priority Message? (F)"=TRUE, "Message"="Exit", "Message Queue"=w860) -> ("error out"=w859:errorcluster, "dup Message Queue"=w858:refnum<queue>)  [unwired: 7 in]
      }
      event User Event {
        # "The Message Handling Loop processed an \"Exit\" message, which fired this event to stop the Event Handling Loop."
        n651 = event-data() -> ()  [unwired: 1 in, 1 out]
      }
    }
    n652 = call "LAB-IQ Error Handler - Event Handling Loop.vi"("error in (no error)"=w590, "Message Queue"=w588) -> ("dup error in"=w587:errorcluster)  [unwired: 8 in, 1 out]
  }
  n653 = while {
    tunnel: w51 -> [w866]
    shift-right: [w873] -> _
    shift-left: w14 -> [w874]
    tunnel: w13 -> [w871]
    tunnel: w44 -> [w870]
    tunnel: [w864] -> w52
    stop <- w872 stop-if-true
    # "Message Handling Loop"
    n654 = call "Dequeue Message.vi"("error in (no error)"=w870, "Message Queue"=w866) -> ("error out"=w869:errorcluster, "Message Data"=w867:variant, "Message"=w868:string, "dup Message Queue"=w865:refnum<queue>)  [unwired: 6 in]
    n655 = case "Message Cases" shown="\"Calculate Rotary\"" w868 {
      selector: w868 -> [_ _ _ _ _ _ _ _ _ _ _ _ _ _ _ _ _ _ _ _ _ _ _ _ _ _ _ _ _ _ _ _ _ _ _ _ _ _ _ _ _ _ _ _ _ _ _ _ _ _ _ _ _ _ _ _ w1790]
      tunnel: w865 -> [_ w927 _ _ _ _ _ _ _ _ _ _ _ _ _ _ _ _ _ _ _ _ _ _ _ _ _ _ _ _ _ _ _ _ _ _ _ _ _ _ _ _ _ _ _ _ _ _ _ _ _ _ _ _ w1778 w1789 _]
      tunnel: w869 -> [w877 w929 w931 w935 w956 w973 w990 w1007 w1028 w1040 w1045 w1049 w1056 w1061 w1126 w1152 w1178 w1213 w1229 w1281 w1285 w1288 w1295 w1338 w1350 w1379 w1409 w1428 w1439 w1450 w1461 w1472 w1483 w1494 w1505 w1517 w1528 w1539 w1550 w1559 w1570 w1581 w1611 w1652 w1658 w1674 w1678 w1681 w1689 w1701 w1713 w1733 w1745 w1774 w1781 w1782 _]
      tunnel: [w884 w896 w931 w936 w951 w968 w985 w1002 w1023 w1032 w1043 w1047 w1054 w1065 w1122 w1148 w1174 w1214 w1230 w1245 w1284 w1287 w1294 w1337 w1349 w1378 w1396 w1430 w1441 w1452 w1463 w1474 w1485 w1496 w1507 w1518 w1529 w1540 w1551 w1561 w1571 w1580 w1610 w1631 w1657 w1675 w1677 w1680 w1688 w1700 w1708 w1726 w1745 w1768 w1780 w1785 w1791] -> w863
      tunnel: w874 -> [w876 w887 w932 w934 w942 w959 w976 w993 w1011 w1030 w1042 w1046 w1052 w1060 w1124 w1150 w1176 w1201 w1216 w1232 w1283 w1286 w1289 w1332 w1348 w1361 w1391 w1426 w1437 w1448 w1459 w1470 w1481 w1492 w1503 w1515 w1526 w1537 w1548 w1558 w1569 w1579 w1609 w1630 w1656 w1660 w1676 w1679 w1683 w1695 w1706 w1728 w1749 w1773 w1775 w1788 w1792]
      tunnel: [w876 w887 w932 w934 w942 w959 w976 w993 w1011 w1030 w1042 w1046 w1052 w1060 w1124 w1150 w1176 w1201 w1216 w1232 w1283 w1286 w1289 w1332 w1348 w1361 w1391 w1426 w1437 w1448 w1459 w1470 w1481 w1492 w1503 w1515 w1526 w1537 w1548 w1558 w1569 w1579 w1609 w1630 w1656 w1660 w1676 w1679 w1683 w1695 w1706 w1728 w1749 w1773 w1775 w1788 w1792] -> w873
      tunnel: [_ _ _ _ _ _ _ _ _ _ _ _ _ _ _ _ _ _ _ _ _ _ _ _ _ _ _ _ _ _ _ _ _ _ _ _ _ _ _ _ _ _ _ _ _ _ _ _ _ _ _ _ _ _ _ TRUE _] -> w872
      tunnel: w867 -> [_ _ _ _ _ _ _ _ _ _ _ _ _ _ _ _ _ _ _ _ _ _ _ _ _ _ _ _ _ _ _ _ _ _ _ _ _ _ _ _ _ _ _ _ _ _ _ _ _ _ _ _ _ w1772 _ _ _]
      tunnel: w871 -> [_ _ _ _ _ _ _ _ _ _ _ _ _ _ _ _ _ _ _ _ _ _ _ _ _ _ _ _ _ _ _ _ _ _ _ _ _ _ _ _ _ _ _ _ _ _ _ _ _ _ _ _ _ _ _ w1784 _]
      frame "Time Out" {
        n656 = call "File Name Entereed Check.vi"("error in (no error)"=w877, "Data Cluster"=w876) -> ("error out"=w881:errorcluster)  [unwired: 9 in]
        n657 = call "Load Cell and Susppension Selection Parameter.vi"("error in (no error)"=w877, "Data Cluster"=w876) -> ("error out"=w880:errorcluster)  [unwired: 9 in]
        n658 = call "Load Cell Higher Value in Steps.vi"("error in (no error)"=w877, "main ref"=w876) -> ("error out"=w879:errorcluster)  [unwired: 9 in]
        n659 = call "To Check whether module selected.vi"("error in (no error)"=w877, "main ref"=w876) -> ("error out"=w878:errorcluster)  [unwired: 9 in]
        n660 = call "Rotatry Speed Limit Ristriction.vi"("error in (no error)"=w877, "main ref"=w876) -> ("error out"=w875:errorcluster)  [unwired: 9 in]
        n661 = call "Pulse_mm conversion loop.vi"("error in (no error)"=w877, "main ref"=w876) -> ("error out"=w885:errorcluster)  [unwired: 9 in]
        n662 = call "Load Commiunication Error.vi"("error in (no error)"=w877, "main ref"=w876) -> ("error out"=w882:errorcluster)  [unwired: 9 in]
        n663 = call "Stage Homing Error Display Status.vi"("error in (no error)"=w877, "Data Cluster"=w876) -> ("error out"=w883:errorcluster)  [unwired: 9 in]
        n664 = Merge Errors(w885, w882, w883, w881, w880, w879, w878, w875) -> (w884:errorcluster)
      }
      frame "init" {
        # "Initialize - All initialization work should take place in this message, since other loops can potentially enqueue messages that execute immediately after this one."
        n665 = call-poly "Enqueue Message.vi"("error in (no error)"=w929, "Message"="Init Other Loop", "Message Queue"=w927) -> ("error out"=w930:errorcluster)  [unwired: 7 in, 1 out]
        n666 = Unbundle By Name(w887) -> ("Loading.Communication is established"=w902:refnum<vi>)
        n667 = Unbundle By Name(w887) -> ("Loading Com Port.Load Cell Temp"=w921:refnum<vi>)
        n668 = Unbundle By Name(w887) -> ("Loading.SSP 0.3"=w915:refnum<vi>)
        n669 = Unbundle By Name(w887) -> ("Loading.SSP 0.5"=w912:refnum<vi>)
        n670 = Unbundle By Name(w887) -> ("Loading.SSP 0.75"=w907:refnum<vi>)
        n671 = Unbundle By Name(w887) -> ("Motion Module.Set WTD"=w895:refnum<vi>)
        n672 = call "Read Config Unitest.vi"("error in (no error)"=w930, "main ref"=w887) -> ("error out"=w925:errorcluster)  [unwired: 9 in]
        n673 = Unbundle By Name(w887) -> ("PID.Ramp"=w899:refnum<vi>)
        n674 = call "Encrypt file path creation.vi"("error in (no error)"=w925) -> ("error out"=w924:errorcluster, "File Path"=w923:path)  [unwired: 9 in]
        n675 = property class="Bool (strict)"(reference=w921, "Value"=FALSE) -> (reference out=w919:refnum<vi>, error out=w920:errorcluster)  [unwired: 1 in]
        n676 = property class="Bool (strict)"(reference=w912, "Visible"=FALSE) -> (reference out=w910:refnum<vi>, error out=w911:errorcluster)  [unwired: 1 in]
        n677 = property class="Bool (strict)"(reference=w915, "Visible"=FALSE) -> (reference out=w917:refnum<vi>, error out=w916:errorcluster)  [unwired: 1 in]
        n678 = property class="Bool (strict)"(reference=w907, "Visible"=FALSE) -> (reference out=w909:refnum<vi>, error out=w908:errorcluster)  [unwired: 1 in]
        n679 = property class="Bool (strict)"(reference=w899, "Value"=FALSE) -> (reference out=w901:refnum<vi>, error out=w900:errorcluster)  [unwired: 1 in]
        n680 = property class="Bool (strict)"(reference=w895, "Visible"=FALSE, "DisabledEnum"=T13."Disabled and Grayed Out" ("Disabled")) -> (reference out=w892:refnum<vi>, error out=w894:errorcluster)  [unwired: 1 in]
        n681 = property class="Bool (strict)"(reference=w902, "Visible"=FALSE ("Value")) -> (reference out=w904:refnum<vi>, error out=w903:errorcluster)  [unwired: 1 in]
        n682 = call "DATA ENCRYPT STRING FILE WRITE.vi"("file path (dialog if empty)"=w923, "error in (no error)"=w924, "User Action"="System Booted", "main ref"=w887) -> ("error out"=w926:errorcluster)  [unwired: 5 in, 1 out]
        n683 = Close Reference(reference=w910, error in (no error)=w911) -> ()  [unwired: 1 out]
        n684 = Close Reference(reference=w917, error in (no error)=w916) -> ()  [unwired: 1 out]
        n685 = Close Reference(reference=w909, error in (no error)=w908) -> ()  [unwired: 1 out]
        n686 = Close Reference(reference=w901, error in (no error)=w900) -> ()  [unwired: 1 out]
        n687 = Close Reference(reference=w919, error in (no error)=w920) -> ()  [unwired: 1 out]
        n688 = Close Reference(reference=w892, error in (no error)=w894) -> ()  [unwired: 1 out]
        n689 = Unbundle By Name(w887) -> ("Motion Module.Wear Track Diameter"=w889:refnum<vi>)
        n690 = Close Reference(reference=w904, error in (no error)=w903) -> ()  [unwired: 1 out]
        n691 = call "Reinitial Parameter After Test.vi"("error in (no error)"=w926, "main ref"=w887) -> ("error out"=w896:errorcluster)  [unwired: 9 in]
        n692 = local write "HEAVE ENABLE"(FALSE ("HEAVE ENABLE")) -> ()
        n693 = property class="DigNum (strict)"(reference=w889, "Value"=0.0) -> (reference out=w888:refnum<vi>, error out=w890:errorcluster)  [unwired: 1 in]
        n694 = Close Reference(reference=w888, error in (no error)=w890) -> ()  [unwired: 1 out]
      }
      frame "Init Other Loop" {
      }
      frame "Service Save" {
        n695 = call "Write Config Unitest.vi"("error in (no error)"=w935, "main ref"=w934) -> ("error out"=w940:errorcluster)  [unwired: 9 in]
        n696 = call "Stall Data Flow.vim"("value in"=w940, "milliseconds to wait"=u32 2000) -> ("value out"=w939:errorcluster)  [unwired: 1 out]
        n697 = call "Read Config Unitest.vi"("error in (no error)"=w939, "main ref"=w934) -> ("error out"=w937:errorcluster)  [unwired: 9 in]
        n698 = call "DATA ENCRYPT STRING FILE WRITE.vi"("error in (no error)"=w937, "User Action"="Service Parameter Saved", "main ref"=w934) -> ("error out"=w936:errorcluster)  [unwired: 6 in, 1 out]
      }
      frame "HOME" {
        n699 = call "DATA ENCRYPT STRING FILE WRITE.vi"("error in (no error)"=w956, "User Action"="User Pressed Home", "main ref"=w942) -> ("error out"=w952:errorcluster)  [unwired: 6 in, 1 out]
        n700 = Unbundle By Name(w942) -> ("Main Home Screen.MainPage"=w947:refnum<vi>)
        n701 = Unbundle By Name(w942) -> ("Main Home Screen.Home"=w955:refnum<vi>)
        n702 = Unbundle By Name(w942) -> ("Main Home Screen.GUI"=w945:refnum<vi>)
        n703 = property class="Bool (strict)"(reference=w955, error in=w952, "Value"=FALSE) -> (reference out=w953:refnum<vi>, error out=w954:errorcluster)
        n704 = property class="TabCtl (strict)"(reference=w947, "Value"=T5."HOME") -> (reference out=w949:refnum<vi>, error out=w948:errorcluster)  [unwired: 1 in]
        n705 = property class="TabCtl (strict)"(reference=w945, "Value"=T4."Setup") -> (reference out=w943:refnum<vi>, error out=w944:errorcluster)  [unwired: 1 in]
        n706 = Close Reference(reference=w953, error in (no error)=w954) -> (error out=w951:errorcluster)
        n707 = Close Reference(reference=w949, error in (no error)=w948) -> ()  [unwired: 1 out]
        n708 = Close Reference(reference=w943, error in (no error)=w944) -> ()  [unwired: 1 out]
      }
      frame "Platform Setting" {
        n709 = call "DATA ENCRYPT STRING FILE WRITE.vi"("error in (no error)"=w973, "User Action"="User Pressed Platform Setting", "main ref"=w959) -> ("error out"=w969:errorcluster)  [unwired: 6 in, 1 out]
        n710 = Unbundle By Name(w959) -> ("Main Home Screen.Platform Settings"=w972:refnum<vi>)
        n711 = Unbundle By Name(w959) -> ("Main Home Screen.MainPage"=w964:refnum<vi>)
        n712 = Unbundle By Name(w959) -> ("Main Home Screen.GUI"=w962:refnum<vi>)
        n713 = property class="TabCtl (strict)"(reference=w964, "Value"=T5."PlatformSetting") -> (reference out=w966:refnum<vi>, error out=w965:errorcluster)  [unwired: 1 in]
        n714 = property class="TabCtl (strict)"(reference=w962, "Value"=T4."Setup") -> (reference out=w960:refnum<vi>, error out=w961:errorcluster)  [unwired: 1 in]
        n715 = property class="Bool (strict)"(reference=w972, error in=w969, "Value"=FALSE) -> (reference out=w970:refnum<vi>, error out=w971:errorcluster)
        n716 = Close Reference(reference=w966, error in (no error)=w965) -> ()  [unwired: 1 out]
        n717 = Close Reference(reference=w960, error in (no error)=w961) -> ()  [unwired: 1 out]
        n718 = Close Reference(reference=w970, error in (no error)=w971) -> (error out=w968:errorcluster)
      }
      frame "Configure" {
        n719 = call "DATA ENCRYPT STRING FILE WRITE.vi"("error in (no error)"=w990, "User Action"="User Pressed Configure", "main ref"=w976) -> ("error out"=w986:errorcluster)  [unwired: 6 in, 1 out]
        n720 = Unbundle By Name(w976) -> ("Main Home Screen.Configure"=w989:refnum<vi>)
        n721 = Unbundle By Name(w976) -> ("Main Home Screen.MainPage"=w981:refnum<vi>)
        n722 = Unbundle By Name(w976) -> ("Main Home Screen.GUI"=w979:refnum<vi>)
        n723 = property class="Bool (strict)"(reference=w989, error in=w986, "Value"=FALSE) -> (reference out=w987:refnum<vi>, error out=w988:errorcluster)
        n724 = property class="TabCtl (strict)"(reference=w981, "Value"=T5."Details") -> (reference out=w983:refnum<vi>, error out=w982:errorcluster)  [unwired: 1 in]
        n725 = property class="TabCtl (strict)"(reference=w979, "Value"=T4."Setup") -> (reference out=w977:refnum<vi>, error out=w978:errorcluster)  [unwired: 1 in]
        n726 = Close Reference(reference=w987, error in (no error)=w988) -> (error out=w985:errorcluster)
        n727 = Close Reference(reference=w983, error in (no error)=w982) -> ()  [unwired: 1 out]
        n728 = Close Reference(reference=w977, error in (no error)=w978) -> ()  [unwired: 1 out]
      }
      frame "Analysis" {
        n729 = call "DATA ENCRYPT STRING FILE WRITE.vi"("error in (no error)"=w1007, "User Action"="User Pressed Analysis", "main ref"=w993) -> ("error out"=w1003:errorcluster)  [unwired: 6 in, 1 out]
        n730 = Unbundle By Name(w993) -> ("Main Home Screen.MainPage"=w998:refnum<vi>)
        n731 = Unbundle By Name(w993) -> ("Main Home Screen.Analysis"=w1006:refnum<vi>)
        n732 = Unbundle By Name(w993) -> ("Main Home Screen.GUI"=w996:refnum<vi>)
        n733 = property class="Bool (strict)"(reference=w1006, error in=w1003, "Value"=FALSE) -> (reference out=w1004:refnum<vi>, error out=w1005:errorcluster)
        n734 = property class="TabCtl (strict)"(reference=w998, "Value"=T5."Analysis") -> (reference out=w1000:refnum<vi>, error out=w999:errorcluster)  [unwired: 1 in]
        n735 = property class="TabCtl (strict)"(reference=w996, "Value"=T4."Setup") -> (reference out=w994:refnum<vi>, error out=w995:errorcluster)  [unwired: 1 in]
        n736 = Close Reference(reference=w1004, error in (no error)=w1005) -> (error out=w1002:errorcluster)
        n737 = Close Reference(reference=w1000, error in (no error)=w999) -> ()  [unwired: 1 out]
        n738 = Close Reference(reference=w994, error in (no error)=w995) -> ()  [unwired: 1 out]
      }
      frame "service 2" {
        n739 = call "DATA ENCRYPT STRING FILE WRITE.vi"("error in (no error)"=w1028, "User Action"="User Pressed service", "main ref"=w1011) -> ("error out"=w1024:errorcluster)  [unwired: 6 in, 1 out]
        n740 = Unbundle By Name(w1011) -> ("Main Screen.Main Screen Tab"=w1012:refnum<vi>)
        n741 = Unbundle By Name(w1011) -> ("Main Home Screen.MainPage"=w1019:refnum<vi>)
        n742 = Unbundle By Name(w1011) -> ("Main Home Screen.Analysis"=w1027:refnum<vi>)
        n743 = Unbundle By Name(w1011) -> ("Main Home Screen.GUI"=w1017:refnum<vi>)
        n744 = property class="Bool (strict)"(reference=w1027, error in=w1024, "Value"=FALSE) -> (reference out=w1025:refnum<vi>, error out=w1026:errorcluster)
        n745 = property class="TabCtl (strict)"(reference=w1019, "Value"=T5."HOME") -> (reference out=w1021:refnum<vi>, error out=w1020:errorcluster)  [unwired: 1 in]
        n746 = property class="TabCtl (strict)"(reference=w1017, "Value"=T4."Begin") -> (reference out=w1015:refnum<vi>, error out=w1016:errorcluster)  [unwired: 1 in]
        n747 = property class="TabCtl (strict)"(reference=w1012, "Value"=T8."About") -> (reference out=w1009:refnum<vi>, error out=w1013:errorcluster)  [unwired: 1 in]
        n748 = Close Reference(reference=w1025, error in (no error)=w1026) -> (error out=w1023:errorcluster)
        n749 = Close Reference(reference=w1021, error in (no error)=w1020) -> ()  [unwired: 1 out]
        n750 = Close Reference(reference=w1015, error in (no error)=w1016) -> ()  [unwired: 1 out]
        n751 = Close Reference(reference=w1009, error in (no error)=w1013) -> ()  [unwired: 1 out]
      }
      frame "Auto" {
        n752 = call "DATA ENCRYPT STRING FILE WRITE.vi"("error in (no error)"=w1040, "User Action"="User Pressed Auto File Name", "main ref"=w1030) -> ("error out"=w1037:errorcluster)  [unwired: 6 in, 1 out]
        n753 = Get Date/Time In Seconds() -> (seconds since 1Jan1904=w1038:timestamp)
        n754 = Format Into String(format string="%<%I_%M_%S_%p_%d_%B_%Y>T", error in=w1037, w1038) -> (resulting string=w1031:string, error out=w1033:errorcluster)  [unwired: 1 in]
        n755 = Unbundle By Name(w1030) -> ("Config Screen.FILE"=w1036:refnum<vi>)
        n756 = property class="Str"(reference=w1036, error in=w1033, "Value"=w1031) -> (reference out=w1034:refnum<vi>, error out=w1035:errorcluster)
        n757 = Close Reference(reference=w1034, error in (no error)=w1035) -> (error out=w1032:errorcluster)
      }
      frame "Select Load Head" {
        n758 = call "Reinitial Parameter.vi"("error in (no error)"=w1045, "Data Cluster"=w1042) -> ("error out"=w1044:errorcluster)  [unwired: 9 in]
        n759 = call "FILE NAME RECHECK.vi"("error in (no error)"=w1044, "main ref"=w1042) -> ("error out"=w1043:errorcluster)  [unwired: 9 in]
      }
      frame "com 3" {
        n760 = call "DATA ENCRYPT STRING FILE WRITE.vi"("error in (no error)"=w1049, "User Action"="User Pressed Check Load Communication", "main ref"=w1046) -> ("error out"=w1048:errorcluster)  [unwired: 6 in, 1 out]
        n761 = call "SET LOAD PARAMETERS.vi"("error in (no error)"=w1048, "main ref"=w1046) -> ("error out"=w1047:errorcluster)  [unwired: 9 in]
      }
      frame "ZeroAll" {
        n762 = call "DATA ENCRYPT STRING FILE WRITE.vi"("error in (no error)"=w1056, "User Action"="User Pressed Zero All", "main ref"=w1052) -> ("error out"=w1055:errorcluster)  [unwired: 6 in, 1 out]
        n763 = local write "ZeroAll"(FALSE ("ZeroAll")) -> ()
        n764 = call "LOAD CELL FGV MAIN.vi"("Enum"=T14."ZEROALL", "error in (no error)"=w1055, "main ref"=w1052) -> ("error IO"=w1054:errorcluster)  [unwired: 8 in]
      }
      frame "Loading Mode" {
        n765 = Unbundle By Name(w1060) -> ("Loading.Loading Mode"=w1062:refnum<vi>)
        n766 = property class="Ring (strict)"(reference=w1062, error in=w1061) -> (reference out=w1064:refnum<vi>, error out=w1063:errorcluster, "Value"=w1058:u16)
        n767 = Close Reference(reference=w1064, error in (no error)=w1063) -> (error out=w1059:errorcluster)
        n768 = case shown="1" w1058 {
          tunnel: [w1079 w1096 w1108 w1120] -> w1065
          tunnel: w1060 -> [w1066 w1082 w1100 w1112]
          tunnel: w1059 -> [w1080 w1095 w1107 w1119]
          frame 0, Default {
            n769 = Unbundle By Name(w1066) -> ("Loading.Enter the Loading Rate (N/min)"=w1073:refnum<vi>)
            n770 = Unbundle By Name(w1066) -> ("Loading.Load Selection"=w1076:refnum<vi>)
            n771 = Unbundle By Name(w1066) -> ("Loading.Enter the Final Load (N)"=w1068:refnum<vi>)
            n772 = property class="TabCtl (strict)"(reference=w1076, "Value"=T6."Constant") -> (reference out=w1078:refnum<vi>, error out=w1077:errorcluster)  [unwired: 1 in]
            n773 = property class="DigNum (strict)"(reference=w1073, "DisabledEnum"=T13."Disabled and Grayed Out" ("Disabled")) -> (reference out=w1072:refnum<vi>, error out=w1074:errorcluster)  [unwired: 1 in]
            n774 = property class="DigNum (strict)"(reference=w1068, "DisabledEnum"=T13."Disabled and Grayed Out" ("Disabled")) -> (reference out=w1069:refnum<vi>, error out=w1067:errorcluster)  [unwired: 1 in]
            n775 = call "DATA ENCRYPT STRING FILE WRITE.vi"("error in (no error)"=w1080, "User Action"="User selected Constant Mode", "main ref"=w1066) -> ("error out"=w1079:errorcluster)  [unwired: 6 in, 1 out]
            n776 = Close Reference(reference=w1078, error in (no error)=w1077) -> ()  [unwired: 1 out]
            n777 = Close Reference(reference=w1072, error in (no error)=w1074) -> ()  [unwired: 1 out]
            n778 = Close Reference(reference=w1069, error in (no error)=w1067) -> ()  [unwired: 1 out]
          }
          frame 1 {
            n779 = Unbundle By Name(w1082) -> ("Loading.Enter the Loading Rate (N/min)"=w1093:refnum<vi>)
            n780 = Unbundle By Name(w1082) -> ("Loading.Enter the Final Load (N)"=w1088:refnum<vi>)
            n781 = Unbundle By Name(w1082) -> ("Loading.Load Selection"=w1084:refnum<vi>)
            n782 = property class="TabCtl (strict)"(reference=w1084, "Value"=T6."Constant") -> (reference out=w1086:refnum<vi>, error out=w1085:errorcluster)  [unwired: 1 in]
            n783 = property class="DigNum (strict)"(reference=w1093, "DisabledEnum"=T13."Enabled" ("Disabled")) -> (reference out=w1092:refnum<vi>, error out=w1094:errorcluster)  [unwired: 1 in]
            n784 = property class="DigNum (strict)"(reference=w1088, "DisabledEnum"=T13."Enabled" ("Disabled")) -> (reference out=w1089:refnum<vi>, error out=w1087:errorcluster)  [unwired: 1 in]
            n785 = call "DATA ENCRYPT STRING FILE WRITE.vi"("error in (no error)"=w1095, "User Action"="User selected Ramp Mode", "main ref"=w1082) -> ("error out"=w1096:errorcluster)  [unwired: 6 in, 1 out]
            n786 = Close Reference(reference=w1086, error in (no error)=w1085) -> ()  [unwired: 1 out]
            n787 = Close Reference(reference=w1092, error in (no error)=w1094) -> ()  [unwired: 1 out]
            n788 = Close Reference(reference=w1089, error in (no error)=w1087) -> ()  [unwired: 1 out]
          }
          frame 2 {
            n789 = Unbundle By Name(w1100) -> ("Loading.Load Selection"=w1104:refnum<vi>)
            n790 = Unbundle By Name(w1100) -> ("Loading.Warning 2"=w1102:refnum<vi>)
            n791 = property class="TabCtl (strict)"(reference=w1104, "Value"=T6."Step") -> (reference out=w1106:refnum<vi>, error out=w1105:errorcluster)  [unwired: 1 in]
            n792 = property class="Bool (strict)"(reference=w1102, "Visible"=FALSE) -> (reference out=w1098:refnum<vi>, error out=w1101:errorcluster)  [unwired: 1 in]
            n793 = call "DATA ENCRYPT STRING FILE WRITE.vi"("error in (no error)"=w1107, "User Action"="User selected Step Mode", "main ref"=w1100) -> ("error out"=w1108:errorcluster)  [unwired: 6 in, 1 out]
            n794 = Close Reference(reference=w1106, error in (no error)=w1105) -> ()  [unwired: 1 out]
            n795 = Close Reference(reference=w1098, error in (no error)=w1101) -> ()  [unwired: 1 out]
          }
          frame 3 {
            n796 = Unbundle By Name(w1112) -> ("Loading.Load Selection"=w1116:refnum<vi>)
            n797 = Unbundle By Name(w1112) -> ("Loading.Warning 2"=w1114:refnum<vi>)
            n798 = property class="TabCtl (strict)"(reference=w1116, "Value"=T6."Indentation") -> (reference out=w1118:refnum<vi>, error out=w1117:errorcluster)  [unwired: 1 in]
            n799 = property class="Bool (strict)"(reference=w1114, "Visible"=FALSE) -> (reference out=w1110:refnum<vi>, error out=w1113:errorcluster)  [unwired: 1 in]
            n800 = call "DATA ENCRYPT STRING FILE WRITE.vi"("error in (no error)"=w1119, "User Action"="User selected Indentation Mode", "main ref"=w1112) -> ("error out"=w1120:errorcluster)  [unwired: 6 in, 1 out]
            n801 = Close Reference(reference=w1118, error in (no error)=w1117) -> ()  [unwired: 1 out]
            n802 = Close Reference(reference=w1110, error in (no error)=w1113) -> ()  [unwired: 1 out]
          }
        }
      }
      frame "SSP 0.3" {
        n803 = Unbundle By Name(w1124) -> ("Loading.SSP 0.3"=w1127:refnum<vi>)
        n804 = property class="Bool (strict)"(reference=w1127, error in=w1126) -> (reference out=w1129:refnum<vi>, error out=w1128:errorcluster, "Value"=w1125:bool)
        n805 = Close Reference(reference=w1129, error in (no error)=w1128) -> (error out=w1123:errorcluster)
        n806 = case shown="True" w1125 {
          tunnel: w1124 -> [_ w1131]
          tunnel: w1123 -> [w1130 w1139]
          tunnel: [w1130 w1138] -> w1122
          frame False {
          }
          frame True {
            w1141 = FALSE ("Value")
            n807 = Unbundle By Name(w1131) -> ("Loading.Enter the Load  (N)"=w1137:refnum<vi>)
            n808 = Unbundle By Name(w1131) -> ("Loading.SSP 0.75"=w1142:refnum<vi>)
            n809 = Unbundle By Name(w1131) -> ("Loading.SSP 0.5"=w1147:refnum<vi>)
            n810 = property class="Bool (strict)"(reference=w1142, "Value"=w1141) -> (reference out=w1144:refnum<vi>, error out=w1143:errorcluster)  [unwired: 1 in]
            n811 = property class="Bool (strict)"(reference=w1147, "Value"=w1141) -> (reference out=w1145:refnum<vi>, error out=w1146:errorcluster)  [unwired: 1 in]
            n812 = property class="DigNum (strict)"(reference=w1137, "Minimum"=2.0 ("Data Entry Limits:Minimum"), "Maximum"=50.0 ("Data Entry Limits:Maximum"), "Increment"=0.1 ("Data Entry Limits:Increment")) -> (reference out=w1135:refnum<vi>, error out=w1136:errorcluster)  [unwired: 1 in]
            n813 = call "DATA ENCRYPT STRING FILE WRITE.vi"("error in (no error)"=w1139, "User Action"="User selected 0.3 SSP", "main ref"=w1131) -> ("error out"=w1138:errorcluster)  [unwired: 6 in, 1 out]
            n814 = Close Reference(reference=w1144, error in (no error)=w1143) -> ()  [unwired: 1 out]
            n815 = Close Reference(reference=w1145, error in (no error)=w1146) -> ()  [unwired: 1 out]
            n816 = Close Reference(reference=w1135, error in (no error)=w1136) -> ()  [unwired: 1 out]
          }
        }
      }
      frame "SSP 0.5" {
        n817 = Unbundle By Name(w1150) -> ("Loading.SSP 0.5"=w1153:refnum<vi>)
        n818 = property class="Bool (strict)"(reference=w1153, error in=w1152) -> (reference out=w1155:refnum<vi>, error out=w1154:errorcluster, "Value"=w1151:bool)
        n819 = Close Reference(reference=w1155, error in (no error)=w1154) -> (error out=w1149:errorcluster)
        n820 = case shown="True" w1151 {
          tunnel: w1150 -> [_ w1157]
          tunnel: w1149 -> [w1156 w1165]
          tunnel: [w1156 w1164] -> w1148
          frame False {
          }
          frame True {
            w1167 = FALSE ("Value")
            n821 = Unbundle By Name(w1157) -> ("Loading.Enter the Load  (N)"=w1163:refnum<vi>)
            n822 = Unbundle By Name(w1157) -> ("Loading.SSP 0.75"=w1173:refnum<vi>)
            n823 = Unbundle By Name(w1157) -> ("Loading.SSP 0.3"=w1168:refnum<vi>)
            n824 = property class="Bool (strict)"(reference=w1168, "Value"=w1167) -> (reference out=w1170:refnum<vi>, error out=w1169:errorcluster)  [unwired: 1 in]
            n825 = property class="Bool (strict)"(reference=w1173, "Value"=w1167) -> (reference out=w1171:refnum<vi>, error out=w1172:errorcluster)  [unwired: 1 in]
            n826 = property class="DigNum (strict)"(reference=w1163, "Minimum"=2.0 ("Data Entry Limits:Minimum"), "Maximum"=200.0 ("Data Entry Limits:Maximum"), "Increment"=0.1 ("Data Entry Limits:Increment")) -> (reference out=w1161:refnum<vi>, error out=w1162:errorcluster)  [unwired: 1 in]
            n827 = call "DATA ENCRYPT STRING FILE WRITE.vi"("error in (no error)"=w1165, "User Action"="User selected 0.5 SSP", "main ref"=w1157) -> ("error out"=w1164:errorcluster)  [unwired: 6 in, 1 out]
            n828 = Close Reference(reference=w1170, error in (no error)=w1169) -> ()  [unwired: 1 out]
            n829 = Close Reference(reference=w1171, error in (no error)=w1172) -> ()  [unwired: 1 out]
            n830 = Close Reference(reference=w1161, error in (no error)=w1162) -> ()  [unwired: 1 out]
          }
        }
      }
      frame "SSP 0.75" {
        n831 = Unbundle By Name(w1176) -> ("Loading.SSP 0.75"=w1179:refnum<vi>)
        n832 = property class="Bool (strict)"(reference=w1179, error in=w1178) -> (reference out=w1181:refnum<vi>, error out=w1180:errorcluster, "Value"=w1177:bool)
        n833 = Close Reference(reference=w1181, error in (no error)=w1180) -> (error out=w1175:errorcluster)
        n834 = case shown="True" w1177 {
          tunnel: w1176 -> [_ w1183]
          tunnel: w1175 -> [w1182 w1191]
          tunnel: [w1182 w1190] -> w1174
          frame False {
          }
          frame True {
            w1193 = FALSE ("Value")
            n835 = Unbundle By Name(w1183) -> ("Loading.SSP 0.3"=w1194:refnum<vi>)
            n836 = Unbundle By Name(w1183) -> ("Loading.SSP 0.5"=w1199:refnum<vi>)
            n837 = Unbundle By Name(w1183) -> ("Loading.Enter the Load  (N)"=w1189:refnum<vi>)
            n838 = property class="Bool (strict)"(reference=w1194, "Value"=w1193) -> (reference out=w1196:refnum<vi>, error out=w1195:errorcluster)  [unwired: 1 in]
            n839 = property class="Bool (strict)"(reference=w1199, "Value"=w1193) -> (reference out=w1197:refnum<vi>, error out=w1198:errorcluster)  [unwired: 1 in]
            n840 = property class="DigNum (strict)"(reference=w1189, "Minimum"=200.0 ("Data Entry Limits:Minimum"), "Maximum"=500.0 ("Data Entry Limits:Maximum"), "Increment"=0.1 ("Data Entry Limits:Increment")) -> (reference out=w1187:refnum<vi>, error out=w1188:errorcluster)  [unwired: 1 in]
            n841 = call "DATA ENCRYPT STRING FILE WRITE.vi"("error in (no error)"=w1191, "User Action"="User selected 0.75 SSP", "main ref"=w1183) -> ("error out"=w1190:errorcluster)  [unwired: 6 in, 1 out]
            n842 = Close Reference(reference=w1196, error in (no error)=w1195) -> ()  [unwired: 1 out]
            n843 = Close Reference(reference=w1197, error in (no error)=w1198) -> ()  [unwired: 1 out]
            n844 = Close Reference(reference=w1187, error in (no error)=w1188) -> ()  [unwired: 1 out]
          }
        }
      }
      frame "LHBack" {
        # "Back to Configure"
        n845 = Unbundle By Name(w1201) -> ("Main Home Screen.GUI"=w1210:refnum<vi>)
        n846 = Unbundle By Name(w1201) -> ("Main Home Screen.MainPage"=w1206:refnum<vi>)
        n847 = Unbundle By Name(w1201) -> ("Loading.LHBack"=w1204:refnum<vi>)
        n848 = property class="TabCtl (strict)"(reference=w1206, "Value"=T5."HOME") -> (reference out=w1208:refnum<vi>, error out=w1207:errorcluster)  [unwired: 1 in]
        n849 = property class="Bool (strict)"(reference=w1204, "Value"=FALSE) -> (reference out=w1202:refnum<vi>, error out=w1203:errorcluster)  [unwired: 1 in]
        n850 = property class="TabCtl (strict)"(reference=w1210, "Value"=T4."Setup") -> (reference out=w1212:refnum<vi>, error out=w1211:errorcluster)  [unwired: 1 in]
        n851 = Close Reference(reference=w1208, error in (no error)=w1207) -> ()  [unwired: 1 out]
        n852 = Close Reference(reference=w1202, error in (no error)=w1203) -> ()  [unwired: 1 out]
        n853 = Close Reference(reference=w1212, error in (no error)=w1211) -> ()  [unwired: 1 out]
        n854 = call "DATA ENCRYPT STRING FILE WRITE.vi"("error in (no error)"=w1213, "User Action"="User selected Back to Configure", "main ref"=w1201) -> ("error out"=w1214:errorcluster)  [unwired: 6 in, 1 out]
      }
      frame "MMBack" {
        # "Back to Configure"
        n855 = Unbundle By Name(w1216) -> ("Motion Module.MMBack"=w1220:refnum<vi>)
        n856 = Unbundle By Name(w1216) -> ("Main Home Screen.GUI"=w1226:refnum<vi>)
        n857 = Unbundle By Name(w1216) -> ("Main Home Screen.MainPage"=w1222:refnum<vi>)
        n858 = property class="Bool (strict)"(reference=w1220, "Value"=FALSE) -> (reference out=w1218:refnum<vi>, error out=w1219:errorcluster)  [unwired: 1 in]
        n859 = property class="TabCtl (strict)"(reference=w1222, "Value"=T5."HOME") -> (reference out=w1224:refnum<vi>, error out=w1223:errorcluster)  [unwired: 1 in]
        n860 = property class="TabCtl (strict)"(reference=w1226, "Value"=T4."Load Head") -> (reference out=w1228:refnum<vi>, error out=w1227:errorcluster)  [unwired: 1 in]
        n861 = Close Reference(reference=w1218, error in (no error)=w1219) -> ()  [unwired: 1 out]
        n862 = Close Reference(reference=w1224, error in (no error)=w1223) -> ()  [unwired: 1 out]
        n863 = Close Reference(reference=w1228, error in (no error)=w1227) -> ()  [unwired: 1 out]
        n864 = call "DATA ENCRYPT STRING FILE WRITE.vi"("error in (no error)"=w1229, "User Action"="User selected Back to Load Selection", "main ref"=w1216) -> ("error out"=w1230:errorcluster)  [unwired: 6 in, 1 out]
      }
      frame "LHNext" {
        w1266 = FALSE ("Visible")
        n865 = Unbundle By Name(w1232) -> ("Motion Module.HomeRot"=w1272:refnum<vi>)
        n866 = Unbundle By Name(w1232) -> ("Motion Module.HomeScratch"=w1267:refnum<vi>)
        n867 = Unbundle By Name(w1232) -> ("Motion Module.PlaceModule"=w1265:refnum<vi>)
        n868 = Unbundle By Name(w1232) -> ("Motion Module.Motion Mode:"=w1258:refnum<vi>)
        n869 = Unbundle By Name(w1232) -> ("Motion Module.Motion Direction:  3"=w1257:refnum<vi>)
        n870 = Unbundle By Name(w1232) -> ("Motion Module.Wear Track Diameter (mm)"=w1251:refnum<vi>)
        n871 = Unbundle By Name(w1232) -> ("Motion Module.Set WTD"=w1248:refnum<vi>)
        n872 = Unbundle By Name(w1232) -> ("Motion Module.Rotary Module Selection"=w1242:refnum<vi>)
        n873 = call "DATA ENCRYPT STRING FILE WRITE.vi"("error in (no error)"=w1281, "User Action"="User selected Select Module", "main ref"=w1232) -> ("error out"=w1245:errorcluster)  [unwired: 6 in, 1 out]
        n874 = property class="TabCtl (strict)"(reference=w1242, "Visible"=FALSE) -> (reference out=w1241:refnum<vi>, error out=w1243:errorcluster)  [unwired: 1 in]
        n875 = property class="Bool (strict)"(reference=w1272, error in=w1245, "Visible"=w1266) -> (reference out=w1270:refnum<vi>, error out=w1271:errorcluster)
        n876 = property class="Bool (strict)"(reference=w1267, error in=w1245, "Visible"=w1266) -> (reference out=w1269:refnum<vi>, error out=w1268:errorcluster)
        n877 = property class="Bool (strict)"(reference=w1265, error in=w1245, "Visible"=TRUE) -> (reference out=w1263:refnum<vi>, error out=w1264:errorcluster)
        n878 = property class="Ring (strict)"(reference=w1258, error in=w1245, "Visible"=FALSE) -> (reference out=w1260:refnum<vi>, error out=w1259:errorcluster)
        n879 = property class="Ring (strict)"(reference=w1257, error in=w1245, "Visible"=FALSE) -> (reference out=w1254:refnum<vi>, error out=w1256:errorcluster)
        n880 = property class="DigNum (strict)"(reference=w1251, "Visible"=FALSE) -> (reference out=w1250:refnum<vi>, error out=w1252:errorcluster)  [unwired: 1 in]
        n881 = property class="Bool (strict)"(reference=w1248, "Visible"=FALSE) -> (reference out=w1249:refnum<vi>, error out=w1247:errorcluster)  [unwired: 1 in]
        n882 = Close Reference(reference=w1270, error in (no error)=w1271) -> ()  [unwired: 1 out]
        n883 = Close Reference(reference=w1269, error in (no error)=w1268) -> ()  [unwired: 1 out]
        n884 = Close Reference(reference=w1263, error in (no error)=w1264) -> ()  [unwired: 1 out]
        n885 = Close Reference(reference=w1260, error in (no error)=w1259) -> ()  [unwired: 1 out]
        n886 = Close Reference(reference=w1254, error in (no error)=w1256) -> ()  [unwired: 1 out]
        n887 = Close Reference(reference=w1250, error in (no error)=w1252) -> ()  [unwired: 1 out]
        n888 = Close Reference(reference=w1241, error in (no error)=w1243) -> ()  [unwired: 1 out]
        n889 = Close Reference(reference=w1249, error in (no error)=w1247) -> ()  [unwired: 1 out]
        n890 = Unbundle By Name(w1232) -> ("Motion Module.M3 Image"=w1240:refnum<vi>)
        n891 = Unbundle By Name(w1232) -> ("Main Home Screen.GUI"=w1278:refnum<vi>)
        n892 = Unbundle By Name(w1232) -> ("Main Home Screen.MainPage"=w1274:refnum<vi>)
        n893 = Unbundle By Name(w1232) -> ("Loading.LHNext"=w1236:refnum<vi>)
        n894 = property class="TabCtl (strict)"(reference=w1240, "Value"=enum32{"Page 1", "Page 2"}."Page 2") -> (reference out=w1238:refnum<vi>, error out=w1239:errorcluster)  [unwired: 1 in]
        n895 = property class="TabCtl (strict)"(reference=w1274, "Value"=T5."HOME") -> (reference out=w1276:refnum<vi>, error out=w1275:errorcluster)  [unwired: 1 in]
        n896 = property class="TabCtl (strict)"(reference=w1278, "Value"=T4."Motion Module") -> (reference out=w1280:refnum<vi>, error out=w1279:errorcluster)  [unwired: 1 in]
        n897 = property class="Bool (strict)"(reference=w1236, "Value"=FALSE ("Visible")) -> (reference out=w1233:refnum<vi>, error out=w1235:errorcluster)  [unwired: 1 in]
        n898 = Close Reference(reference=w1238, error in (no error)=w1239) -> ()  [unwired: 1 out]
        n899 = Close Reference(reference=w1233, error in (no error)=w1235) -> ()  [unwired: 1 out]
        n900 = Close Reference(reference=w1276, error in (no error)=w1275) -> ()  [unwired: 1 out]
        n901 = Close Reference(reference=w1280, error in (no error)=w1279) -> ()  [unwired: 1 out]
      }
      frame "Rot Ver" {
        n902 = call "Rotory Module Selection.vi"("error in (no error)"=w1285, "Data Cluster"=w1283) -> ("error out"=w1284:errorcluster)  [unwired: 9 in]
      }
      frame "Scratch" {
        n903 = call "Scratch Module Selection.vi"("error in (no error)"=w1288, "Data Cluster"=w1286) -> ("error out"=w1287:errorcluster)  [unwired: 9 in]
      }
      frame "Motion Mode:" {
        n904 = Unbundle By Name(w1289) -> ("Motion Module.Motion Mode:"=w1291:refnum<vi>)
        n905 = property class="Ring (strict)"(reference=w1291) -> (reference out=w1293:refnum<vi>, error out=w1292:errorcluster, "Value"=w1290:u16)  [unwired: 1 in]
        n906 = Close Reference(reference=w1293, error in (no error)=w1292) -> ()  [unwired: 1 out]
        n907 = case shown="3" w1290 {
          tunnel: w1295 -> [w1304 w1313 w1322 w1331]
          tunnel: [w1303 w1312 w1321 w1330] -> w1294
          tunnel: w1289 -> [w1302 w1311 w1320 w1329]
          tunnel: w1289 -> [w1297 w1306 w1315 w1324]
          frame 0, Default {
            n908 = Unbundle By Name(w1297) -> ("Motion Module.Rotary Module Selection"=w1298:refnum<vi>)
            n909 = property class="TabCtl (strict)"(reference=w1298, "Value"=T7."Uniform Rotation") -> (reference out=w1300:refnum<vi>, error out=w1299:errorcluster)  [unwired: 1 in]
            n910 = Close Reference(reference=w1300, error in (no error)=w1299) -> ()  [unwired: 1 out]
            n911 = call "DATA ENCRYPT STRING FILE WRITE.vi"("error in (no error)"=w1304, "User Action"="User Selected Uniform Rotation", "main ref"=w1302) -> ("error out"=w1303:errorcluster)  [unwired: 6 in, 1 out]
          }
          frame 1 {
            n912 = Unbundle By Name(w1306) -> ("Motion Module.Rotary Module Selection"=w1307:refnum<vi>)
            n913 = property class="TabCtl (strict)"(reference=w1307, "Value"=T7."Angular Oscillation") -> (reference out=w1309:refnum<vi>, error out=w1308:errorcluster)  [unwired: 1 in]
            n914 = Close Reference(reference=w1309, error in (no error)=w1308) -> ()  [unwired: 1 out]
            n915 = call "DATA ENCRYPT STRING FILE WRITE.vi"("error in (no error)"=w1313, "User Action"="User Selected Angular Oscillation", "main ref"=w1311) -> ("error out"=w1312:errorcluster)  [unwired: 6 in, 1 out]
          }
          frame 2 {
            n916 = Unbundle By Name(w1315) -> ("Motion Module.Rotary Module Selection"=w1316:refnum<vi>)
            n917 = property class="TabCtl (strict)"(reference=w1316, "Value"=T7."Speed Ramp") -> (reference out=w1318:refnum<vi>, error out=w1317:errorcluster)  [unwired: 1 in]
            n918 = Close Reference(reference=w1318, error in (no error)=w1317) -> ()  [unwired: 1 out]
            n919 = call "DATA ENCRYPT STRING FILE WRITE.vi"("error in (no error)"=w1322, "User Action"="User Selected Ramp Mode", "main ref"=w1320) -> ("error out"=w1321:errorcluster)  [unwired: 6 in, 1 out]
          }
          frame 3 {
            n920 = Unbundle By Name(w1324) -> ("Motion Module.Rotary Module Selection"=w1325:refnum<vi>)
            n921 = property class="TabCtl (strict)"(reference=w1325, "Value"=T7."Speed Step") -> (reference out=w1327:refnum<vi>, error out=w1326:errorcluster)  [unwired: 1 in]
            n922 = Close Reference(reference=w1327, error in (no error)=w1326) -> ()  [unwired: 1 out]
            n923 = call "DATA ENCRYPT STRING FILE WRITE.vi"("error in (no error)"=w1331, "User Action"="User Selected Step Mode", "main ref"=w1329) -> ("error out"=w1330:errorcluster)  [unwired: 6 in, 1 out]
          }
        }
      }
      frame "MMNext" {
        n924 = Unbundle By Name(w1332) -> ("Motion Module.MMNext"=w1336:refnum<vi>)
        n925 = Unbundle By Name(w1332) -> ("Motion Module.MMNext"=w1343:refnum<vi>)
        n926 = Unbundle By Name(w1332) -> ("Main Home Screen.GUI"=w1345:refnum<vi>)
        n927 = property class="Bool (strict)"(reference=w1336, "Value"=FALSE ("Visible")) -> (reference out=w1333:refnum<vi>, error out=w1335:errorcluster)  [unwired: 1 in]
        n928 = property class="TabCtl (strict)"(reference=w1345, "Value"=T4."Environment") -> (reference out=w1347:refnum<vi>, error out=w1346:errorcluster)  [unwired: 1 in]
        n929 = property class="Bool (strict)"(reference=w1343, "Value"=FALSE) -> (reference out=w1341:refnum<vi>, error out=w1342:errorcluster)  [unwired: 1 in]
        n930 = Close Reference(reference=w1333, error in (no error)=w1335) -> ()  [unwired: 1 out]
        n931 = Close Reference(reference=w1341, error in (no error)=w1342) -> ()  [unwired: 1 out]
        n932 = Close Reference(reference=w1347, error in (no error)=w1346) -> ()  [unwired: 1 out]
        n933 = call "DATA ENCRYPT STRING FILE WRITE.vi"("error in (no error)"=w1338, "User Action"="User Selected SetUp Module", "main ref"=w1332) -> ("error out"=w1337:errorcluster)  [unwired: 6 in, 1 out]
      }
      frame "APBack" {
        n934 = Unbundle By Name(w1348) -> ("Environmental control.APBack"=w1355:refnum<vi>)
        n935 = Unbundle By Name(w1348) -> ("Main Home Screen.GUI"=w1357:refnum<vi>)
        n936 = property class="TabCtl (strict)"(reference=w1357, "Value"=T4."Motion Module") -> (reference out=w1359:refnum<vi>, error out=w1358:errorcluster)  [unwired: 1 in]
        n937 = property class="Bool (strict)"(reference=w1355, "Value"=FALSE) -> (reference out=w1353:refnum<vi>, error out=w1354:errorcluster)  [unwired: 1 in]
        n938 = Close Reference(reference=w1353, error in (no error)=w1354) -> ()  [unwired: 1 out]
        n939 = Close Reference(reference=w1359, error in (no error)=w1358) -> ()  [unwired: 1 out]
        n940 = call "DATA ENCRYPT STRING FILE WRITE.vi"("error in (no error)"=w1350, "User Action"="User Selected Back to Module", "main ref"=w1348) -> ("error out"=w1349:errorcluster)  [unwired: 6 in, 1 out]
      }
      frame "SNext" {
        w1372 = FALSE ("Value")
        n941 = Unbundle By Name(w1361) -> ("Main Screen.zNL 2"=w1364:refnum<vi>)
        n942 = Unbundle By Name(w1361) -> ("Main Screen.Start Test"=w1375:refnum<vi>)
        n943 = Unbundle By Name(w1361) -> ("Main Screen.STOP"=w1374:refnum<vi>)
        n944 = Unbundle By Name(w1361) -> ("Environmental control.SNext"=w1384:refnum<vi>)
        n945 = Unbundle By Name(w1361) -> ("Main Home Screen.GUI"=w1386:refnum<vi>)
        n946 = Unbundle By Name(w1361) -> ("PID.Ramp"=w1367:refnum<vi>)
        n947 = property class="Bool (strict)"(reference=w1364, "DisabledEnum"=T13."Enabled" ("Disabled")) -> (reference out=w1362:refnum<vi>, error out=w1363:errorcluster)  [unwired: 1 in]
        n948 = property class="Bool (strict)"(reference=w1367, "Value"=FALSE) -> (reference out=w1365:refnum<vi>, error out=w1368:errorcluster)  [unwired: 1 in]
        n949 = property class="Bool (strict)"(reference=w1375, "Visible"=TRUE ("Value"), "Value"=FALSE) -> (reference out=w1370:refnum<vi>, error out=w1376:errorcluster)  [unwired: 1 in]
        n950 = property class="Bool (strict)"(reference=w1374, "Value"=w1372, "Visible"=w1372) -> (reference out=w1369:refnum<vi>, error out=w1373:errorcluster)  [unwired: 1 in]
        n951 = property class="TabCtl (strict)"(reference=w1386, "Value"=T4."Begin") -> (reference out=w1388:refnum<vi>, error out=w1387:errorcluster)  [unwired: 1 in]
        n952 = property class="Bool (strict)"(reference=w1384, "Value"=FALSE) -> (reference out=w1382:refnum<vi>, error out=w1383:errorcluster)  [unwired: 1 in]
        n953 = Close Reference(reference=w1362, error in (no error)=w1363) -> ()  [unwired: 1 out]
        n954 = Close Reference(reference=w1365, error in (no error)=w1368) -> ()  [unwired: 1 out]
        n955 = Close Reference(reference=w1370, error in (no error)=w1376) -> ()  [unwired: 1 out]
        n956 = Close Reference(reference=w1369, error in (no error)=w1373) -> ()  [unwired: 1 out]
        n957 = Close Reference(reference=w1382, error in (no error)=w1383) -> ()  [unwired: 1 out]
        n958 = Close Reference(reference=w1388, error in (no error)=w1387) -> ()  [unwired: 1 out]
        n959 = call "DATA ENCRYPT STRING FILE WRITE.vi"("error in (no error)"=w1379, "User Action"="User Pressed Setup", "main ref"=w1361) -> ("error out"=w1378:errorcluster)  [unwired: 6 in, 1 out]
      }
      frame "Enable Platform" {
        n960 = Unbundle By Name(w1391) -> ("Heave AND Surge.Sequence ID"=w1393:refnum<vi>)
        n961 = Unbundle By Name(w1391) -> ("Heave AND Surge.Mode Command"=w1417:refnum<vi>)
        n962 = Unbundle By Name(w1391) -> ("Heave AND Surge.Distance"=w1414:refnum<vi>)
        n963 = Unbundle By Name(w1391) -> ("Heave AND Surge.SPEED"=w1411:refnum<vi>)
        n964 = Unbundle By Name(w1391) -> ("Platform Settings.Enable Platform"=w1425:refnum<vi>)
        n965 = property class="DigNum (strict)"(reference=w1393, "Value"=u16 0) -> (reference out=w1392:refnum<vi>, error out=w1394:errorcluster)  [unwired: 1 in]
        n966 = property class="DigNum (strict)"(reference=w1414, error in=w1409, "Value"=sgl 0.0) -> (reference out=w1415:refnum<vi>, error out=w1413:errorcluster)
        n967 = property class="DigNum (strict)"(reference=w1411, error in=w1409, "Value"=sgl 0.0) -> (reference out=w1412:refnum<vi>, error out=w1410:errorcluster)
        n968 = property class="DigNum (strict)"(reference=w1417, error in=w1409, "Value"=u8 1) -> (reference out=w1416:refnum<vi>, error out=w1418:errorcluster)
        n969 = property class="Bool (strict)"(reference=w1425, "Value"=FALSE) -> (reference out=w1423:refnum<vi>, error out=w1424:errorcluster)  [unwired: 1 in]
        n970 = Close Reference(reference=w1392, error in (no error)=w1394) -> (error out=w1390:errorcluster)
        n971 = Close Reference(reference=w1415, error in (no error)=w1413) -> (error out=w1406:errorcluster)
        n972 = Close Reference(reference=w1412, error in (no error)=w1410) -> (error out=w1405:errorcluster)
        n973 = Close Reference(reference=w1416, error in (no error)=w1418) -> (error out=w1407:errorcluster)
        n974 = Close Reference(reference=w1423, error in (no error)=w1424) -> ()  [unwired: 1 out]
        n975 = Merge Errors(w1409, w1407, w1406, w1405, w1390) -> (w1408:errorcluster)
        n976 = call "DATA ENCRYPT STRING FILE WRITE.vi"("error in (no error)"=w1408, "User Action"="User Pressed Enable Platform", "main ref"=w1391) -> ("error out"=w1420:errorcluster)  [unwired: 6 in, 1 out]
        n977 = call "HEAVE WRITE FGV.vi"("Enum - Menu"=Heave_Write_enum."WRITE", "error in (no error)"=w1420, "main ref"=w1391) -> ("error out"=w1397:errorcluster)  [unwired: 8 in]
        n978 = Unbundle By Name(w1391) -> ("Heave AND Surge.Read Heave Temp"=w1401:refnum<vi>)
        n979 = property class="Bool (strict)"(reference=w1401, error in=w1397, "Value"=TRUE) -> (reference out=w1399:refnum<vi>, error out=w1400:errorcluster)
        n980 = Close Reference(reference=w1399, error in (no error)=w1400) -> (error out=w1396:errorcluster)
        "HEAVE ENABLE" <- TRUE ("HEAVE ENABLE")
      }
      frame "Heave Up main" {
        n981 = Unbundle By Name(w1426) -> ("Platform Settings.Heave Up main"=w1436:refnum<vi>)
        n982 = call "Heave Up Main.vi"("error in (no error)"=w1428, "main ref"=w1426) -> ("error out"=w1427:errorcluster)  [unwired: 9 in]
        n983 = property class="Bool (strict)"(reference=w1436, "Value"=FALSE) -> (reference out=w1434:refnum<vi>, error out=w1435:errorcluster)  [unwired: 1 in]
        n984 = Close Reference(reference=w1434, error in (no error)=w1435) -> ()  [unwired: 1 out]
        n985 = call "DATA ENCRYPT STRING FILE WRITE.vi"("error in (no error)"=w1427, "User Action"="User Pressed Heave UP", "main ref"=w1426) -> ("error out"=w1431:errorcluster)  [unwired: 6 in, 1 out]
        n986 = call "HEAVE WRITE FGV.vi"("Enum - Menu"=Heave_Write_enum."WRITE", "error in (no error)"=w1431, "main ref"=w1426) -> ("error out"=w1430:errorcluster)  [unwired: 8 in]
      }
      frame "Heave Up MM" {
        n987 = Unbundle By Name(w1437) -> ("Motion Module.Heave Up MM"=w1447:refnum<vi>)
        n988 = call "Heave Up Motion Module.vi"("error in (no error)"=w1439, "main ref"=w1437) -> ("error out"=w1438:errorcluster)  [unwired: 9 in]
        n989 = property class="Bool (strict)"(reference=w1447, "Value"=FALSE) -> (reference out=w1445:refnum<vi>, error out=w1446:errorcluster)  [unwired: 1 in]
        n990 = Close Reference(reference=w1445, error in (no error)=w1446) -> ()  [unwired: 1 out]
        n991 = call "DATA ENCRYPT STRING FILE WRITE.vi"("error in (no error)"=w1438, "User Action"="User Pressed Heave UP in Motion Module", "main ref"=w1437) -> ("error out"=w1442:errorcluster)  [unwired: 6 in, 1 out]
        n992 = call "HEAVE WRITE FGV.vi"("Enum - Menu"=Heave_Write_enum."WRITE", "error in (no error)"=w1442, "main ref"=w1437) -> ("error out"=w1441:errorcluster)  [unwired: 8 in]
      }
      frame "Heave Down Main" {
        n993 = call "Heave Down Main.vi"("error in (no error)"=w1450, "main ref"=w1448) -> ("error out"=w1449:errorcluster)  [unwired: 9 in]
        n994 = Unbundle By Name(w1448) -> ("Platform Settings.Heave Down Main"=w1458:refnum<vi>)
        n995 = property class="Bool (strict)"(reference=w1458, "Value"=FALSE) -> (reference out=w1456:refnum<vi>, error out=w1457:errorcluster)  [unwired: 1 in]
        n996 = Close Reference(reference=w1456, error in (no error)=w1457) -> ()  [unwired: 1 out]
        n997 = call "DATA ENCRYPT STRING FILE WRITE.vi"("error in (no error)"=w1449, "User Action"="User Pressed Heave DOWN", "main ref"=w1448) -> ("error out"=w1453:errorcluster)  [unwired: 6 in, 1 out]
        n998 = call "HEAVE WRITE FGV.vi"("Enum - Menu"=Heave_Write_enum."WRITE", "error in (no error)"=w1453, "main ref"=w1448) -> ("error out"=w1452:errorcluster)  [unwired: 8 in]
      }
      frame "Heave Down MM" {
        n999 = call "Heave Down Motion Module.vi"("error in (no error)"=w1461, "main ref"=w1459) -> ("error out"=w1460:errorcluster)  [unwired: 9 in]
        n1000 = Unbundle By Name(w1459) -> ("Motion Module.Heave Down MM"=w1469:refnum<vi>)
        n1001 = property class="Bool (strict)"(reference=w1469, "Value"=FALSE) -> (reference out=w1467:refnum<vi>, error out=w1468:errorcluster)  [unwired: 1 in]
        n1002 = Close Reference(reference=w1467, error in (no error)=w1468) -> ()  [unwired: 1 out]
        n1003 = call "DATA ENCRYPT STRING FILE WRITE.vi"("error in (no error)"=w1460, "User Action"="User Pressed Heave DOWN in Motion Module", "main ref"=w1459) -> ("error out"=w1464:errorcluster)  [unwired: 6 in, 1 out]
        n1004 = call "HEAVE WRITE FGV.vi"("Enum - Menu"=Heave_Write_enum."WRITE", "error in (no error)"=w1464, "main ref"=w1459) -> ("error out"=w1463:errorcluster)  [unwired: 8 in]
      }
      frame "Surge Backward Main" {
        n1005 = Unbundle By Name(w1470) -> ("Platform Settings.Surge Backward Main"=w1480:refnum<vi>)
        n1006 = call "Surge Backward Main.vi"("error in (no error)"=w1472, "main ref"=w1470) -> ("error out"=w1471:errorcluster)  [unwired: 9 in]
        n1007 = property class="Bool (strict)"(reference=w1480, "Value"=FALSE) -> (reference out=w1478:refnum<vi>, error out=w1479:errorcluster)  [unwired: 1 in]
        n1008 = Close Reference(reference=w1478, error in (no error)=w1479) -> ()  [unwired: 1 out]
        n1009 = call "DATA ENCRYPT STRING FILE WRITE.vi"("error in (no error)"=w1471, "User Action"="User Pressed Surge Backward", "main ref"=w1470) -> ("error out"=w1475:errorcluster)  [unwired: 6 in, 1 out]
        n1010 = call "HEAVE WRITE FGV.vi"("Enum - Menu"=Heave_Write_enum."WRITE", "error in (no error)"=w1475, "main ref"=w1470) -> ("error out"=w1474:errorcluster)  [unwired: 8 in]
      }
      frame "Surge Backward MM" {
        n1011 = Unbundle By Name(w1481) -> ("Motion Module.Surge Backward MM"=w1491:refnum<vi>)
        n1012 = call "Surge Backward Main.vi"("error in (no error)"=w1483, "main ref"=w1481) -> ("error out"=w1482:errorcluster)  [unwired: 9 in]
        n1013 = property class="Bool (strict)"(reference=w1491, "Value"=FALSE) -> (reference out=w1489:refnum<vi>, error out=w1490:errorcluster)  [unwired: 1 in]
        n1014 = Close Reference(reference=w1489, error in (no error)=w1490) -> ()  [unwired: 1 out]
        n1015 = call "DATA ENCRYPT STRING FILE WRITE.vi"("error in (no error)"=w1482, "User Action"="User Pressed Surge Backward in Motion Module", "main ref"=w1481) -> ("error out"=w1486:errorcluster)  [unwired: 6 in, 1 out]
        n1016 = call "HEAVE WRITE FGV.vi"("Enum - Menu"=Heave_Write_enum."WRITE", "error in (no error)"=w1486, "main ref"=w1481) -> ("error out"=w1485:errorcluster)  [unwired: 8 in]
      }
      frame "Surge Forward Main" {
        n1017 = Unbundle By Name(w1492) -> ("Platform Settings.Surge Forward Main"=w1502:refnum<vi>)
        n1018 = call "Surge Forward Main.vi"("error in (no error)"=w1494, "main ref"=w1492) -> ("error out"=w1493:errorcluster)  [unwired: 9 in]
        n1019 = property class="Bool (strict)"(reference=w1502, "Value"=FALSE) -> (reference out=w1500:refnum<vi>, error out=w1501:errorcluster)  [unwired: 1 in]
        n1020 = Close Reference(reference=w1500, error in (no error)=w1501) -> ()  [unwired: 1 out]
        n1021 = call "DATA ENCRYPT STRING FILE WRITE.vi"("error in (no error)"=w1493, "User Action"="User Pressed Surge Forward", "main ref"=w1492) -> ("error out"=w1497:errorcluster)  [unwired: 6 in, 1 out]
        n1022 = call "HEAVE WRITE FGV.vi"("Enum - Menu"=Heave_Write_enum."WRITE", "error in (no error)"=w1497, "main ref"=w1492) -> ("error out"=w1496:errorcluster)  [unwired: 8 in]
      }
      frame "Surge Forward MM" {
        n1023 = Unbundle By Name(w1503) -> ("Motion Module.Surge Forward MM"=w1513:refnum<vi>)
        n1024 = call "Surge Forward MM.vi"("error in (no error)"=w1505, "main ref"=w1503) -> ("error out"=w1504:errorcluster)  [unwired: 9 in]
        n1025 = property class="Bool (strict)"(reference=w1513, "Value"=FALSE) -> (reference out=w1511:refnum<vi>, error out=w1512:errorcluster)  [unwired: 1 in]
        n1026 = Close Reference(reference=w1511, error in (no error)=w1512) -> ()  [unwired: 1 out]
        n1027 = call "DATA ENCRYPT STRING FILE WRITE.vi"("error in (no error)"=w1504, "User Action"="User Pressed Surge Forward in Motion Module", "main ref"=w1503) -> ("error out"=w1508:errorcluster)  [unwired: 6 in, 1 out]
        n1028 = call "HEAVE WRITE FGV.vi"("Enum - Menu"=Heave_Write_enum."WRITE", "error in (no error)"=w1508, "main ref"=w1503) -> ("error out"=w1507:errorcluster)  [unwired: 8 in]
      }
      frame "Sway Left Main" {
        n1029 = call "Sway Left Main.vi"("error in (no error)"=w1517, "main ref"=w1515) -> ("error out"=w1516:errorcluster)  [unwired: 9 in]
        n1030 = Unbundle By Name(w1515) -> ("Platform Settings.Sway Left Main"=w1524:refnum<vi>)
        n1031 = property class="Bool (strict)"(reference=w1524, "Value"=FALSE) -> (reference out=w1522:refnum<vi>, error out=w1523:errorcluster)  [unwired: 1 in]
        n1032 = Close Reference(reference=w1522, error in (no error)=w1523) -> ()  [unwired: 1 out]
        n1033 = call "DATA ENCRYPT STRING FILE WRITE.vi"("error in (no error)"=w1516, "User Action"="User Pressed Sway Left ", "main ref"=w1515) -> ("error out"=w1519:errorcluster)  [unwired: 6 in, 1 out]
        n1034 = call "SWAY WRITE FGV.vi"("Enum - Menu"=Sway_Write_enum."WRITE", "error in (no error)"=w1519, "main ref"=w1515) -> ("error out"=w1518:errorcluster)  [unwired: 8 in]
      }
      frame "Sway Left MM" {
        n1035 = call "Sway Left MM.vi"("error in (no error)"=w1528, "main ref"=w1526) -> ("error out"=w1527:errorcluster)  [unwired: 9 in]
        n1036 = Unbundle By Name(w1526) -> ("Motion Module.Sway Left MM"=w1535:refnum<vi>)
        n1037 = property class="Bool (strict)"(reference=w1535, "Value"=FALSE) -> (reference out=w1533:refnum<vi>, error out=w1534:errorcluster)  [unwired: 1 in]
        n1038 = Close Reference(reference=w1533, error in (no error)=w1534) -> ()  [unwired: 1 out]
        n1039 = call "DATA ENCRYPT STRING FILE WRITE.vi"("error in (no error)"=w1527, "User Action"="User Pressed Sway Left in MM", "main ref"=w1526) -> ("error out"=w1530:errorcluster)  [unwired: 6 in, 1 out]
        n1040 = call "SWAY WRITE FGV.vi"("Enum - Menu"=Sway_Write_enum."WRITE", "error in (no error)"=w1530, "main ref"=w1526) -> ("error out"=w1529:errorcluster)  [unwired: 8 in]
      }
      frame "Sway Right MM" {
        n1041 = call "Sway Right MM.vi"("error in (no error)"=w1539, "main ref"=w1537) -> ("error out"=w1538:errorcluster)  [unwired: 9 in]
        n1042 = Unbundle By Name(w1537) -> ("Motion Module.Sway Right MM"=w1546:refnum<vi>)
        n1043 = property class="Bool (strict)"(reference=w1546, "Value"=FALSE) -> (reference out=w1544:refnum<vi>, error out=w1545:errorcluster)  [unwired: 1 in]
        n1044 = Close Reference(reference=w1544, error in (no error)=w1545) -> ()  [unwired: 1 out]
        n1045 = call "DATA ENCRYPT STRING FILE WRITE.vi"("error in (no error)"=w1538, "User Action"="User Pressed Sway Right in MM", "main ref"=w1537) -> ("error out"=w1541:errorcluster)  [unwired: 6 in, 1 out]
        n1046 = call "SWAY WRITE FGV.vi"("Enum - Menu"=Sway_Write_enum."WRITE", "error in (no error)"=w1541, "main ref"=w1537) -> ("error out"=w1540:errorcluster)  [unwired: 8 in]
      }
      frame "Sway Right Main" {
        n1047 = call "Sway Right Main.vi"("error in (no error)"=w1550, "main ref"=w1548) -> ("error out"=w1549:errorcluster)  [unwired: 9 in]
        n1048 = Unbundle By Name(w1548) -> ("Platform Settings.Sway Right Main"=w1557:refnum<vi>)
        n1049 = property class="Bool (strict)"(reference=w1557, "Value"=FALSE) -> (reference out=w1555:refnum<vi>, error out=w1556:errorcluster)  [unwired: 1 in]
        n1050 = Close Reference(reference=w1555, error in (no error)=w1556) -> ()  [unwired: 1 out]
        n1051 = call "DATA ENCRYPT STRING FILE WRITE.vi"("error in (no error)"=w1549, "User Action"="User Pressed Sway Right", "main ref"=w1548) -> ("error out"=w1552:errorcluster)  [unwired: 6 in, 1 out]
        n1052 = call "SWAY WRITE FGV.vi"("Enum - Menu"=Sway_Write_enum."WRITE", "error in (no error)"=w1552, "main ref"=w1548) -> ("error out"=w1551:errorcluster)  [unwired: 8 in]
      }
      frame "Manual Write Heave & Surge" {
        n1053 = Unbundle By Name(w1558) -> ("Heave AND Surge.Manual Write"=w1567:refnum<vi>)
        n1054 = property class="Bool (strict)"(reference=w1567, "Value"=FALSE) -> (reference out=w1565:refnum<vi>, error out=w1566:errorcluster)  [unwired: 1 in]
        n1055 = Close Reference(reference=w1565, error in (no error)=w1566) -> ()  [unwired: 1 out]
        n1056 = call "DATA ENCRYPT STRING FILE WRITE.vi"("error in (no error)"=w1559, "User Action"="User Pressed Manual Write Heave and Surge", "main ref"=w1558) -> ("error out"=w1562:errorcluster)  [unwired: 6 in, 1 out]
        n1057 = call "HEAVE WRITE FGV.vi"("Enum - Menu"=Heave_Write_enum."WRITE", "error in (no error)"=w1562, "main ref"=w1558) -> ("error out"=w1561:errorcluster)  [unwired: 8 in]
      }
      frame "Manual Write SWAY" {
        n1058 = Unbundle By Name(w1569) -> ("SWAY.Manual Write SWAY"=w1577:refnum<vi>)
        n1059 = property class="Bool (strict)"(reference=w1577, "Value"=FALSE) -> (reference out=w1575:refnum<vi>, error out=w1576:errorcluster)  [unwired: 1 in]
        n1060 = Close Reference(reference=w1575, error in (no error)=w1576) -> ()  [unwired: 1 out]
        n1061 = call "DATA ENCRYPT STRING FILE WRITE.vi"("error in (no error)"=w1570, "User Action"="User Pressed Manual Write Sway", "main ref"=w1569) -> ("error out"=w1572:errorcluster)  [unwired: 6 in, 1 out]
        n1062 = call "SWAY WRITE FGV.vi"("Enum - Menu"=Sway_Write_enum."WRITE", "error in (no error)"=w1572, "main ref"=w1569) -> ("error out"=w1571:errorcluster)  [unwired: 8 in]
      }
      frame "Load En" {
        # "zNL 2"
        n1063 = Unbundle By Name(w1579) -> ("Main Screen.Load En"=w1584:refnum<vi>)
        n1064 = property class="Bool (strict)"(reference=w1584) -> (reference out=w1582:refnum<vi>, error out=w1583:errorcluster, "Value"=w1578:bool)  [unwired: 1 in]
        n1065 = Close Reference(reference=w1582, error in (no error)=w1583) -> ()  [unwired: 1 out]
        n1066 = case shown="False" w1578 {
          tunnel: [w1596 w1606] -> w1580
          tunnel: w1581 -> [w1598 w1605]
          tunnel: w1579 -> [w1586 w1600]
          tunnel: w1579 -> [w1594 _]
          tunnel: w1579 -> [w1593 _]
          frame False {
            n1067 = call "DATA ENCRYPT STRING FILE WRITE.vi"("error in (no error)"=w1598, "User Action"="User Pressed UnLoad on Main Screen", "main ref"=w1586) -> ("error out"=w1587:errorcluster)  [unwired: 6 in, 1 out]
            n1068 = call "Stall Data Flow.vim"("value in"=w1587, "milliseconds to wait"=u32 2000) -> ("value out"=w1592:errorcluster)  [unwired: 1 out]
            n1069 = Unbundle By Name(w1586) -> ("Main Screen.zNL 2"=w1590:refnum<vi>)
            n1070 = property class="Bool (strict)"(reference=w1590, "DisabledEnum"=T13."Enabled" ("Disabled")) -> (reference out=w1588:refnum<vi>, error out=w1589:errorcluster)  [unwired: 1 in]
            n1071 = call "PID UNLOAD.vi"("error in (no error)"=w1592, "main ref"=w1593) -> ("error out"=w1595:errorcluster)  [unwired: 9 in]
            n1072 = Close Reference(reference=w1588, error in (no error)=w1589) -> ()  [unwired: 1 out]
            n1073 = call "HEAVE WRITE FGV.vi"("Enum - Menu"=Heave_Write_enum."WRITE", "error in (no error)"=w1595, "main ref"=w1594) -> ("error out"=w1596:errorcluster)  [unwired: 8 in]
          }
          frame True {
            n1074 = call "DATA ENCRYPT STRING FILE WRITE.vi"("error in (no error)"=w1605, "User Action"="User Pressed Load on Main Screen", "main ref"=w1600) -> ("error out"=w1606:errorcluster)  [unwired: 6 in, 1 out]
            n1075 = Unbundle By Name(w1600) -> ("Main Screen.zNL 2"=w1604:refnum<vi>)
            n1076 = property class="Bool (strict)"(reference=w1604, "DisabledEnum"=T13."Disabled and Grayed Out" ("Disabled")) -> (reference out=w1602:refnum<vi>, error out=w1603:errorcluster)  [unwired: 1 in]
            n1077 = Close Reference(reference=w1602, error in (no error)=w1603) -> ()  [unwired: 1 out]
          }
        }
      }
      frame "apply load" {
        n1078 = Unbundle By Name(w1609) -> ("Main Screen.Load En"=w1614:refnum<vi>)
        n1079 = property class="Bool (strict)"(reference=w1614) -> (reference out=w1612:refnum<vi>, error out=w1613:errorcluster, "Value"=w1608:bool)  [unwired: 1 in]
        n1080 = Close Reference(reference=w1612, error in (no error)=w1613) -> ()  [unwired: 1 out]
        n1081 = case shown="False" w1608 {
          tunnel: [w1621 w1628] -> w1610
          tunnel: w1611 -> [w1624 w1627]
          tunnel: w1609 -> [w1623 w1626]
          tunnel: w1609 -> [w1618 _]
          tunnel: w1609 -> [w1617 _]
          frame False {
            n1082 = call "DATA ENCRYPT STRING FILE WRITE.vi"("error in (no error)"=w1624, "User Action"="User Pressed UnLoad on Service Screen", "main ref"=w1623) -> ("error out"=w1620:errorcluster)  [unwired: 6 in, 1 out]
            n1083 = call "Stall Data Flow.vim"("value in"=w1620, "milliseconds to wait"=u32 2000) -> ("value out"=w1616:errorcluster)  [unwired: 1 out]
            n1084 = call "PID UNLOAD.vi"("error in (no error)"=w1616, "main ref"=w1617) -> ("error out"=w1619:errorcluster)  [unwired: 9 in]
            n1085 = call "HEAVE WRITE FGV.vi"("Enum - Menu"=Heave_Write_enum."WRITE", "error in (no error)"=w1619, "main ref"=w1618) -> ("error out"=w1621:errorcluster)  [unwired: 8 in]
          }
          frame True {
            n1086 = call "DATA ENCRYPT STRING FILE WRITE.vi"("error in (no error)"=w1627, "User Action"="User Pressed Load on Service Screen", "main ref"=w1626) -> ("error out"=w1628:errorcluster)  [unwired: 6 in, 1 out]
          }
        }
      }
      frame "BACK" {
        w1635 = FALSE ("Value")
        n1087 = Unbundle By Name(w1630) -> ("Main Screen.BACK"=w1655:refnum<vi>)
        n1088 = property class="Bool (strict)"(reference=w1655, "Value"=FALSE) -> (reference out=w1653:refnum<vi>, error out=w1654:errorcluster)  [unwired: 1 in]
        n1089 = Close Reference(reference=w1653, error in (no error)=w1654) -> ()  [unwired: 1 out]
        n1090 = call "DATA ENCRYPT STRING FILE WRITE.vi"("error in (no error)"=w1652, "User Action"="User Pressed Back on Main Screen", "main ref"=w1630) -> ("error out"=w1650:errorcluster)  [unwired: 6 in, 1 out]
        n1091 = Unbundle By Name(w1630) -> ("Main Home Screen.MainPage"=w1642:refnum<vi>)
        n1092 = Unbundle By Name(w1630) -> ("Main Screen.Start Test"=w1638:refnum<vi>)
        n1093 = Unbundle By Name(w1630) -> ("Main Screen.STOP"=w1637:refnum<vi>)
        n1094 = Unbundle By Name(w1630) -> ("Main Home Screen.GUI"=w1646:refnum<vi>)
        n1095 = property class="TabCtl (strict)"(reference=w1642, "Value"=T5."HOME") -> (reference out=w1644:refnum<vi>, error out=w1643:errorcluster)  [unwired: 1 in]
        n1096 = property class="TabCtl (strict)"(reference=w1646, "Value"=T4."Setup") -> (reference out=w1648:refnum<vi>, error out=w1647:errorcluster)  [unwired: 1 in]
        n1097 = property class="Bool (strict)"(reference=w1638, "Visible"=TRUE ("Value"), "Value"=FALSE) -> (reference out=w1633:refnum<vi>, error out=w1639:errorcluster)  [unwired: 1 in]
        n1098 = property class="Bool (strict)"(reference=w1637, "Value"=w1635, "Visible"=w1635) -> (reference out=w1632:refnum<vi>, error out=w1636:errorcluster)  [unwired: 1 in]
        n1099 = Close Reference(reference=w1648, error in (no error)=w1647) -> ()  [unwired: 1 out]
        n1100 = Close Reference(reference=w1644, error in (no error)=w1643) -> ()  [unwired: 1 out]
        n1101 = Close Reference(reference=w1633, error in (no error)=w1639) -> ()  [unwired: 1 out]
        n1102 = Close Reference(reference=w1632, error in (no error)=w1636) -> ()  [unwired: 1 out]
        n1103 = call "Reinitial Parameter After Test.vi"("error in (no error)"=w1650, "main ref"=w1630) -> ("error out"=w1631:errorcluster)  [unwired: 9 in]
      }
      frame "Start Test" {
        n1104 = call "Test Start Sequence.vi"("error in (no error)"=w1658, "Data Cluster"=w1656) -> ("error out"=w1657:errorcluster)  [unwired: 9 in]
      }
      frame "STOP" {
        n1105 = Unbundle By Name(w1660) -> ("Main Screen.Load En"=w1673:refnum<vi>)
        n1106 = Unbundle By Name(w1660) -> ("Main Screen.CZ FF"=w1668:refnum<vi>)
        n1107 = Unbundle By Name(w1660) -> ("Main Screen.zFF"=w1665:refnum<vi>)
        n1108 = property class="Bool (strict)"(reference=w1673, "DisabledEnum"=T13."Disabled and Grayed Out" ("Disabled")) -> (reference out=w1661:refnum<vi>, error out=w1672:errorcluster)  [unwired: 1 in]
        n1109 = property class="Bool (strict)"(reference=w1668, "DisabledEnum"=T13."Disabled and Grayed Out" ("Disabled"), "Value"=FALSE ("Visible")) -> (reference out=w1667:refnum<vi>, error out=w1669:errorcluster)  [unwired: 1 in]
        n1110 = property class="Bool (strict)"(reference=w1665, "DisabledEnum"=T13."Disabled and Grayed Out" ("Disabled"), "Value"=FALSE ("Visible")) -> (reference out=w1666:refnum<vi>, error out=w1664:errorcluster)  [unwired: 1 in]
        n1111 = Close Reference(reference=w1661, error in (no error)=w1672) -> ()  [unwired: 1 out]
        n1112 = Close Reference(reference=w1667, error in (no error)=w1669) -> ()  [unwired: 1 out]
        n1113 = Close Reference(reference=w1666, error in (no error)=w1664) -> ()  [unwired: 1 out]
        n1114 = call "Test Stop.vi"("error in (no error)"=w1674, "Data Cluster"=w1660) -> ("error out"=w1675:errorcluster)  [unwired: 9 in]
      }
      frame "PlaceModule" {
        n1115 = call "Place Module.vi"("error in (no error)"=w1678, "main ref"=w1676) -> ("error out"=w1677:errorcluster)  [unwired: 9 in]
      }
      frame "Stage Homing" {
        n1116 = call "HOMINING.vi"("error in (no error)"=w1681, "main ref"=w1679) -> ("error out"=w1680:errorcluster)  [unwired: 9 in]
      }
      frame "Clear 3" {
        n1117 = Unbundle By Name(w1683) -> ("Loading.Stribeck Table  For loading"=w1693:refnum<vi>)
        n1118 = Unbundle By Name(w1683) -> ("Loading.Clear 3"=w1684:refnum<vi>)
        n1119 = property class="Bool (strict)"(reference=w1684, "Value"=FALSE) -> (reference out=w1686:refnum<vi>, error out=w1685:errorcluster)  [unwired: 1 in]
        n1120 = call "DATA ENCRYPT STRING FILE WRITE.vi"("error in (no error)"=w1689, "User Action"="User Pressed Clear  on Step Load Sequence", "main ref"=w1683) -> ("error out"=w1688:errorcluster)  [unwired: 6 in, 1 out]
        n1121 = property class="Tbl (strict)"(reference=w1693, "Value"=string[][] []) -> (reference out=w1691:refnum<vi>, error out=w1692:errorcluster)  [unwired: 1 in]
        n1122 = Close Reference(reference=w1686, error in (no error)=w1685) -> ()  [unwired: 1 out]
        n1123 = Close Reference(reference=w1691, error in (no error)=w1692) -> ()  [unwired: 1 out]
      }
      frame "Set WTD" {
        n1124 = Unbundle By Name(w1695) -> ("Loading.Stribeck Table  For loading"=w1705:refnum<vi>)
        n1125 = Unbundle By Name(w1695) -> ("Loading.Clear 3"=w1696:refnum<vi>)
        n1126 = property class="Bool (strict)"(reference=w1696, "Value"=FALSE) -> (reference out=w1698:refnum<vi>, error out=w1697:errorcluster)  [unwired: 1 in]
        n1127 = call "DATA ENCRYPT STRING FILE WRITE.vi"("error in (no error)"=w1701, "User Action"="User Pressed Clear  on Step Load Sequence", "main ref"=w1695) -> ("error out"=w1700:errorcluster)  [unwired: 6 in, 1 out]
        n1128 = property class="Tbl (strict)"(reference=w1705, "Value"=string[][] []) -> (reference out=w1703:refnum<vi>, error out=w1704:errorcluster)  [unwired: 1 in]
        n1129 = Close Reference(reference=w1698, error in (no error)=w1697) -> ()  [unwired: 1 out]
        n1130 = Close Reference(reference=w1703, error in (no error)=w1704) -> ()  [unwired: 1 out]
      }
      frame "Import 2" {
        n1131 = call "File Dialog"("start path"=path "C:/LAB-IQ 150/User Defined Protocol", "error in"=w1713) -> ("selected path"=w1707:path, "cancelled"=w1710:bool, "error out"=w1712:errorcluster)  [unwired: 10 in, 1 out]
        n1132 = call <vilib>:"Clear Errors.vi"("error in (no error)"=w1712) -> ("error out"=w1709:errorcluster)  [unwired: 5 in, 1 out]
        n1133 = case shown="False" w1710 {
          tunnel: w1709 -> [w1723 w1724]
          tunnel: [w1715 w1724] -> w1708
          tunnel: w1707 -> [w1722 _]
          tunnel: w1706 -> [w1717 _]
          frame False {
            n1134 = call-poly <vilib>:"Read Delimited Spreadsheet.vi"("file path (dialog if empty)"=w1722, "error in (no error)"=w1723, "delimiter (\\t)"=":" ("delimiter (\\t)")) -> ("all rows"=w1714:string[][], "error out"=w1716:errorcluster)  [unwired: 7 in, 4 out]
            n1135 = Unbundle By Name(w1717) -> ("Motion Module.StepTable For Speed"=w1720:refnum<vi>)
            n1136 = property class="Tbl (strict)"(reference=w1720, error in=w1716, "Value"=w1714) -> (reference out=w1718:refnum<vi>, error out=w1719:errorcluster)
            n1137 = Close Reference(reference=w1718, error in (no error)=w1719) -> (error out=w1715:errorcluster)
          }
          frame True {
          }
        }
      }
      frame "Save 2" {
        n1138 = Unbundle By Name(w1728) -> ("Motion Module.StepTable For Speed"=w1743:refnum<vi>)
        n1139 = property class="Tbl (strict)"(reference=w1743) -> (reference out=w1741:refnum<vi>, error out=w1742:errorcluster, "Value"=w1739:string[][])  [unwired: 1 in]
        n1140 = call "File Dialog2"("start path"=path "C:/LAB-IQ 150/User Defined Protocol", "error in"=w1733) -> ("selected path"=w1736:path, "error out"=w1735:errorcluster)  [unwired: 10 in, 2 out]
        n1141 = call <vilib>:"Clear Errors.vi"("error in (no error)"=w1735) -> ("error out"=w1734:errorcluster)  [unwired: 5 in, 1 out]
        n1142 = Close Reference(reference=w1741, error in (no error)=w1742) -> ()  [unwired: 1 out]
        n1143 = call-poly <vilib>:"Write Delimited Spreadsheet.vi"("file path (dialog if empty)"=w1736, "2D data"=w1739, "append to file? (new file:F)"=TRUE, "error in (no error)"=w1734, "delimiter (\\t)"=":" ("delimiter (\\t)")) -> ("error out"=w1732:errorcluster)  [unwired: 9 in, 1 out]
        n1144 = call <vilib>:"Clear Errors.vi"("error in (no error)"=w1732) -> ("error out"=w1727:errorcluster)  [unwired: 5 in, 1 out]
        n1145 = Unbundle By Name(w1728) -> ("Motion Module.Save 2"=w1729:refnum<vi>)
        n1146 = property class="Bool (strict)"(reference=w1729, error in=w1727, "Value"=FALSE) -> (reference out=w1731:refnum<vi>, error out=w1730:errorcluster)
        n1147 = Close Reference(reference=w1731, error in (no error)=w1730) -> (error out=w1726:errorcluster)
      }
      frame "Calculate Rotary" {
        n1148 = Unbundle By Name(w1749) -> ("Motion Module.StepTable For Speed"=w1762:refnum<vi>)
        n1149 = Unbundle By Name(w1749) -> ("Motion Module.Wear Track Diameter (mm)"=w1754:refnum<vi>)
        n1150 = property class="Tbl (strict)"(reference=w1762, error in=w1745) -> (reference out=w1760:refnum<vi>, error out=w1761:errorcluster, "Value"=w1759:string[][])
        n1151 = property class="DigNum (strict)"(reference=w1754) -> (reference out=w1756:refnum<vi>, error out=w1755:errorcluster, "Value"=w1753:dbl)  [unwired: 1 in]
        n1152 = Close Reference(reference=w1760, error in (no error)=w1761) -> ()  [unwired: 1 out]
        n1153 = Index Array(array=w1759, index (col)=2 ("disabled index (col)")) -> (element=w1757:string[])  [unwired: 1 in]
        n1154 = Close Reference(reference=w1756, error in (no error)=w1755) -> ()  [unwired: 1 out]
        n1155 = for {
          tunnel: w1757 -> [w1767] mode=indexing
          tunnel: w1753 -> [w1766]
          tunnel: [w1763] -> w1746 mode=indexing
          n1156 = Fract/Exp String To Number(string=w1767) -> (number=w1765:dbl)  [unwired: 3 in, 1 out]
          n1157 = call "rpm to mm_sec conversion.vi"("Wear Track Diameter"=w1766, "Initial Speed (RPM)"=w1765) -> ("Enter initial Velocity (m/s)  4"=w1764:dbl)  [unwired: 7 in, 2 out]
          n1158 = Number To Fractional String(number=w1764) -> (F-format string=w1763:string)  [unwired: 3 in]
        }
        n1159 = Unbundle By Name(w1749) -> ("Motion Module.StepTable For Speed 3"=w1750:refnum<vi>)
        n1160 = Insert Into Array(array=string[][] [] ("Value"), new element=w1746) -> (w1747:string[][])  [unwired: 2 in]
        n1161 = property class="Tbl (strict)"(reference=w1750, "Value"=w1747) -> (reference out=w1752:refnum<vi>, error out=w1751:errorcluster)  [unwired: 1 in]
        n1162 = Close Reference(reference=w1752, error in (no error)=w1751) -> (error out=→"error out":errorcluster)
      }
      frame "Error" {
        # "#CodeRecommended - If you ever change the name of this \"Error\" message, you'll need to update the name in the Check Loop Error.vi as well."
        # "#CodeRecommended - Consider creating a system for logging errors in some way. These errors are for notification purposes only. Handling of specific errors should be performed in the message frames that generated the error."
        # "Error - Display an error dialog. This message is sent by the \"Error Handler\" VIs at the end of other loops in this application."
        n1163 = Variant To Data(error in=w1774, type=errorcluster {"status"=FALSE, "code"=0, "source"=""} ("error constant"), Variant=w1772) -> (data=w1770:errorcluster, error out=w1769:errorcluster)
        n1164 = call <vilib>:"Simple Error Handler.vi"("error in (no error)"=w1770) -> ()  [unwired: 4 in, 5 out]
        n1165 = Merge Errors(w1769) -> (w1768:errorcluster)
      }
      frame "Confirm Quit" {
        # "#CodeNeeded - If you want to provide an \"Are you sure\" dialog (or some other notification) before the application exits, place that code here. This message is typically sent from a Panel Close? event."
        # "Confirm Quit - Message that can confirm whether or not the user wants to exit the application."
        n1166 = call-poly "Enqueue Message.vi"("Priority Message? (F)"=TRUE, "error in (no error)"=w1781, "Message"="Exit", "Message Queue"=w1778) -> ("error out"=w1779:errorcluster)  [unwired: 6 in, 1 out]
        n1167 = Merge Errors(w1779) -> (w1780:errorcluster)
      }
      frame "Exit" {
        # "Stop the VI"
        # "Release the message queue reference"
        # "#CodeNeeded - Add any required cleanup code here. Note that if 'Exit' was called as a result of an error, an error dialog will be displayed. Add any custom error handling for an 'Exit' condition here as well."
        # "Exit - Exit the application."
        n1168 = call "Fire User Event - Stop.vi"("User Event - Stop"=w1784) -> ("error out"=w1783:errorcluster)  [unwired: 10 in]
        n1169 = Release Queue(queue=w1789, error in (no error)=w1782) -> (error out=w1786:errorcluster)  [unwired: 1 in, 2 out]
        n1170 = Merge Errors(w1783, w1786) -> (w1785:errorcluster)
      }
      frame Default {
        # "'Default' case only runs if there is a message that isn't defined in any of the other cases.  Output a programming error."
        n1171 = xnode "Error Ring"("parameter 0"=w1790) -> ("error out"=w1791:errorcluster)
      }
    }
    n1172 = call "LAB-IQ Error Handler - Message Handling Loop.vi"("error in (no error)"=w863, "Message Queue"=w865) -> ("dup error in"=w864:errorcluster)  [unwired: 8 in, 1 out]
  }
  n1173 = while {
    shift-right: [w1810] -> _
    shift-left: w14 -> [w1811]
    tunnel: [w1804] -> w24
    tunnel: w23 -> [w1802]
    tunnel: w4 -> [w1801]
    tunnel: w13 -> [w1800]
    stop <- w1809 stop-if-true
    # "Load  Handling Loop"
    n1174 = call "Dequeue Message.vi"("error in (no error)"=w1801, "Message Queue"=w1802) -> ("error out"=w1808:errorcluster, "Message Data"=w1806:variant, "Message"=w1807:string, "dup Message Queue"=w1805:refnum<queue>)  [unwired: 6 in]
    n1175 = case "Message Cases" shown="\"Load Main\"" w1807 {
      selector: w1807 -> [_ _ _ _ _ w1865]
      tunnel: w1805 -> [w1812 w1825 _ w1854 w1864 _]
      tunnel: w1808 -> [w1815 w1823 w1841 w1856 w1858 _]
      tunnel: [w1816 w1826 w1835 w1842 w1860 w1866] -> w1803
      tunnel: w1811 -> [w1814 w1818 w1840 w1851 w1863 w1867]
      tunnel: [w1814 w1818 w1840 w1851 w1863 w1867] -> w1810
      tunnel: [_ _ _ _ TRUE _] -> w1809
      tunnel: w1806 -> [_ _ w1839 _ _ _]
      tunnel: w1800 -> [_ _ _ _ w1857 _]
      frame "init" {
        # "Bundle control references and a sample string value."
        # "Initialize - All initialization work should take place in this message, since other loops can potentially enqueue messages that execute immediately after this one."
        n1176 = call-poly "Enqueue Message.vi"("error in (no error)"=w1815, "Message"="Load Main", "Message Queue"=w1812) -> ("error out"=w1816:errorcluster)  [unwired: 7 in, 1 out]
      }
      frame "Load Main" {
        n1177 = call "LOAD CELL READ.vi"("error in (no error)"=w1823, "main ref"=w1818) -> ("error out"=w1819:errorcluster)  [unwired: 9 in]
        n1178 = call <vilib>:"Clear Errors.vi"("error in (no error)"=w1819) -> ("error out"=w1817:errorcluster)  [unwired: 5 in, 1 out]
        n1179 = Unbundle By Name(w1818) -> ("Main Home Screen.EXIT"=w1824:refnum<vi>)
        n1180 = property class="Bool (strict)"(reference=w1824) -> (reference out=w1821:refnum<vi>, error out=w1822:errorcluster, "Value"=w1820:bool)  [unwired: 1 in]
        n1181 = Close Reference(reference=w1821, error in (no error)=w1822) -> ()  [unwired: 1 out]
        n1182 = case shown="False" w1820 {
          tunnel: [w1829 w1833] -> w1826
          tunnel: w1825 -> [w1828 w1832]
          tunnel: w1817 -> [w1827 w1831]
          frame True {
            n1183 = call-poly "Enqueue Message.vi"("error in (no error)"=w1827, "Message"="Confirm Quit", "Message Queue"=w1828) -> ("error out"=w1829:errorcluster)  [unwired: 7 in, 1 out]
          }
          frame False {
            n1184 = call-poly "Enqueue Message.vi"("error in (no error)"=w1831, "Message"="Load Main", "Message Queue"=w1832) -> ("error out"=w1833:errorcluster)  [unwired: 7 in, 1 out]
          }
        }
      }
      frame "Error" {
        # "#CodeRecommended - If you ever change the name of this \"Error\" message, you'll need to update the name in the Check Loop Error.vi as well."
        # "#CodeRecommended - Consider creating a system for logging errors in some way. These errors are for notification purposes only. Handling of specific errors should be performed in the message frames that generated the error."
        # "Error - Display an error dialog. This message is sent by the \"Error Handler\" VIs at the end of other loops in this application."
        n1185 = Variant To Data(error in=w1841, type=errorcluster {"status"=FALSE, "code"=0, "source"=""} ("error constant"), Variant=w1839) -> (data=w1837:errorcluster, error out=w1836:errorcluster)
        n1186 = call <vilib>:"Simple Error Handler.vi"("error in (no error)"=w1837) -> ()  [unwired: 4 in, 5 out]
        n1187 = Merge Errors(w1836) -> (w1835:errorcluster)
      }
      frame "Confirm Quit" {
        # "#CodeNeeded - If you want to provide an \"Are you sure\" dialog (or some other notification) before the application exits, place that code here. This message is typically sent from a Panel Close? event."
        # "Confirm Quit - Message that can confirm whether or not the user wants to exit the application."
        n1188 = call-poly "Enqueue Message.vi"("Priority Message? (F)"=TRUE, "error in (no error)"=w1856, "Message"="Exit", "Message Queue"=w1854) -> ("error out"=w1855:errorcluster)  [unwired: 6 in, 1 out]
        n1189 = Merge Errors(w1855) -> (w1847:errorcluster)
        n1190 = call <vilib>:"Clear Errors.vi"("error in (no error)"=w1847) -> ("error out"=w1843:errorcluster)  [unwired: 5 in, 1 out]
        n1191 = call "LOAD CELL FGV MAIN.vi"("Enum"=T14."UNINITIAL", "error in (no error)"=w1843, "main ref"=w1851) -> ("error IO"=w1850:errorcluster)  [unwired: 8 in]
        n1192 = call "Stall Data Flow.vim"("value in"=w1850, "milliseconds to wait"=u32 1000) -> ("value out"=w1845:errorcluster)  [unwired: 1 out]
        n1193 = call "LOAD CELL FGV MAIN.vi"("Enum"=T14."DELETEHANDLE", "error in (no error)"=w1845, "main ref"=w1851) -> ("error IO"=w1846:errorcluster)  [unwired: 8 in]
        n1194 = call <vilib>:"Clear Errors.vi"("error in (no error)"=w1846) -> ("error out"=w1842:errorcluster)  [unwired: 5 in, 1 out]
      }
      frame "Exit" {
        # "Stop the VI"
        # "Release the message queue reference"
        # "#CodeNeeded - Add any required cleanup code here. Note that if 'Exit' was called as a result of an error, an error dialog will be displayed. Add any custom error handling for an 'Exit' condition here as well."
        # "Exit - Exit the application."
        n1195 = call "Fire User Event - Stop.vi"("User Event - Stop"=w1857) -> ("error out"=w1859:errorcluster)  [unwired: 10 in]
        n1196 = Release Queue(queue=w1864, error in (no error)=w1858) -> (error out=w1861:errorcluster)  [unwired: 1 in, 2 out]
        n1197 = Merge Errors(w1859, w1861) -> (w1860:errorcluster)
      }
      frame Default {
        # "'Default' case only runs if there is a message that isn't defined in any of the other cases.  Output a programming error."
        n1198 = xnode "Error Ring"("parameter 0"=w1865) -> ("error out"=w1866:errorcluster)
      }
    }
    n1199 = call "LAB-IQ Error Handler - Message Handling Loop.vi"("error in (no error)"=w1803, "Message Queue"=w1805) -> ("dup error in"=w1804:errorcluster)  [unwired: 8 in, 1 out]
  }
  n1200 = while {
    shift-right: [w1885] -> _
    shift-left: w14 -> [w1886]
    tunnel: [w1879] -> w21
    tunnel: w22 -> [w1877]
    tunnel: w4 -> [w1876]
    tunnel: w13 -> [w1875]
    stop <- w1884 stop-if-true
    # "Sway Motor  Handling Loop"
    n1201 = call "Dequeue Message.vi"("error in (no error)"=w1876, "Message Queue"=w1877) -> ("error out"=w1883:errorcluster, "Message Data"=w1881:variant, "Message"=w1882:string, "dup Message Queue"=w1880:refnum<queue>)  [unwired: 6 in]
    n1202 = case "Message Cases" shown="\"Sway Main\"" w1882 {
      selector: w1882 -> [_ _ _ _ _ w1970]
      tunnel: w1880 -> [w1898 w1927 _ w1957 w1969 _]
      tunnel: w1883 -> [w1900 w1908 w1954 w1961 w1963 _]
      tunnel: [w1901 w1928 w1948 w1959 w1965 w1971] -> w1878
      tunnel: w1886 -> [w1889 w1902 w1953 w1960 w1968 w1972]
      tunnel: [w1889 w1902 w1953 w1960 w1968 w1972] -> w1885
      tunnel: [_ _ _ _ TRUE _] -> w1884
      tunnel: w1881 -> [_ _ w1952 _ _ _]
      tunnel: w1875 -> [_ _ _ _ w1962 _]
      frame "init" {
        # "Initialize - All initialization work should take place in this message, since other loops can potentially enqueue messages that execute immediately after this one."
        n1203 = call "SWAY WRITE FGV.vi"("Enum - Menu"=Sway_Write_enum."INIT", "error in (no error)"=w1900, "main ref"=w1889) -> ("error out"=w1897:errorcluster)  [unwired: 8 in]
        n1204 = call <vilib>:"Clear Errors.vi"("error in (no error)"=w1897) -> ("error out"=w1888:errorcluster)  [unwired: 5 in, 1 out]
        n1205 = call "Stall Data Flow.vim"("value in"=w1888, "milliseconds to wait"=u32 1000) -> ("value out"=w1895:errorcluster)  [unwired: 1 out]
        n1206 = call "Sway Init.vi"("error in (no error)"=w1895, "main ref"=w1889) -> ("error out"=w1890:errorcluster)  [unwired: 9 in]
        n1207 = call <vilib>:"Clear Errors.vi"("error in (no error)"=w1890) -> ("error out"=w1887:errorcluster)  [unwired: 5 in, 1 out]
        n1208 = call "SWAY READ FGV.vi"("Enum - Menu"=Sway_Right_enum."INIT", "error in (no error)"=w1887, "main ref"=w1889) -> ("error out"=w1893:errorcluster)  [unwired: 7 in, 1 out]
        n1209 = call <vilib>:"Clear Errors.vi"("error in (no error)"=w1893) -> ("error out"=w1892:errorcluster)  [unwired: 5 in, 1 out]
        n1210 = call-poly "Enqueue Message.vi"("error in (no error)"=w1892, "Message"="Sway Main", "Message Queue"=w1898) -> ("error out"=w1901:errorcluster)  [unwired: 7 in, 1 out]
      }
      frame "Sway Main" {
        n1211 = Unbundle By Name(w1902) -> ("Heave AND Surge.SURGE POSE"=w1913:refnum<vi>)
        n1212 = Unbundle By Name(w1902) -> ("SWAY.Read SWAY Temp"=w1922:refnum<vi>)
        n1213 = local read "HEAVE ENABLE"() -> (w1917:bool)
        n1214 = property class="DigNum (strict)"(reference=w1913) -> (reference out=w1915:refnum<vi>, error out=w1914:errorcluster, "Value"=w1912:sgl)  [unwired: 1 in]
        n1215 = property class="Bool (strict)"(reference=w1922) -> (reference out=w1920:refnum<vi>, error out=w1921:errorcluster, "Value"=w1919:bool)  [unwired: 1 in]
        n1216 = Equal?(x=w1917, y=TRUE) -> (x = y?=w1911:bool)
        n1217 = Close Reference(reference=w1915, error in (no error)=w1914) -> ()  [unwired: 1 out]
        n1218 = Equal?(x=w1912, y=sgl 25000.0) -> (x = y?=w1910:bool)
        n1219 = Close Reference(reference=w1920, error in (no error)=w1921) -> ()  [unwired: 1 out]
        n1220 = And(x=w1911, y=w1910) -> (x .and. y?=w1909:bool)
        n1221 = case shown="True" w1909 {
          tunnel: w1902 -> [_ w1934]
          tunnel: w1908 -> [w1929 w1933]
          tunnel: [w1929 w1930] -> w1906
          frame False {
          }
          frame True {
            n1222 = call "SWAY HOME.vi"("error in (no error)"=w1933, "Data Cluster"=w1934) -> ("error out"=w1931:errorcluster)  [unwired: 9 in]
            n1223 = local write "HEAVE ENABLE"(FALSE ("HEAVE ENABLE")) -> ()
            n1224 = call <vilib>:"Clear Errors.vi"("error in (no error)"=w1931) -> ("error out"=w1930:errorcluster)  [unwired: 5 in, 1 out]
          }
        }
        n1225 = case shown="True" w1919 {
          tunnel: w1908 -> [w1935 w1939]
          tunnel: [w1935 w1938] -> w1904
          tunnel: w1902 -> [_ w1937]
          frame False {
          }
          frame True {
            n1226 = call "SWAY READ FGV.vi"("Enum - Menu"=Sway_Right_enum."READ", "error in (no error)"=w1939, "main ref"=w1937) -> ("error out"=w1938:errorcluster)  [unwired: 7 in, 1 out]
          }
        }
        n1227 = call "Sway Reinitize.vi"("error in (no error)"=w1904, "Data Cluster"=w1902) -> ("error out"=w1903:errorcluster)  [unwired: 9 in]
        n1228 = Unbundle By Name(w1902) -> ("Main Home Screen.EXIT"=w1926:refnum<vi>)
        n1229 = property class="Bool (strict)"(reference=w1926) -> (reference out=w1924:refnum<vi>, error out=w1925:errorcluster, "Value"=w1923:bool)  [unwired: 1 in]
        n1230 = call <vilib>:"Clear Errors.vi"("error in (no error)"=w1903) -> ("error out"=w1918:errorcluster)  [unwired: 5 in, 1 out]
        n1231 = Merge Errors(w1918, w1906) -> (w1907:errorcluster)
        n1232 = Close Reference(reference=w1924, error in (no error)=w1925) -> ()  [unwired: 1 out]
        n1233 = case shown="False" w1923 {
          tunnel: [w1942 w1946] -> w1928
          tunnel: w1927 -> [w1941 w1945]
          tunnel: w1907 -> [w1940 w1944]
          frame True {
            n1234 = call-poly "Enqueue Message.vi"("error in (no error)"=w1940, "Message"="Confirm Quit", "Message Queue"=w1941) -> ("error out"=w1942:errorcluster)  [unwired: 7 in, 1 out]
          }
          frame False {
            n1235 = call-poly "Enqueue Message.vi"("error in (no error)"=w1944, "Message"="Sway Main", "Message Queue"=w1945) -> ("error out"=w1946:errorcluster)  [unwired: 7 in, 1 out]
          }
        }
      }
      frame "Error" {
        # "#CodeRecommended - If you ever change the name of this \"Error\" message, you'll need to update the name in the Check Loop Error.vi as well."
        # "#CodeRecommended - Consider creating a system for logging errors in some way. These errors are for notification purposes only. Handling of specific errors should be performed in the message frames that generated the error."
        # "Error - Display an error dialog. This message is sent by the \"Error Handler\" VIs at the end of other loops in this application."
        n1236 = Variant To Data(error in=w1954, type=errorcluster {"status"=FALSE, "code"=0, "source"=""} ("error constant"), Variant=w1952) -> (data=w1950:errorcluster, error out=w1949:errorcluster)
        n1237 = call <vilib>:"Simple Error Handler.vi"("error in (no error)"=w1950) -> ()  [unwired: 4 in, 5 out]
        n1238 = Merge Errors(w1949) -> (w1948:errorcluster)
      }
      frame "Confirm Quit" {
        # "#CodeNeeded - If you want to provide an \"Are you sure\" dialog (or some other notification) before the application exits, place that code here. This message is typically sent from a Panel Close? event."
        # "Confirm Quit - Message that can confirm whether or not the user wants to exit the application."
        n1239 = call-poly "Enqueue Message.vi"("Priority Message? (F)"=TRUE, "error in (no error)"=w1961, "Message"="Exit", "Message Queue"=w1957) -> ("error out"=w1958:errorcluster)  [unwired: 6 in, 1 out]
        n1240 = Merge Errors(w1958) -> (w1959:errorcluster)
      }
      frame "Exit" {
        # "Stop the VI"
        # "Release the message queue reference"
        # "#CodeNeeded - Add any required cleanup code here. Note that if 'Exit' was called as a result of an error, an error dialog will be displayed. Add any custom error handling for an 'Exit' condition here as well."
        # "Exit - Exit the application."
        n1241 = call "Fire User Event - Stop.vi"("User Event - Stop"=w1962) -> ("error out"=w1964:errorcluster)  [unwired: 10 in]
        n1242 = Release Queue(queue=w1969, error in (no error)=w1963) -> (error out=w1966:errorcluster)  [unwired: 1 in, 2 out]
        n1243 = Merge Errors(w1964, w1966) -> (w1965:errorcluster)
      }
      frame Default {
        # "'Default' case only runs if there is a message that isn't defined in any of the other cases.  Output a programming error."
        n1244 = xnode "Error Ring"("parameter 0"=w1970) -> ("error out"=w1971:errorcluster)
      }
    }
    n1245 = call "LAB-IQ Error Handler - Message Handling Loop.vi"("error in (no error)"=w1878, "Message Queue"=w1880) -> ("dup error in"=w1879:errorcluster)  [unwired: 8 in, 1 out]
  }
  n1246 = while {
    shift-right: [w1990] -> _
    shift-left: w14 -> [w1991]
    tunnel: [w1984] -> w19
    tunnel: w5 -> [w1982]
    tunnel: w4 -> [w1981]
    tunnel: w13 -> [w1980]
    stop <- w1989 stop-if-true
    # "Heave Motor  Handling Loop"
    n1247 = call "Dequeue Message.vi"("error in (no error)"=w1981, "Message Queue"=w1982) -> ("error out"=w1988:errorcluster, "Message Data"=w1986:variant, "Message"=w1987:string, "dup Message Queue"=w1985:refnum<queue>)  [unwired: 6 in]
    n1248 = case "Message Cases" shown="\"Heave Main\"" w1987 {
      selector: w1987 -> [_ _ _ _ _ w2062]
      tunnel: w1985 -> [w2004 w2019 _ w2050 w2061 _]
      tunnel: w1988 -> [w2001 w2017 w2040 w2053 w2055 _]
      tunnel: [w2002 w2020 w2034 w2041 w2057 w2063] -> w1983
      tunnel: w1991 -> [w2000 w2007 w2039 w2044 w2060 w2064]
      tunnel: [w2000 w2007 w2039 w2044 w2060 w2064] -> w1990
      tunnel: [_ _ _ _ TRUE _] -> w1989
      tunnel: w1986 -> [_ _ w2038 _ _ _]
      tunnel: w1980 -> [_ _ _ _ w2054 _]
      frame "init" {
        # "Initialize - All initialization work should take place in this message, since other loops can potentially enqueue messages that execute immediately after this one."
        n1249 = call "HEAVE WRITE FGV.vi"("Enum - Menu"=Heave_Write_enum."INIT", "error in (no error)"=w2001, "main ref"=w2000) -> ("error out"=w1999:errorcluster)  [unwired: 8 in]
        n1250 = call <vilib>:"Clear Errors.vi"("error in (no error)"=w1999) -> ("error out"=w1993:errorcluster)  [unwired: 5 in, 1 out]
        n1251 = call "Stall Data Flow.vim"("value in"=w1993, "milliseconds to wait"=u32 1000) -> ("value out"=w1997:errorcluster)  [unwired: 1 out]
        n1252 = call "Heave Init.vi"("error in (no error)"=w1997, "main ref"=w2000) -> ("error out"=w1994:errorcluster)  [unwired: 9 in]
        n1253 = call "HEAVE READ FGV.vi"("Enum - Menu"=Heave_Right_enum."INIT", "error in (no error)"=w1994, "main ref"=w2000) -> ("error out"=w1995:errorcluster)  [unwired: 7 in, 1 out]
        n1254 = call <vilib>:"Clear Errors.vi"("error in (no error)"=w1995) -> ("error out"=w2003:errorcluster)  [unwired: 5 in, 1 out]
        n1255 = call-poly "Enqueue Message.vi"("error in (no error)"=w2003, "Message"="Heave Main", "Message Queue"=w2004) -> ("error out"=w2002:errorcluster)  [unwired: 7 in, 1 out]
      }
      frame "Heave Main" {
        n1256 = Unbundle By Name(w2007) -> ("Heave AND Surge.Read Heave Temp"=w2013:refnum<vi>)
        n1257 = property class="Bool (strict)"(reference=w2013) -> (reference out=w2011:refnum<vi>, error out=w2012:errorcluster, "Value"=w2010:bool)  [unwired: 1 in]
        n1258 = Close Reference(reference=w2011, error in (no error)=w2012) -> ()  [unwired: 1 out]
        n1259 = case shown="True" w2010 {
          tunnel: w2017 -> [w2021 w2025]
          tunnel: [w2021 w2024] -> w2008
          tunnel: w2007 -> [_ w2023]
          frame False {
          }
          frame True {
            n1260 = call "HEAVE READ FGV.vi"("Enum - Menu"=Heave_Right_enum."READ", "error in (no error)"=w2025, "main ref"=w2023) -> ("error out"=w2024:errorcluster)  [unwired: 7 in, 1 out]
          }
        }
        n1261 = call "Heave Reinitial.vi"("error in (no error)"=w2008, "Data Cluster"=w2007) -> ("error out"=w2006:errorcluster)  [unwired: 9 in]
        n1262 = Unbundle By Name(w2007) -> ("Main Home Screen.EXIT"=w2018:refnum<vi>)
        n1263 = property class="Bool (strict)"(reference=w2018) -> (reference out=w2015:refnum<vi>, error out=w2016:errorcluster, "Value"=w2014:bool)  [unwired: 1 in]
        n1264 = call <vilib>:"Clear Errors.vi"("error in (no error)"=w2006) -> ("error out"=w2009:errorcluster)  [unwired: 5 in, 1 out]
        n1265 = Close Reference(reference=w2015, error in (no error)=w2016) -> ()  [unwired: 1 out]
        n1266 = case shown="False" w2014 {
          tunnel: [w2028 w2032] -> w2020
          tunnel: w2019 -> [w2027 w2031]
          tunnel: w2009 -> [w2026 w2030]
          frame True {
            n1267 = call-poly "Enqueue Message.vi"("error in (no error)"=w2026, "Message"="Confirm Quit", "Message Queue"=w2027) -> ("error out"=w2028:errorcluster)  [unwired: 7 in, 1 out]
          }
          frame False {
            n1268 = call-poly "Enqueue Message.vi"("error in (no error)"=w2030, "Message"="Heave Main", "Message Queue"=w2031) -> ("error out"=w2032:errorcluster)  [unwired: 7 in, 1 out]
          }
        }
      }
      frame "Error" {
        # "#CodeRecommended - If you ever change the name of this \"Error\" message, you'll need to update the name in the Check Loop Error.vi as well."
        # "#CodeRecommended - Consider creating a system for logging errors in some way. These errors are for notification purposes only. Handling of specific errors should be performed in the message frames that generated the error."
        # "Error - Display an error dialog. This message is sent by the \"Error Handler\" VIs at the end of other loops in this application."
        n1269 = Variant To Data(error in=w2040, type=errorcluster {"status"=FALSE, "code"=0, "source"=""} ("error constant"), Variant=w2038) -> (data=w2036:errorcluster, error out=w2035:errorcluster)
        n1270 = call <vilib>:"Simple Error Handler.vi"("error in (no error)"=w2036) -> ()  [unwired: 4 in, 5 out]
        n1271 = Merge Errors(w2035) -> (w2034:errorcluster)
      }
      frame "Confirm Quit" {
        # "#CodeNeeded - If you want to provide an \"Are you sure\" dialog (or some other notification) before the application exits, place that code here. This message is typically sent from a Panel Close? event."
        # "Confirm Quit - Message that can confirm whether or not the user wants to exit the application."
        n1272 = call-poly "Enqueue Message.vi"("Priority Message? (F)"=TRUE, "error in (no error)"=w2053, "Message"="Exit", "Message Queue"=w2050) -> ("error out"=w2051:errorcluster)  [unwired: 6 in, 1 out]
        n1273 = Merge Errors(w2051) -> (w2052:errorcluster)
        n1274 = call "HEAVE READ FGV.vi"("Enum - Menu"=Heave_Right_enum."CLOSE", "error in (no error)"=w2052, "main ref"=w2044) -> ("error out"=w2047:errorcluster)  [unwired: 7 in, 1 out]
        n1275 = call <vilib>:"Clear Errors.vi"("error in (no error)"=w2047) -> ("error out"=w2042:errorcluster)  [unwired: 5 in, 1 out]
        n1276 = call "HEAVE WRITE FGV.vi"("Enum - Menu"=Heave_Write_enum."CLOSE", "error in (no error)"=w2042, "main ref"=w2044) -> ("error out"=w2045:errorcluster)  [unwired: 8 in]
        n1277 = call <vilib>:"Clear Errors.vi"("error in (no error)"=w2045) -> ("error out"=w2041:errorcluster)  [unwired: 5 in, 1 out]
      }
      frame "Exit" {
        # "Stop the VI"
        # "Release the message queue reference"
        # "#CodeNeeded - Add any required cleanup code here. Note that if 'Exit' was called as a result of an error, an error dialog will be displayed. Add any custom error handling for an 'Exit' condition here as well."
        # "Exit - Exit the application."
        n1278 = call "Fire User Event - Stop.vi"("User Event - Stop"=w2054) -> ("error out"=w2056:errorcluster)  [unwired: 10 in]
        n1279 = Release Queue(queue=w2061, error in (no error)=w2055) -> (error out=w2058:errorcluster)  [unwired: 1 in, 2 out]
        n1280 = Merge Errors(w2056, w2058) -> (w2057:errorcluster)
      }
      frame Default {
        # "'Default' case only runs if there is a message that isn't defined in any of the other cases.  Output a programming error."
        n1281 = xnode "Error Ring"("parameter 0"=w2062) -> ("error out"=w2063:errorcluster)
      }
    }
    n1282 = call "LAB-IQ Error Handler - Message Handling Loop.vi"("error in (no error)"=w1983, "Message Queue"=w1985) -> ("dup error in"=w1984:errorcluster)  [unwired: 8 in, 1 out]
  }
  n1283 = while {
    shift-right: [w2082] -> _
    shift-left: w14 -> [w2083]
    tunnel: [w2076] -> w1
    tunnel: w20 -> [w2074]
    tunnel: w4 -> [w2073]
    tunnel: w13 -> [w2072]
    stop <- w2081 stop-if-true
    # "Temperature  Handling Loop"
    n1284 = call "Dequeue Message.vi"("error in (no error)"=w2073, "Message Queue"=w2074) -> ("error out"=w2080:errorcluster, "Message Data"=w2078:variant, "Message"=w2079:string, "dup Message Queue"=w2077:refnum<queue>)  [unwired: 6 in]
    n1285 = case "Message Cases" shown="\"Temperature Main\"" w2079 {
      selector: w2079 -> [_ _ _ _ _ w2127]
      tunnel: w2077 -> [w2084 w2095 _ w2114 w2126 _]
      tunnel: w2080 -> [w2087 w2092 w2111 w2118 w2120 _]
      tunnel: [w2088 w2096 w2105 w2116 w2122 w2128] -> w2075
      tunnel: w2083 -> [w2086 w2094 w2110 w2117 w2125 w2129]
      tunnel: [w2086 w2094 w2110 w2117 w2125 w2129] -> w2082
      tunnel: [_ _ _ _ TRUE _] -> w2081
      tunnel: w2078 -> [_ _ w2109 _ _ _]
      tunnel: w2072 -> [_ _ _ _ w2119 _]
      frame "init" {
        # "Initialize - All initialization work should take place in this message, since other loops can potentially enqueue messages that execute immediately after this one."
        n1286 = call-poly "Enqueue Message.vi"("error in (no error)"=w2087, "Message"="Temperature Main", "Message Queue"=w2084) -> ("error out"=w2088:errorcluster)  [unwired: 7 in, 1 out]
      }
      frame "Temperature Main" {
        n1287 = Unbundle By Name(w2094) -> ("Main Home Screen.EXIT"=w2093:refnum<vi>)
        n1288 = property class="Bool (strict)"(reference=w2093) -> (reference out=w2090:refnum<vi>, error out=w2091:errorcluster, "Value"=w2089:bool)  [unwired: 1 in]
        n1289 = case shown="False" w2089 {
          tunnel: [w2099 w2103] -> w2096
          tunnel: w2095 -> [w2098 w2102]
          tunnel: w2092 -> [w2097 w2101]
          frame True {
            n1290 = call-poly "Enqueue Message.vi"("error in (no error)"=w2097, "Message"="Confirm Quit", "Message Queue"=w2098) -> ("error out"=w2099:errorcluster)  [unwired: 7 in, 1 out]
          }
          frame False {
            n1291 = call-poly "Enqueue Message.vi"("error in (no error)"=w2101, "Message"="Temperature Main", "Message Queue"=w2102) -> ("error out"=w2103:errorcluster)  [unwired: 7 in, 1 out]
          }
        }
        n1292 = Close Reference(reference=w2090, error in (no error)=w2091) -> ()  [unwired: 1 out]
      }
      frame "Error" {
        # "#CodeRecommended - If you ever change the name of this \"Error\" message, you'll need to update the name in the Check Loop Error.vi as well."
        # "#CodeRecommended - Consider creating a system for logging errors in some way. These errors are for notification purposes only. Handling of specific errors should be performed in the message frames that generated the error."
        # "Error - Display an error dialog. This message is sent by the \"Error Handler\" VIs at the end of other loops in this application."
        n1293 = Variant To Data(error in=w2111, type=errorcluster {"status"=FALSE, "code"=0, "source"=""} ("error constant"), Variant=w2109) -> (data=w2107:errorcluster, error out=w2106:errorcluster)
        n1294 = call <vilib>:"Simple Error Handler.vi"("error in (no error)"=w2107) -> ()  [unwired: 4 in, 5 out]
        n1295 = Merge Errors(w2106) -> (w2105:errorcluster)
      }
      frame "Confirm Quit" {
        # "#CodeNeeded - If you want to provide an \"Are you sure\" dialog (or some other notification) before the application exits, place that code here. This message is typically sent from a Panel Close? event."
        # "Confirm Quit - Message that can confirm whether or not the user wants to exit the application."
        n1296 = call-poly "Enqueue Message.vi"("Priority Message? (F)"=TRUE, "error in (no error)"=w2118, "Message"="Exit", "Message Queue"=w2114) -> ("error out"=w2115:errorcluster)  [unwired: 6 in, 1 out]
        n1297 = Merge Errors(w2115) -> (w2116:errorcluster)
      }
      frame "Exit" {
        # "Stop the VI"
        # "Release the message queue reference"
        # "#CodeNeeded - Add any required cleanup code here. Note that if 'Exit' was called as a result of an error, an error dialog will be displayed. Add any custom error handling for an 'Exit' condition here as well."
        # "Exit - Exit the application."
        n1298 = call "Fire User Event - Stop.vi"("User Event - Stop"=w2119) -> ("error out"=w2121:errorcluster)  [unwired: 10 in]
        n1299 = Release Queue(queue=w2126, error in (no error)=w2120) -> (error out=w2123:errorcluster)  [unwired: 1 in, 2 out]
        n1300 = Merge Errors(w2121, w2123) -> (w2122:errorcluster)
      }
      frame Default {
        # "'Default' case only runs if there is a message that isn't defined in any of the other cases.  Output a programming error."
        n1301 = xnode "Error Ring"("parameter 0"=w2127) -> ("error out"=w2128:errorcluster)
      }
    }
    n1302 = call "LAB-IQ Error Handler - Message Handling Loop.vi"("error in (no error)"=w2075, "Message Queue"=w2077) -> ("dup error in"=w2076:errorcluster)  [unwired: 8 in, 1 out]
  }
  n1303 = while {
    shift-right: [w2147] -> _
    shift-left: w14 -> [w2148]
    tunnel: [w2141] -> _
    tunnel: w18 -> [w2139]
    tunnel: w4 -> [w2138]
    tunnel: w13 -> [w2137]
    stop <- w2146 stop-if-true
    # "Ramp Motor  Handling Loop"
    n1304 = call "Dequeue Message.vi"("error in (no error)"=w2138, "Message Queue"=w2139) -> ("error out"=w2145:errorcluster, "Message Data"=w2143:variant, "Message"=w2144:string, "dup Message Queue"=w2142:refnum<queue>)  [unwired: 6 in]
    n1305 = case "Message Cases" shown="\"Ramp Main\"" w2144 {
      selector: w2144 -> [_ _ _ _ _ w2192]
      tunnel: w2142 -> [w2149 w2160 _ w2179 w2191 _]
      tunnel: w2145 -> [w2152 w2157 w2176 w2183 w2185 _]
      tunnel: [w2153 w2161 w2170 w2181 w2187 w2193] -> w2140
      tunnel: w2148 -> [w2151 w2159 w2175 w2182 w2190 w2194]
      tunnel: [w2151 w2159 w2175 w2182 w2190 w2194] -> w2147
      tunnel: [_ _ _ _ TRUE _] -> w2146
      tunnel: w2143 -> [_ _ w2174 _ _ _]
      tunnel: w2137 -> [_ _ _ _ w2184 _]
      frame "init" {
        # "Initialize - All initialization work should take place in this message, since other loops can potentially enqueue messages that execute immediately after this one."
        n1306 = call-poly "Enqueue Message.vi"("error in (no error)"=w2152, "Message"="Ramp Main", "Message Queue"=w2149) -> ("error out"=w2153:errorcluster)  [unwired: 7 in, 1 out]
      }
      frame "Ramp Main" {
        n1307 = Unbundle By Name(w2159) -> ("Main Home Screen.EXIT"=w2158:refnum<vi>)
        n1308 = property class="Bool (strict)"(reference=w2158) -> (reference out=w2155:refnum<vi>, error out=w2156:errorcluster, "Value"=w2154:bool)  [unwired: 1 in]
        n1309 = case shown="False" w2154 {
          tunnel: [w2164 w2168] -> w2161
          tunnel: w2160 -> [w2163 w2167]
          tunnel: w2157 -> [w2162 w2166]
          frame True {
            n1310 = call-poly "Enqueue Message.vi"("error in (no error)"=w2162, "Message"="Confirm Quit", "Message Queue"=w2163) -> ("error out"=w2164:errorcluster)  [unwired: 7 in, 1 out]
          }
          frame False {
            n1311 = call-poly "Enqueue Message.vi"("error in (no error)"=w2166, "Message"="Ramp Main", "Message Queue"=w2167) -> ("error out"=w2168:errorcluster)  [unwired: 7 in, 1 out]
          }
        }
        n1312 = Close Reference(reference=w2155, error in (no error)=w2156) -> ()  [unwired: 1 out]
      }
      frame "Error" {
        # "#CodeRecommended - If you ever change the name of this \"Error\" message, you'll need to update the name in the Check Loop Error.vi as well."
        # "#CodeRecommended - Consider creating a system for logging errors in some way. These errors are for notification purposes only. Handling of specific errors should be performed in the message frames that generated the error."
        # "Error - Display an error dialog. This message is sent by the \"Error Handler\" VIs at the end of other loops in this application."
        n1313 = Variant To Data(error in=w2176, type=errorcluster {"status"=FALSE, "code"=0, "source"=""} ("error constant"), Variant=w2174) -> (data=w2172:errorcluster, error out=w2171:errorcluster)
        n1314 = call <vilib>:"Simple Error Handler.vi"("error in (no error)"=w2172) -> ()  [unwired: 4 in, 5 out]
        n1315 = Merge Errors(w2171) -> (w2170:errorcluster)
      }
      frame "Confirm Quit" {
        # "#CodeNeeded - If you want to provide an \"Are you sure\" dialog (or some other notification) before the application exits, place that code here. This message is typically sent from a Panel Close? event."
        # "Confirm Quit - Message that can confirm whether or not the user wants to exit the application."
        n1316 = call-poly "Enqueue Message.vi"("Priority Message? (F)"=TRUE, "error in (no error)"=w2183, "Message"="Exit", "Message Queue"=w2179) -> ("error out"=w2180:errorcluster)  [unwired: 6 in, 1 out]
        n1317 = Merge Errors(w2180) -> (w2181:errorcluster)
      }
      frame "Exit" {
        # "Stop the VI"
        # "Release the message queue reference"
        # "#CodeNeeded - Add any required cleanup code here. Note that if 'Exit' was called as a result of an error, an error dialog will be displayed. Add any custom error handling for an 'Exit' condition here as well."
        # "Exit - Exit the application."
        n1318 = call "Fire User Event - Stop.vi"("User Event - Stop"=w2184) -> ("error out"=w2186:errorcluster)  [unwired: 10 in]
        n1319 = Release Queue(queue=w2191, error in (no error)=w2185) -> (error out=w2188:errorcluster)  [unwired: 1 in, 2 out]
        n1320 = Merge Errors(w2186, w2188) -> (w2187:errorcluster)
      }
      frame Default {
        # "'Default' case only runs if there is a message that isn't defined in any of the other cases.  Output a programming error."
        n1321 = xnode "Error Ring"("parameter 0"=w2192) -> ("error out"=w2193:errorcluster)
      }
    }
    n1322 = call "LAB-IQ Error Handler - Message Handling Loop.vi"("error in (no error)"=w2140, "Message Queue"=w2142) -> ("dup error in"=w2141:errorcluster)  [unwired: 8 in, 1 out]
  }
  n1323 = while {
    shift-right: [w2212] -> _
    shift-left: w14 -> [w2213]
    tunnel: [w2206] -> _
    tunnel: w17 -> [w2204]
    tunnel: w4 -> [w2203]
    tunnel: w13 -> [w2202]
    stop <- w2211 stop-if-true
    # "ECR  Handling Loop"
    n1324 = call "Dequeue Message.vi"("error in (no error)"=w2203, "Message Queue"=w2204) -> ("error out"=w2210:errorcluster, "Message Data"=w2208:variant, "Message"=w2209:string, "dup Message Queue"=w2207:refnum<queue>)  [unwired: 6 in]
    n1325 = case "Message Cases" shown="\"ECR Main\"" w2209 {
      selector: w2209 -> [_ _ _ _ _ w2257]
      tunnel: w2207 -> [w2214 w2225 _ w2244 w2256 _]
      tunnel: w2210 -> [w2217 w2222 w2241 w2248 w2250 _]
      tunnel: [w2218 w2226 w2235 w2246 w2252 w2258] -> w2205
      tunnel: w2213 -> [w2216 w2224 w2240 w2247 w2255 w2259]
      tunnel: [w2216 w2224 w2240 w2247 w2255 w2259] -> w2212
      tunnel: [_ _ _ _ TRUE _] -> w2211
      tunnel: w2208 -> [_ _ w2239 _ _ _]
      tunnel: w2202 -> [_ _ _ _ w2249 _]
      frame "init" {
        # "Initialize - All initialization work should take place in this message, since other loops can potentially enqueue messages that execute immediately after this one."
        n1326 = call-poly "Enqueue Message.vi"("error in (no error)"=w2217, "Message"="ECR Main", "Message Queue"=w2214) -> ("error out"=w2218:errorcluster)  [unwired: 7 in, 1 out]
      }
      frame "ECR Main" {
        n1327 = Unbundle By Name(w2224) -> ("Main Home Screen.EXIT"=w2223:refnum<vi>)
        n1328 = property class="Bool (strict)"(reference=w2223) -> (reference out=w2220:refnum<vi>, error out=w2221:errorcluster, "Value"=w2219:bool)  [unwired: 1 in]
        n1329 = case shown="False" w2219 {
          tunnel: [w2229 w2233] -> w2226
          tunnel: w2225 -> [w2228 w2232]
          tunnel: w2222 -> [w2227 w2231]
          frame True {
            n1330 = call-poly "Enqueue Message.vi"("error in (no error)"=w2227, "Message"="Confirm Quit", "Message Queue"=w2228) -> ("error out"=w2229:errorcluster)  [unwired: 7 in, 1 out]
          }
          frame False {
            n1331 = call-poly "Enqueue Message.vi"("error in (no error)"=w2231, "Message"="ECR Main", "Message Queue"=w2232) -> ("error out"=w2233:errorcluster)  [unwired: 7 in, 1 out]
          }
        }
        n1332 = Close Reference(reference=w2220, error in (no error)=w2221) -> ()  [unwired: 1 out]
      }
      frame "Error" {
        # "#CodeRecommended - If you ever change the name of this \"Error\" message, you'll need to update the name in the Check Loop Error.vi as well."
        # "#CodeRecommended - Consider creating a system for logging errors in some way. These errors are for notification purposes only. Handling of specific errors should be performed in the message frames that generated the error."
        # "Error - Display an error dialog. This message is sent by the \"Error Handler\" VIs at the end of other loops in this application."
        n1333 = Variant To Data(error in=w2241, type=errorcluster {"status"=FALSE, "code"=0, "source"=""} ("error constant"), Variant=w2239) -> (data=w2237:errorcluster, error out=w2236:errorcluster)
        n1334 = call <vilib>:"Simple Error Handler.vi"("error in (no error)"=w2237) -> ()  [unwired: 4 in, 5 out]
        n1335 = Merge Errors(w2236) -> (w2235:errorcluster)
      }
      frame "Confirm Quit" {
        # "#CodeNeeded - If you want to provide an \"Are you sure\" dialog (or some other notification) before the application exits, place that code here. This message is typically sent from a Panel Close? event."
        # "Confirm Quit - Message that can confirm whether or not the user wants to exit the application."
        n1336 = call-poly "Enqueue Message.vi"("Priority Message? (F)"=TRUE, "error in (no error)"=w2248, "Message"="Exit", "Message Queue"=w2244) -> ("error out"=w2245:errorcluster)  [unwired: 6 in, 1 out]
        n1337 = Merge Errors(w2245) -> (w2246:errorcluster)
      }
      frame "Exit" {
        # "Stop the VI"
        # "Release the message queue reference"
        # "#CodeNeeded - Add any required cleanup code here. Note that if 'Exit' was called as a result of an error, an error dialog will be displayed. Add any custom error handling for an 'Exit' condition here as well."
        # "Exit - Exit the application."
        n1338 = call "Fire User Event - Stop.vi"("User Event - Stop"=w2249) -> ("error out"=w2251:errorcluster)  [unwired: 10 in]
        n1339 = Release Queue(queue=w2256, error in (no error)=w2250) -> (error out=w2253:errorcluster)  [unwired: 1 in, 2 out]
        n1340 = Merge Errors(w2251, w2253) -> (w2252:errorcluster)
      }
      frame Default {
        # "'Default' case only runs if there is a message that isn't defined in any of the other cases.  Output a programming error."
        n1341 = xnode "Error Ring"("parameter 0"=w2257) -> ("error out"=w2258:errorcluster)
      }
    }
    n1342 = call "LAB-IQ Error Handler - Message Handling Loop.vi"("error in (no error)"=w2205, "Message Queue"=w2207) -> ("dup error in"=w2206:errorcluster)  [unwired: 8 in, 1 out]
  }
  n1343 = while {
    shift-right: [w2277] -> _
    shift-left: w14 -> [w2278]
    tunnel: [w2271] -> _
    tunnel: w16 -> [w2269]
    tunnel: w4 -> [w2268]
    tunnel: w13 -> [w2267]
    stop <- w2276 stop-if-true
    # "Humidity  Handling Loop"
    n1344 = call "Dequeue Message.vi"("error in (no error)"=w2268, "Message Queue"=w2269) -> ("error out"=w2275:errorcluster, "Message Data"=w2273:variant, "Message"=w2274:string, "dup Message Queue"=w2272:refnum<queue>)  [unwired: 6 in]
    n1345 = case "Message Cases" shown="\"Humidity Main\"" w2274 {
      selector: w2274 -> [_ _ _ _ _ w2322]
      tunnel: w2272 -> [w2279 w2290 _ w2309 w2321 _]
      tunnel: w2275 -> [w2282 w2287 w2306 w2313 w2315 _]
      tunnel: [w2283 w2291 w2300 w2311 w2317 w2323] -> w2270
      tunnel: w2278 -> [w2281 w2289 w2305 w2312 w2320 w2324]
      tunnel: [w2281 w2289 w2305 w2312 w2320 w2324] -> w2277
      tunnel: [_ _ _ _ TRUE _] -> w2276
      tunnel: w2273 -> [_ _ w2304 _ _ _]
      tunnel: w2267 -> [_ _ _ _ w2314 _]
      frame "init" {
        # "Initialize - All initialization work should take place in this message, since other loops can potentially enqueue messages that execute immediately after this one."
        n1346 = call-poly "Enqueue Message.vi"("error in (no error)"=w2282, "Message"="Humidity Main", "Message Queue"=w2279) -> ("error out"=w2283:errorcluster)  [unwired: 7 in, 1 out]
      }
      frame "Humidity Main" {
        n1347 = Unbundle By Name(w2289) -> ("Main Home Screen.EXIT"=w2288:refnum<vi>)
        n1348 = property class="Bool (strict)"(reference=w2288) -> (reference out=w2285:refnum<vi>, error out=w2286:errorcluster, "Value"=w2284:bool)  [unwired: 1 in]
        n1349 = case shown="False" w2284 {
          tunnel: [w2294 w2298] -> w2291
          tunnel: w2290 -> [w2293 w2297]
          tunnel: w2287 -> [w2292 w2296]
          frame True {
            n1350 = call-poly "Enqueue Message.vi"("error in (no error)"=w2292, "Message"="Confirm Quit", "Message Queue"=w2293) -> ("error out"=w2294:errorcluster)  [unwired: 7 in, 1 out]
          }
          frame False {
            n1351 = call-poly "Enqueue Message.vi"("error in (no error)"=w2296, "Message"="Humidity Main", "Message Queue"=w2297) -> ("error out"=w2298:errorcluster)  [unwired: 7 in, 1 out]
          }
        }
        n1352 = Close Reference(reference=w2285, error in (no error)=w2286) -> ()  [unwired: 1 out]
      }
      frame "Error" {
        # "#CodeRecommended - If you ever change the name of this \"Error\" message, you'll need to update the name in the Check Loop Error.vi as well."
        # "#CodeRecommended - Consider creating a system for logging errors in some way. These errors are for notification purposes only. Handling of specific errors should be performed in the message frames that generated the error."
        # "Error - Display an error dialog. This message is sent by the \"Error Handler\" VIs at the end of other loops in this application."
        n1353 = Variant To Data(error in=w2306, type=errorcluster {"status"=FALSE, "code"=0, "source"=""} ("error constant"), Variant=w2304) -> (data=w2302:errorcluster, error out=w2301:errorcluster)
        n1354 = call <vilib>:"Simple Error Handler.vi"("error in (no error)"=w2302) -> ()  [unwired: 4 in, 5 out]
        n1355 = Merge Errors(w2301) -> (w2300:errorcluster)
      }
      frame "Confirm Quit" {
        # "#CodeNeeded - If you want to provide an \"Are you sure\" dialog (or some other notification) before the application exits, place that code here. This message is typically sent from a Panel Close? event."
        # "Confirm Quit - Message that can confirm whether or not the user wants to exit the application."
        n1356 = call-poly "Enqueue Message.vi"("Priority Message? (F)"=TRUE, "error in (no error)"=w2313, "Message"="Exit", "Message Queue"=w2309) -> ("error out"=w2310:errorcluster)  [unwired: 6 in, 1 out]
        n1357 = Merge Errors(w2310) -> (w2311:errorcluster)
      }
      frame "Exit" {
        # "Stop the VI"
        # "Release the message queue reference"
        # "#CodeNeeded - Add any required cleanup code here. Note that if 'Exit' was called as a result of an error, an error dialog will be displayed. Add any custom error handling for an 'Exit' condition here as well."
        # "Exit - Exit the application."
        n1358 = call "Fire User Event - Stop.vi"("User Event - Stop"=w2314) -> ("error out"=w2316:errorcluster)  [unwired: 10 in]
        n1359 = Release Queue(queue=w2321, error in (no error)=w2315) -> (error out=w2318:errorcluster)  [unwired: 1 in, 2 out]
        n1360 = Merge Errors(w2316, w2318) -> (w2317:errorcluster)
      }
      frame Default {
        # "'Default' case only runs if there is a message that isn't defined in any of the other cases.  Output a programming error."
        n1361 = xnode "Error Ring"("parameter 0"=w2322) -> ("error out"=w2323:errorcluster)
      }
    }
    n1362 = call "LAB-IQ Error Handler - Message Handling Loop.vi"("error in (no error)"=w2270, "Message Queue"=w2272) -> ("dup error in"=w2271:errorcluster)  [unwired: 8 in, 1 out]
  }
  n1363 = while {
    shift-right: [w2342] -> _
    shift-left: w14 -> [w2343]
    tunnel: [w2336] -> _
    tunnel: w15 -> [w2334]
    tunnel: w4 -> [w2333]
    tunnel: w13 -> [w2332]
    stop <- w2341 stop-if-true
    # "Program  Handling Loop"
    n1364 = call "Dequeue Message.vi"("error in (no error)"=w2333, "Message Queue"=w2334) -> ("error out"=w2340:errorcluster, "Message Data"=w2338:variant, "Message"=w2339:string, "dup Message Queue"=w2337:refnum<queue>)  [unwired: 6 in]
    n1365 = case "Message Cases" shown="\"Program Main\"" w2339 {
      selector: w2339 -> [_ _ _ _ _ w2388]
      tunnel: w2337 -> [w2344 w2356 _ w2375 w2387 _]
      tunnel: w2340 -> [w2347 w2350 w2372 w2379 w2381 _]
      tunnel: [w2348 w2357 w2366 w2377 w2383 w2389] -> w2335
      tunnel: w2343 -> [w2346 w2349 w2371 w2378 w2386 w2390]
      tunnel: [w2346 w2349 w2371 w2378 w2386 w2390] -> w2342
      tunnel: [_ _ _ _ TRUE _] -> w2341
      tunnel: w2338 -> [_ _ w2370 _ _ _]
      tunnel: w2332 -> [_ _ _ _ w2380 _]
      frame "init" {
        # "Initialize - All initialization work should take place in this message, since other loops can potentially enqueue messages that execute immediately after this one."
        n1366 = call-poly "Enqueue Message.vi"("error in (no error)"=w2347, "Message"="Program Main", "Message Queue"=w2344) -> ("error out"=w2348:errorcluster)  [unwired: 7 in, 1 out]
      }
      frame "Program Main" {
        n1367 = call "Main Program Loop Vi.vi"("error in (no error)"=w2350, "Data Cluster"=w2349) -> ("error out"=w2351:errorcluster)  [unwired: 9 in]
        n1368 = Unbundle By Name(w2349) -> ("Main Home Screen.EXIT"=w2355:refnum<vi>)
        n1369 = property class="Bool (strict)"(reference=w2355) -> (reference out=w2353:refnum<vi>, error out=w2354:errorcluster, "Value"=w2352:bool)  [unwired: 1 in]
        n1370 = case shown="False" w2352 {
          tunnel: [w2360 w2364] -> w2357
          tunnel: w2356 -> [w2359 w2363]
          tunnel: w2351 -> [w2358 w2362]
          frame True {
            n1371 = call-poly "Enqueue Message.vi"("error in (no error)"=w2358, "Message"="Confirm Quit", "Message Queue"=w2359) -> ("error out"=w2360:errorcluster)  [unwired: 7 in, 1 out]
          }
          frame False {
            n1372 = call-poly "Enqueue Message.vi"("error in (no error)"=w2362, "Message"="Program Main", "Message Queue"=w2363) -> ("error out"=w2364:errorcluster)  [unwired: 7 in, 1 out]
          }
        }
        n1373 = Close Reference(reference=w2353, error in (no error)=w2354) -> ()  [unwired: 1 out]
      }
      frame "Error" {
        # "#CodeRecommended - If you ever change the name of this \"Error\" message, you'll need to update the name in the Check Loop Error.vi as well."
        # "#CodeRecommended - Consider creating a system for logging errors in some way. These errors are for notification purposes only. Handling of specific errors should be performed in the message frames that generated the error."
        # "Error - Display an error dialog. This message is sent by the \"Error Handler\" VIs at the end of other loops in this application."
        n1374 = Variant To Data(error in=w2372, type=errorcluster {"status"=FALSE, "code"=0, "source"=""} ("error constant"), Variant=w2370) -> (data=w2368:errorcluster, error out=w2367:errorcluster)
        n1375 = call <vilib>:"Simple Error Handler.vi"("error in (no error)"=w2368) -> ()  [unwired: 4 in, 5 out]
        n1376 = Merge Errors(w2367) -> (w2366:errorcluster)
      }
      frame "Confirm Quit" {
        # "#CodeNeeded - If you want to provide an \"Are you sure\" dialog (or some other notification) before the application exits, place that code here. This message is typically sent from a Panel Close? event."
        # "Confirm Quit - Message that can confirm whether or not the user wants to exit the application."
        n1377 = call-poly "Enqueue Message.vi"("Priority Message? (F)"=TRUE, "error in (no error)"=w2379, "Message"="Exit", "Message Queue"=w2375) -> ("error out"=w2376:errorcluster)  [unwired: 6 in, 1 out]
        n1378 = Merge Errors(w2376) -> (w2377:errorcluster)
      }
      frame "Exit" {
        # "Stop the VI"
        # "Release the message queue reference"
        # "#CodeNeeded - Add any required cleanup code here. Note that if 'Exit' was called as a result of an error, an error dialog will be displayed. Add any custom error handling for an 'Exit' condition here as well."
        # "Exit - Exit the application."
        n1379 = call "Fire User Event - Stop.vi"("User Event - Stop"=w2380) -> ("error out"=w2382:errorcluster)  [unwired: 10 in]
        n1380 = Release Queue(queue=w2387, error in (no error)=w2381) -> (error out=w2384:errorcluster)  [unwired: 1 in, 2 out]
        n1381 = Merge Errors(w2382, w2384) -> (w2383:errorcluster)
      }
      frame Default {
        # "'Default' case only runs if there is a message that isn't defined in any of the other cases.  Output a programming error."
        n1382 = xnode "Error Ring"("parameter 0"=w2388) -> ("error out"=w2389:errorcluster)
      }
    }
    n1383 = call "LAB-IQ Error Handler - Message Handling Loop.vi"("error in (no error)"=w2335, "Message Queue"=w2337) -> ("dup error in"=w2336:errorcluster)  [unwired: 8 in, 1 out]
  }
  n1384 = while {
    shift-right: [w2408] -> _
    shift-left: w14 -> [w2409]
    tunnel: [w2402] -> _
    tunnel: w12 -> [w2400]
    tunnel: w4 -> [w2399]
    tunnel: w13 -> [w2398]
    stop <- w2407 stop-if-true
    # "Monitor  Handling Loop"
    n1385 = call "Dequeue Message.vi"("error in (no error)"=w2399, "Message Queue"=w2400) -> ("error out"=w2406:errorcluster, "Message Data"=w2404:variant, "Message"=w2405:string, "dup Message Queue"=w2403:refnum<queue>)  [unwired: 6 in]
    n1386 = case "Message Cases" shown="\"Monitor Main\"" w2405 {
      selector: w2405 -> [_ _ _ _ _ w2454]
      tunnel: w2403 -> [w2410 w2422 _ w2441 w2453 _]
      tunnel: w2406 -> [w2413 w2416 w2438 w2445 w2447 _]
      tunnel: [w2414 w2423 w2432 w2443 w2449 w2455] -> w2401
      tunnel: w2409 -> [w2412 w2415 w2437 w2444 w2452 w2456]
      tunnel: [w2412 w2415 w2437 w2444 w2452 w2456] -> w2408
      tunnel: [_ _ _ _ TRUE _] -> w2407
      tunnel: w2404 -> [_ _ w2436 _ _ _]
      tunnel: w2398 -> [_ _ _ _ w2446 _]
      frame "init" {
        # "Initialize - All initialization work should take place in this message, since other loops can potentially enqueue messages that execute immediately after this one."
        n1387 = call-poly "Enqueue Message.vi"("error in (no error)"=w2413, "Message"="Monitor Main", "Message Queue"=w2410) -> ("error out"=w2414:errorcluster)  [unwired: 7 in, 1 out]
      }
      frame "Monitor Main" {
        n1388 = call "Main Monitor Loop.vi"("error in (no error)"=w2416, "main ref"=w2415) -> ("error out"=w2417:errorcluster)  [unwired: 9 in]
        n1389 = call "LOAD SELECTION MAIN CODE.vi"("error in (no error)"=w2416, "main ref"=w2415) -> ()  [unwired: 9 in, 1 out]
        n1390 = Unbundle By Name(w2415) -> ("Main Home Screen.EXIT"=w2421:refnum<vi>)
        n1391 = property class="Bool (strict)"(reference=w2421) -> (reference out=w2419:refnum<vi>, error out=w2420:errorcluster, "Value"=w2418:bool)  [unwired: 1 in]
        n1392 = case shown="False" w2418 {
          tunnel: [w2426 w2430] -> w2423
          tunnel: w2422 -> [w2425 w2429]
          tunnel: w2417 -> [w2424 w2428]
          frame True {
            n1393 = call-poly "Enqueue Message.vi"("error in (no error)"=w2424, "Message"="Confirm Quit", "Message Queue"=w2425) -> ("error out"=w2426:errorcluster)  [unwired: 7 in, 1 out]
          }
          frame False {
            n1394 = call-poly "Enqueue Message.vi"("error in (no error)"=w2428, "Message"="Monitor Main", "Message Queue"=w2429) -> ("error out"=w2430:errorcluster)  [unwired: 7 in, 1 out]
          }
        }
        n1395 = Close Reference(reference=w2419, error in (no error)=w2420) -> ()  [unwired: 1 out]
      }
      frame "Error" {
        # "#CodeRecommended - If you ever change the name of this \"Error\" message, you'll need to update the name in the Check Loop Error.vi as well."
        # "#CodeRecommended - Consider creating a system for logging errors in some way. These errors are for notification purposes only. Handling of specific errors should be performed in the message frames that generated the error."
        # "Error - Display an error dialog. This message is sent by the \"Error Handler\" VIs at the end of other loops in this application."
        n1396 = Variant To Data(error in=w2438, type=errorcluster {"status"=FALSE, "code"=0, "source"=""} ("error constant"), Variant=w2436) -> (data=w2434:errorcluster, error out=w2433:errorcluster)
        n1397 = call <vilib>:"Simple Error Handler.vi"("error in (no error)"=w2434) -> ()  [unwired: 4 in, 5 out]
        n1398 = Merge Errors(w2433) -> (w2432:errorcluster)
      }
      frame "Confirm Quit" {
        # "#CodeNeeded - If you want to provide an \"Are you sure\" dialog (or some other notification) before the application exits, place that code here. This message is typically sent from a Panel Close? event."
        # "Confirm Quit - Message that can confirm whether or not the user wants to exit the application."
        n1399 = call-poly "Enqueue Message.vi"("Priority Message? (F)"=TRUE, "error in (no error)"=w2445, "Message"="Exit", "Message Queue"=w2441) -> ("error out"=w2442:errorcluster)  [unwired: 6 in, 1 out]
        n1400 = Merge Errors(w2442) -> (w2443:errorcluster)
      }
      frame "Exit" {
        # "Stop the VI"
        # "Release the message queue reference"
        # "#CodeNeeded - Add any required cleanup code here. Note that if 'Exit' was called as a result of an error, an error dialog will be displayed. Add any custom error handling for an 'Exit' condition here as well."
        # "Exit - Exit the application."
        n1401 = call "Fire User Event - Stop.vi"("User Event - Stop"=w2446) -> ("error out"=w2448:errorcluster)  [unwired: 10 in]
        n1402 = Release Queue(queue=w2453, error in (no error)=w2447) -> (error out=w2450:errorcluster)  [unwired: 1 in, 2 out]
        n1403 = Merge Errors(w2448, w2450) -> (w2449:errorcluster)
      }
      frame Default {
        # "'Default' case only runs if there is a message that isn't defined in any of the other cases.  Output a programming error."
        n1404 = xnode "Error Ring"("parameter 0"=w2454) -> ("error out"=w2455:errorcluster)
      }
    }
    n1405 = call "LAB-IQ Error Handler - Message Handling Loop.vi"("error in (no error)"=w2401, "Message Queue"=w2403) -> ("dup error in"=w2402:errorcluster)  [unwired: 8 in, 1 out]
  }
  n1406 = while {
    shift-right: [w2474] -> _
    shift-left: w14 -> [w2475]
    tunnel: [w2468] -> _
    tunnel: w11 -> [w2466]
    tunnel: w4 -> [w2465]
    tunnel: w13 -> [w2464]
    stop <- w2473 stop-if-true
    # "Load Pid  Handling Loop"
    n1407 = call "Dequeue Message.vi"("error in (no error)"=w2465, "Message Queue"=w2466) -> ("error out"=w2472:errorcluster, "Message Data"=w2470:variant, "Message"=w2471:string, "dup Message Queue"=w2469:refnum<queue>)  [unwired: 6 in]
    n1408 = case "Message Cases" shown="\"Load Pid Main\"" w2471 {
      selector: w2471 -> [_ _ _ _ _ w2540]
      tunnel: w2469 -> [w2476 w2497 _ w2527 w2539 _]
      tunnel: w2472 -> [w2479 w2495 w2524 w2531 w2533 _]
      tunnel: [w2480 w2498 w2518 w2529 w2535 w2541] -> w2467
      tunnel: w2475 -> [w2478 w2484 w2523 w2530 w2538 w2542]
      tunnel: [w2478 w2484 w2523 w2530 w2538 w2542] -> w2474
      tunnel: [_ _ _ _ TRUE _] -> w2473
      tunnel: w2470 -> [_ _ w2522 _ _ _]
      tunnel: w2464 -> [_ _ _ _ w2532 _]
      frame "init" {
        # "Initialize - All initialization work should take place in this message, since other loops can potentially enqueue messages that execute immediately after this one."
        n1409 = call-poly "Enqueue Message.vi"("error in (no error)"=w2479, "Message"="Load Pid Main", "Message Queue"=w2476) -> ("error out"=w2480:errorcluster)  [unwired: 7 in, 1 out]
      }
      frame "Load Pid Main" {
        n1410 = Unbundle By Name(w2484) -> ("Main Screen.Load En"=w2490:refnum<vi>)
        n1411 = Unbundle By Name(w2484) -> ("PID.apply load"=w2485:refnum<vi>)
        n1412 = property class="Bool (strict)"(reference=w2490) -> (reference out=w2488:refnum<vi>, error out=w2489:errorcluster, "Value"=w2483:bool)  [unwired: 1 in]
        n1413 = property class="Bool (strict)"(reference=w2485) -> (reference out=w2487:refnum<vi>, error out=w2486:errorcluster, "Value"=w2482:bool)  [unwired: 1 in]
        n1414 = Close Reference(reference=w2488, error in (no error)=w2489) -> ()  [unwired: 1 out]
        n1415 = Close Reference(reference=w2487, error in (no error)=w2486) -> ()  [unwired: 1 out]
        n1416 = Or(x=w2483, y=w2482) -> (x .or. y?=w2481:bool)
        n1417 = case shown="True" w2481 {
          tunnel: w2495 -> [w2499 w2502]
          tunnel: [w2499 w2501] -> w2491
          tunnel: w2484 -> [_ w2500]
          frame False {
          }
          frame True {
            n1418 = disable-structure shown="Enabled" {
              disable-tunnel: w2502 -> [w2505 w2509]
              disable-tunnel: [w2504 w2508] -> w2501
              disable-tunnel: w2500 -> [w2503 w2507]
              frame Disabled {
                n1419 = call "load pid.vi"("error in (no error)"=w2505, "main ref"=w2503) -> ("error out"=w2504:errorcluster)  [unwired: 9 in]
              }
              frame Enabled {
                n1420 = call "NEW LOAD CELL PID.vi"("error in (no error)"=w2509, "Checkbox"=TRUE, "main ref"=w2507) -> ("error out"=w2508:errorcluster)  [unwired: 8 in]
              }
            }
          }
        }
        n1421 = Unbundle By Name(w2484) -> ("Main Home Screen.EXIT"=w2496:refnum<vi>)
        n1422 = property class="Bool (strict)"(reference=w2496) -> (reference out=w2493:refnum<vi>, error out=w2494:errorcluster, "Value"=w2492:bool)  [unwired: 1 in]
        n1423 = case shown="False" w2492 {
          tunnel: [w2512 w2516] -> w2498
          tunnel: w2497 -> [w2511 w2515]
          tunnel: w2491 -> [w2510 w2514]
          frame True {
            n1424 = call-poly "Enqueue Message.vi"("error in (no error)"=w2510, "Message"="Confirm Quit", "Message Queue"=w2511) -> ("error out"=w2512:errorcluster)  [unwired: 7 in, 1 out]
          }
          frame False {
            n1425 = call-poly "Enqueue Message.vi"("error in (no error)"=w2514, "Message"="Load Pid Main", "Message Queue"=w2515) -> ("error out"=w2516:errorcluster)  [unwired: 7 in, 1 out]
          }
        }
        n1426 = Close Reference(reference=w2493, error in (no error)=w2494) -> ()  [unwired: 1 out]
      }
      frame "Error" {
        # "#CodeRecommended - If you ever change the name of this \"Error\" message, you'll need to update the name in the Check Loop Error.vi as well."
        # "#CodeRecommended - Consider creating a system for logging errors in some way. These errors are for notification purposes only. Handling of specific errors should be performed in the message frames that generated the error."
        # "Error - Display an error dialog. This message is sent by the \"Error Handler\" VIs at the end of other loops in this application."
        n1427 = Variant To Data(error in=w2524, type=errorcluster {"status"=FALSE, "code"=0, "source"=""} ("error constant"), Variant=w2522) -> (data=w2520:errorcluster, error out=w2519:errorcluster)
        n1428 = call <vilib>:"Simple Error Handler.vi"("error in (no error)"=w2520) -> ()  [unwired: 4 in, 5 out]
        n1429 = Merge Errors(w2519) -> (w2518:errorcluster)
      }
      frame "Confirm Quit" {
        # "#CodeNeeded - If you want to provide an \"Are you sure\" dialog (or some other notification) before the application exits, place that code here. This message is typically sent from a Panel Close? event."
        # "Confirm Quit - Message that can confirm whether or not the user wants to exit the application."
        n1430 = call-poly "Enqueue Message.vi"("Priority Message? (F)"=TRUE, "error in (no error)"=w2531, "Message"="Exit", "Message Queue"=w2527) -> ("error out"=w2528:errorcluster)  [unwired: 6 in, 1 out]
        n1431 = Merge Errors(w2528) -> (w2529:errorcluster)
      }
      frame "Exit" {
        # "Stop the VI"
        # "Release the message queue reference"
        # "#CodeNeeded - Add any required cleanup code here. Note that if 'Exit' was called as a result of an error, an error dialog will be displayed. Add any custom error handling for an 'Exit' condition here as well."
        # "Exit - Exit the application."
        n1432 = call "Fire User Event - Stop.vi"("User Event - Stop"=w2532) -> ("error out"=w2534:errorcluster)  [unwired: 10 in]
        n1433 = Release Queue(queue=w2539, error in (no error)=w2533) -> (error out=w2536:errorcluster)  [unwired: 1 in, 2 out]
        n1434 = Merge Errors(w2534, w2536) -> (w2535:errorcluster)
      }
      frame Default {
        # "'Default' case only runs if there is a message that isn't defined in any of the other cases.  Output a programming error."
        n1435 = xnode "Error Ring"("parameter 0"=w2540) -> ("error out"=w2541:errorcluster)
      }
    }
    n1436 = call "LAB-IQ Error Handler - Message Handling Loop.vi"("error in (no error)"=w2467, "Message Queue"=w2469) -> ("dup error in"=w2468:errorcluster)  [unwired: 8 in, 1 out]
  }
  n1437 = while {
    shift-right: [w2560] -> _
    shift-left: w14 -> [w2561]
    tunnel: [w2554] -> _
    tunnel: w10 -> [w2552]
    tunnel: w4 -> [w2551]
    tunnel: w13 -> [w2550]
    stop <- w2559 stop-if-true
    # "Report  Handling Loop"
    n1438 = call "Dequeue Message.vi"("error in (no error)"=w2551, "Message Queue"=w2552) -> ("error out"=w2558:errorcluster, "Message Data"=w2556:variant, "Message"=w2557:string, "dup Message Queue"=w2555:refnum<queue>)  [unwired: 6 in]
    n1439 = case "Message Cases" shown="\"Report Main\"" w2557 {
      selector: w2557 -> [_ _ _ _ _ w2606]
      tunnel: w2555 -> [w2562 w2574 _ w2593 w2605 _]
      tunnel: w2558 -> [w2565 w2572 w2590 w2597 w2599 _]
      tunnel: [w2566 w2575 w2584 w2595 w2601 w2607] -> w2553
      tunnel: w2561 -> [w2564 w2567 w2589 w2596 w2604 w2608]
      tunnel: [w2564 w2567 w2589 w2596 w2604 w2608] -> w2560
      tunnel: [_ _ _ _ TRUE _] -> w2559
      tunnel: w2556 -> [_ _ w2588 _ _ _]
      tunnel: w2550 -> [_ _ _ _ w2598 _]
      frame "init" {
        # "Initialize - All initialization work should take place in this message, since other loops can potentially enqueue messages that execute immediately after this one."
        n1440 = call-poly "Enqueue Message.vi"("error in (no error)"=w2565, "Message"="Report Main", "Message Queue"=w2562) -> ("error out"=w2566:errorcluster)  [unwired: 7 in, 1 out]
      }
      frame "Report Main" {
        n1441 = call "Main Data Log.vi"("error in (no error)"=w2572, "main ref"=w2567) -> ("error out"=w2568:errorcluster)  [unwired: 9 in]
        n1442 = Unbundle By Name(w2567) -> ("Main Home Screen.EXIT"=w2573:refnum<vi>)
        n1443 = property class="Bool (strict)"(reference=w2573) -> (reference out=w2570:refnum<vi>, error out=w2571:errorcluster, "Value"=w2569:bool)  [unwired: 1 in]
        n1444 = case shown="False" w2569 {
          tunnel: [w2578 w2582] -> w2575
          tunnel: w2574 -> [w2577 w2581]
          tunnel: w2568 -> [w2576 w2580]
          frame True {
            n1445 = call-poly "Enqueue Message.vi"("error in (no error)"=w2576, "Message"="Confirm Quit", "Message Queue"=w2577) -> ("error out"=w2578:errorcluster)  [unwired: 7 in, 1 out]
          }
          frame False {
            n1446 = call-poly "Enqueue Message.vi"("error in (no error)"=w2580, "Message"="Report Main", "Message Queue"=w2581) -> ("error out"=w2582:errorcluster)  [unwired: 7 in, 1 out]
          }
        }
        n1447 = Close Reference(reference=w2570, error in (no error)=w2571) -> ()  [unwired: 1 out]
      }
      frame "Error" {
        # "#CodeRecommended - If you ever change the name of this \"Error\" message, you'll need to update the name in the Check Loop Error.vi as well."
        # "#CodeRecommended - Consider creating a system for logging errors in some way. These errors are for notification purposes only. Handling of specific errors should be performed in the message frames that generated the error."
        # "Error - Display an error dialog. This message is sent by the \"Error Handler\" VIs at the end of other loops in this application."
        n1448 = Variant To Data(error in=w2590, type=errorcluster {"status"=FALSE, "code"=0, "source"=""} ("error constant"), Variant=w2588) -> (data=w2586:errorcluster, error out=w2585:errorcluster)
        n1449 = call <vilib>:"Simple Error Handler.vi"("error in (no error)"=w2586) -> ()  [unwired: 4 in, 5 out]
        n1450 = Merge Errors(w2585) -> (w2584:errorcluster)
      }
      frame "Confirm Quit" {
        # "#CodeNeeded - If you want to provide an \"Are you sure\" dialog (or some other notification) before the application exits, place that code here. This message is typically sent from a Panel Close? event."
        # "Confirm Quit - Message that can confirm whether or not the user wants to exit the application."
        n1451 = call-poly "Enqueue Message.vi"("Priority Message? (F)"=TRUE, "error in (no error)"=w2597, "Message"="Exit", "Message Queue"=w2593) -> ("error out"=w2594:errorcluster)  [unwired: 6 in, 1 out]
        n1452 = Merge Errors(w2594) -> (w2595:errorcluster)
      }
      frame "Exit" {
        # "Stop the VI"
        # "Release the message queue reference"
        # "#CodeNeeded - Add any required cleanup code here. Note that if 'Exit' was called as a result of an error, an error dialog will be displayed. Add any custom error handling for an 'Exit' condition here as well."
        # "Exit - Exit the application."
        n1453 = call "Fire User Event - Stop.vi"("User Event - Stop"=w2598) -> ("error out"=w2600:errorcluster)  [unwired: 10 in]
        n1454 = Release Queue(queue=w2605, error in (no error)=w2599) -> (error out=w2602:errorcluster)  [unwired: 1 in, 2 out]
        n1455 = Merge Errors(w2600, w2602) -> (w2601:errorcluster)
      }
      frame Default {
        # "'Default' case only runs if there is a message that isn't defined in any of the other cases.  Output a programming error."
        n1456 = xnode "Error Ring"("parameter 0"=w2606) -> ("error out"=w2607:errorcluster)
      }
    }
    n1457 = call "LAB-IQ Error Handler - Message Handling Loop.vi"("error in (no error)"=w2553, "Message Queue"=w2555) -> ("dup error in"=w2554:errorcluster)  [unwired: 8 in, 1 out]
  }
  n1458 = Unregister For Events(event registration refnum=w48, error in=w46) -> (error out=w49:errorcluster)
  n1459 = Merge Errors(w49, w52, w24, w21, w19, w1) -> (w50:errorcluster)
  n1460 = call "Destroy User Event - Stop.vi"("error in (no error)"=w50, "User Event - Stop"=w13) -> ("error out"=w47:errorcluster)  [unwired: 9 in]
  n1461 = disable-structure shown="RUN_TIME_ENGINE==True" {
    disable-tunnel: w47 -> [_ _]
    frame condition #0 (active) {
    }
    frame condition #1 {
      # "Call Quit LabVIEW if running as a built application."
      n1462 = Quit LabVIEW() -> ()  [unwired: 1 in]
    }
  }
